vi "Measurement UI.vi"() -> ()   [LabVIEW 2024, in "Device Power Sequencer UI.lvlib"]
doc: "This module lets user configure a sequence to power up or power down any device. \n\nThe various configuration operations allowed are:\n1. Add Pin - Add a pin to the sequence\n2.Delete Pin - Delete a pin from the sequence\n3.Move Pin Up - Move the selected pin a level up in the sequence\n4.Move Pin Down - Move the selected pin a level down in the sequence\n5.Edit Pin - Change pin mapping and edit the configuration paramters.\n\nThe results displayed after sequence execution are:\n1. Voltage Waveform - Displays voltage graph for each pin\n2.Current Waveform - Displays current graph for each pin"
uses:
  Device Power Sequencer UI.lvlib
  Device Power Sequencer/controls/Source Pin Config.ctl
  Device Power Sequencer/controls/Source Mode.ctl
  Device Power Sequencer/controls/UI_Relative To.ctl
  Device Power Sequencer/controls/Sense Mode.ctl
  Device Power Sequencer/controls/Transient Response.ctl
  Device Power Sequencer/controls/Relative To.ctl
  Device Power Sequencer/controls/Plot Colors.ctl
  Device Power Sequencer/controls/Empty Plot Legend.ctl
  Device Power Sequencer/controls/Power line frequency.ctl
  Device Power Sequencer/controls/Plot Legend.ctl
  Device Power Sequencer/controls/Plot Cluster.ctl
  Device Power Sequencer/Device Power Sequencer.lvlib
panel:
  in  "Monitor":bool
  out "Pin Readbacks":string="      Pin readbacks"
  in  "Legend":T1
  in  "Empty Legend":T2={"Free label"="", "Header"="  Plot visibility", "Msg"="  No active channels"}
  out "Voltage":waveform(dbl)[](graph) caption="Voltage Measurements"
  out "Current":waveform(dbl)[](graph) caption="Current Measurements"
  in  "PD-Image":bool
  in  "Power Down Info":bool
  in  "Power Down":bool caption="Quick Power Down"
  out "Power Up/Down":bool
  in  "R-Image":bool
  in  "Pin Selection":i32(listbox)
  in  "Hover icon":bool
  in  "Selection icon":bool
  in  "Source Pin Seq":i32(listbox)
  out "Border":string
  in  "Move Down":bool
  in  "Move Up":bool
  in  "Remove":bool
  in  "Add":bool
  out "Error Header":string="Errors"
  out "Error":bool
  in  "Settings":bool
  in  "Reorder Hover Icon":bool
  out "Error Display":i32(listbox)
  out "Color Array":T3
  in  "Scrollbar":i32(c297)
  in  "Tab":T4(tab)
  in  "Info":bool
  in  "Pin Config":T5={"Pin"="Pin A", "MODE"="", "TARGET VALUE"=0.0, "RAMP RATE"=0.0, "COMPLIANCE LIMIT"=0.0, "START DELAY"=0.0, "Source Mode"=0, "RELATIVE TO"=enum."Power sequence start", "DEFAULT RAMP RATE"=FALSE, "SENSE MODE"=0, "Sense Mode Frame"="", "TRANSIENT RESPONSE"=0, "Transient Reponse Frame"="", "START VALUE"=0.0} {"START VALUE" min=-200.0 max=200.0 format="%_6p V"; "SENSE MODE" items=["Local", "Remote"]; "START DELAY" min=0.0 max=20.0 format="%_6p s"; "RAMP RATE" min=0.0 max=1.0 format="%_6p V/us"; "COMPLIANCE LIMIT" min=0.0 max=3.0 format="%_6p A"; "TARGET VALUE" min=-200.0 max=200.0 format="%_6p V"; "Source Mode" items=["DC Voltage", "DC Current"]; "TRANSIENT RESPONSE" items=["Slow", "Normal", "Fast"]}
  in  "PN AutoFit":string
  in  "Start Delay":dbl[](array[numeric]) format="%#_6p"
  in  "Start Value":dbl[](array[numeric]) format="%#_6p"
  in  "Relative To":T10[](array[typedef]) items=["Power sequence start", "Previous source start", "Previous source end"]
  in  "Pin Name":string[](array[combo])
  in  "Ramp Rate":dbl[](array[numeric]) format="%#_6p"
  in  "Compliance Limit":dbl[](array[numeric]) format="%#_6p"
  in  "Source Mode":T6[](array[typedef]) items=["Voltage", "Current"]
  in  "Target Value":dbl[](array[numeric]) format="%#_6p"
  in  "Data Capture":bool
  in  "Power line frequency":T11 items=["50 Hz", "60 Hz"]
  in  "Quick Power Down":bool
  in  "Default Ramp Rate":bool[](array[boolean])
  in  "Sense Mode":T8[](array[typedef]) items=["Local", "Remote"]
  in  "Transient Response":T9[](array[typedef]) items=["Slow", "Normal", "Fast"]
  out "Indices":i32[](array[numeric])
  out "Actual Ramp Rates":dbl[](array[numeric])
  out "dt values":dbl[](array[numeric])
  out "Current Measurements":dbl[](array[numeric])
  out "Voltage Measurements":dbl[](array[numeric])
  out "Default Ramp Rate?":bool[](array[boolean])
  out "Warning":string[](array[string])
  out "Operation Complete?":bool
  # "Source Pins"
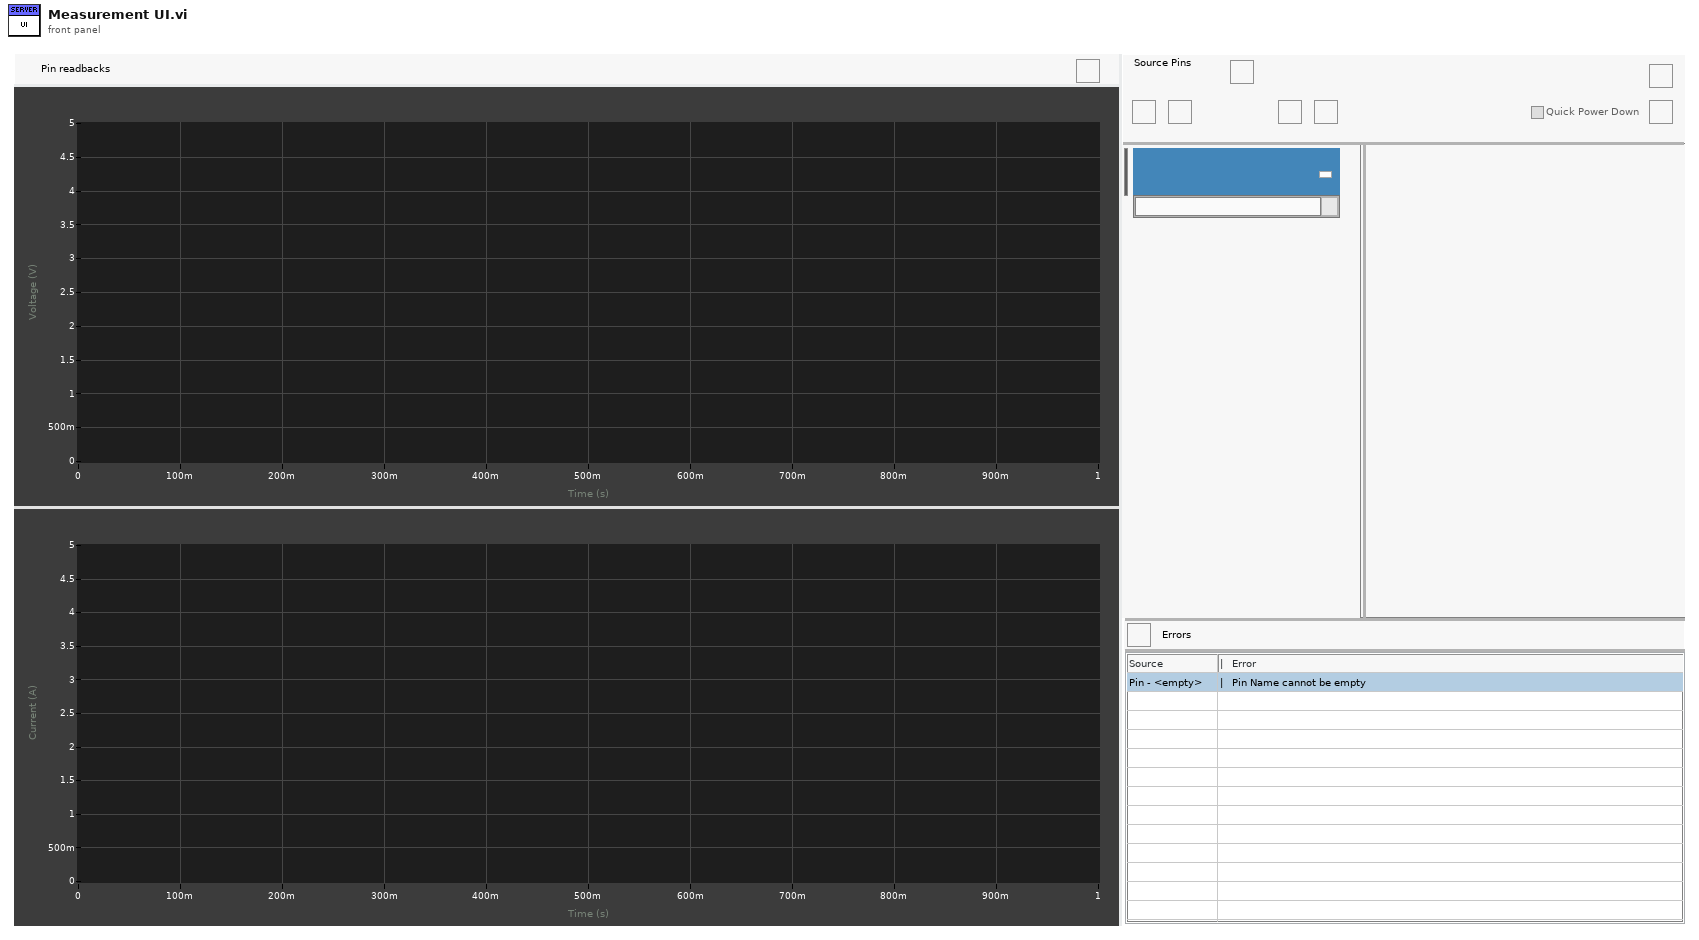
[diagram p1: front panel]
types:
  T1 = cluster{"Free label":string, "Voltage (V)":cluster{"Color":u32, "Name":string, "Visible":bool}[], "Current (A)":cluster{"Color":u32, "Name":string, "Visible":bool}[]}
  T2 = typedef "Device Power Sequencer.lvlib/Empty Plot Legend.ctl" = cluster{"Free label":string, "Header":string, "Msg":string}
  T3 = typedef "Device Power Sequencer.lvlib/Plot Colors.ctl" = u32[]
  T4 = enum32{"Default", "Config", "Hidden Ctl", "ML Ctl", "ML Ctl 2", "ML Results 1"}
  T5 = typedef "Device Power Sequencer.lvlib/Source Pin Config.ctl" = cluster{"Pin":string, "MODE":string, "TARGET VALUE":dbl, "RAMP RATE":dbl, "COMPLIANCE LIMIT":dbl, "START DELAY":dbl, "Source Mode":T6, "RELATIVE TO":T7, "DEFAULT RAMP RATE":bool, "SENSE MODE":T8, "Sense Mode Frame":string, "TRANSIENT RESPONSE":T9, "Transient Reponse Frame":string, "START VALUE":dbl}
  T6 = typedef "Device Power Sequencer.lvlib/Source Mode.ctl" = i32
  T7 = typedef "Device Power Sequencer.lvlib/UI_Relative To.ctl" = enum32{"Power sequence start", "Previous source start", "Previous source end"}
  T8 = typedef "Device Power Sequencer.lvlib/Sense Mode.ctl" = i32
  T9 = typedef "Device Power Sequencer.lvlib/Transient Response.ctl" = i32
  T10 = typedef "Device Power Sequencer.lvlib/Relative To.ctl" = u32
  T11 = typedef "Device Power Sequencer.lvlib/Power line frequency.ctl" = u32
  T12 = typedef "Device Power Sequencer.lvlib/Plot Legend.ctl" = cluster{"Free label":string, "Voltage (V)":T13[], "Current (A)":T13[]}
  T13 = typedef "Device Power Sequencer.lvlib/Plot Cluster.ctl" = cluster{"Color":u32, "Name":string, "Visible":bool}
  T14 = cluster{"#Rows":u32, "List Specs":cluster{"Active Row Nos":u32[], "CellBG":u32[], "Cell Height":i32[], "UI Pin List":string[], "Pin List":string[]}, "Pinmap List":string[], "Action":string, "Pins":string[], "Scrollbar":cluster{"DocMax":u32, "New Val":i32, "Old Val":i32, "Action":enum16{"None", "Up", "Down"}}, "Pin Selection":cluster{"Selection Coords":cluster{"Horizontal":i32, "Vertical":i32}, "Dimensions":cluster{"Width":i32, "Left":i32, "Height":i32, "Top":i32}}, "Coords":cluster{"Selection Coords":cluster{"Horizontal":i32, "Vertical":i32}, "Hover Coords":cluster{"Horizontal":i32, "Vertical":i32}, "List Coords":cluster{"Icon Left":i32, "Icon Top Offset":i32, "Reorder Icon Left":i32, "Reorder Icon Top Offset":i32}, "Mouse Coords":cluster{"Horizontal":i32, "Vertical":i32}, "Border Left":i32, "Active Row Pos":cluster{"Left":i32, "Top":i32}, "Source Pin Seq":cluster{"Width":i32, "Left":i32, "Height":i32, "Top":i32}, "Selection Icon":cluster{"Width":i32, "Left":i32, "Height":i32, "Top":i32}, "Info Icon":cluster{"Width":i32, "Left":i32, "Height":i32, "Top":i32}, "Plot Legend":cluster{"Width":i32, "Left":i32, "Height":i32, "Top":i32}, "Monitor":cluster{"Width":i32, "Left":i32, "Height":i32, "Top":i32, "Right":i32}, "Empty Legend":cluster{"Width":i32, "Left":i32, "Height":i32, "Top":i32}, "Error Display":cluster{"Width":i32, "Left":i32, "Height":i32, "Top":i32}, "Hover Coords Old":cluster{"Horizontal":i32, "Vertical":i32}, "Graph Size":cluster{"Width":u32, "Height":u32}, "Reorder Hover Icon":cluster{"Width":i32, "Left":i32, "Height":i32, "Top":i32}, "PDInfo Icon":cluster{"Width":i32, "Left":i32, "Height":i32, "Top":i32}}, "Indices":cluster{"Active Row":i32, "Last Active Row":i32, "Pin Change":i32, "Row No Ref":u32, "Selected Row":i32, "NumRows":u32, "Top Row":u32, "Actual Sel Row":i32, "Pin Len \nold":i32, "Pin Len new":i32, "Pin Len Ind":i32, "No.Errors":i32, "Error Db Clk Row":i32, "Edit Pin Row":i32}, "Seq Reorder":cluster{"Drag Ind":i32, "Drop Ind":i32, "Drag?":bool, "Up?":bool}, "Pin Config":cluster{"Source Pin Config":T5[], "Active Pin Config":T5, "Power Up/Down":bool, "Color Array":T3, "ML Config":cluster{"Power Down":bool, "Pin Name":string[], "Source Mode":T6[], "Start Value":dbl[], "Target Value":dbl[], "Compliance Limit":dbl[], "Sense Mode":T8[], "Default Ramp Rate":bool[], "Ramp Rate":dbl[], "Start Delay":dbl[], "Relative To":T10[], "Transient Response":T9[], "Data Capture":bool, "Power line frequency":T11}, "Error Info":string[], "Overall Errors":string, "Error Ind":i32[]}, "Flags":cluster{"Same Hover Row?":bool, "Visibilty":cluster{"Hover Icon":bool, "Selection Icon":bool, "Pin Selection List":bool, "Border":bool, "Scrollbar?":bool, "Help?":bool, "Plot Legend":bool, "Plot Legend Scrollbar":bool, "Settings Icon":bool, "Reorder Hover Icon":bool, "PD Info":bool}, "Mouse Move In Source Pin Seq?":bool, "Mouse Down In Source Pin Seq?":bool, "Changes?":bool, "Same Size?":bool, "UI State":enum8{"Enabled", "Disabled", "Disabled and Grayed Out"}, "Check All?":bool, "Color Errors?":bool, "Adv Settings Change?":bool, "P.up Success?":bool}, "All Refs":refnum<vi>[], "Error Map":map{i32, string}, "Legend":T12, "Plot Colors":u32[], "Pin Symbols":i32[], "Adv Settings":cluster{"Setting.Sel":cluster{"Main":string[], "PL_Freq":string[]}, "Adv Setting":cluster{"Power line frequency":T11, "Data Capture":bool}, "Item Tag":string}, "Ref Colors":u32[]}
  T15 = typedef "LVRectTypeDef.ctl" = cluster{"Left":i16, "Top":i16, "Right":i16, "Bottom":i16}
  T16 = typedef "LVPoint32TypeDef.ctl" = cluster{"Horizontal":i32, "Vertical":i32}
  T17 = cluster{"Color":u32, "Name":string, "Visible":bool}[]
  T18 = cluster{"Pin":bool, "MODE":bool, "TARGET VALUE":bool, "RAMP RATE":bool, "COMPLIANCE LIMIT":bool, "START DELAY":bool, "Source Mode":bool, "RELATIVE TO":bool, "DEFAULT RAMP RATE":bool, "SENSE MODE":bool, "Sense Mode Frame":bool, "TRANSIENT RESPONSE":bool, "Transient Reponse Frame":bool, "START VALUE":bool}
  T19 = typedef "LVBoundsTypeDef.ctl" = cluster{"Width":u32, "Height":u32}
  T20 = enum8{"Enabled", "Disabled", "Disabled and Grayed Out"}
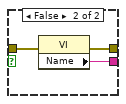
[diagram p2: hidden frame]
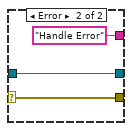
[diagram p3: hidden frame]
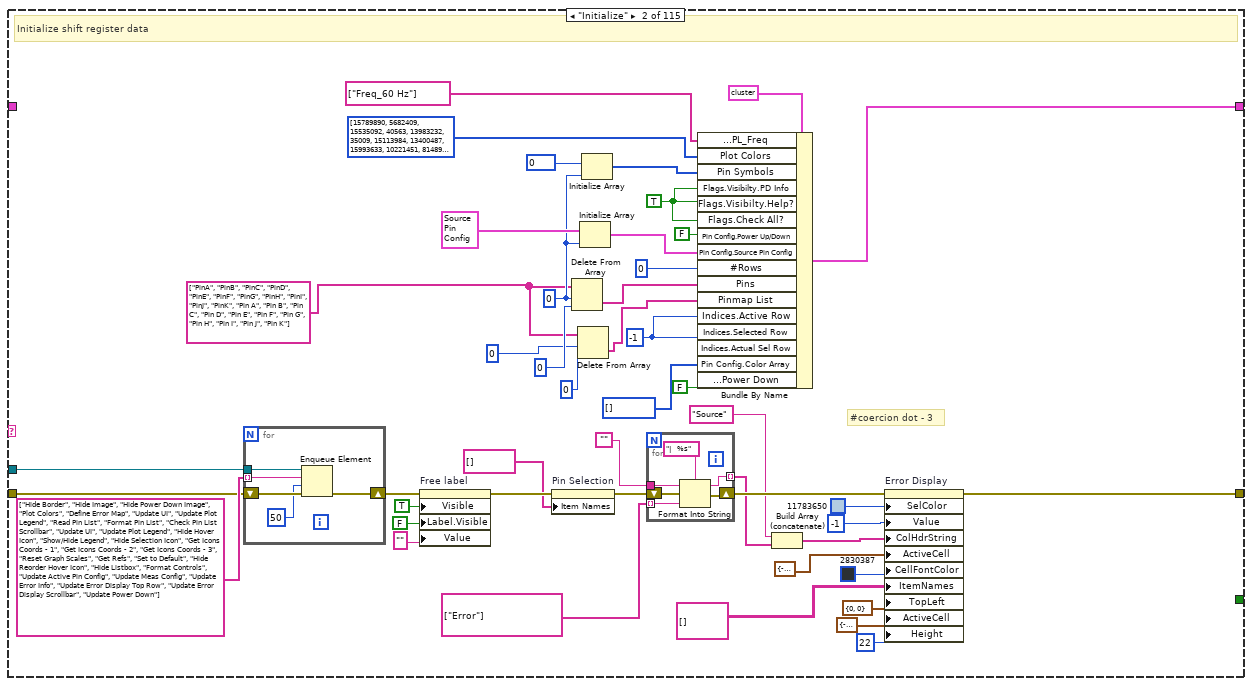
[diagram p5: hidden frame]
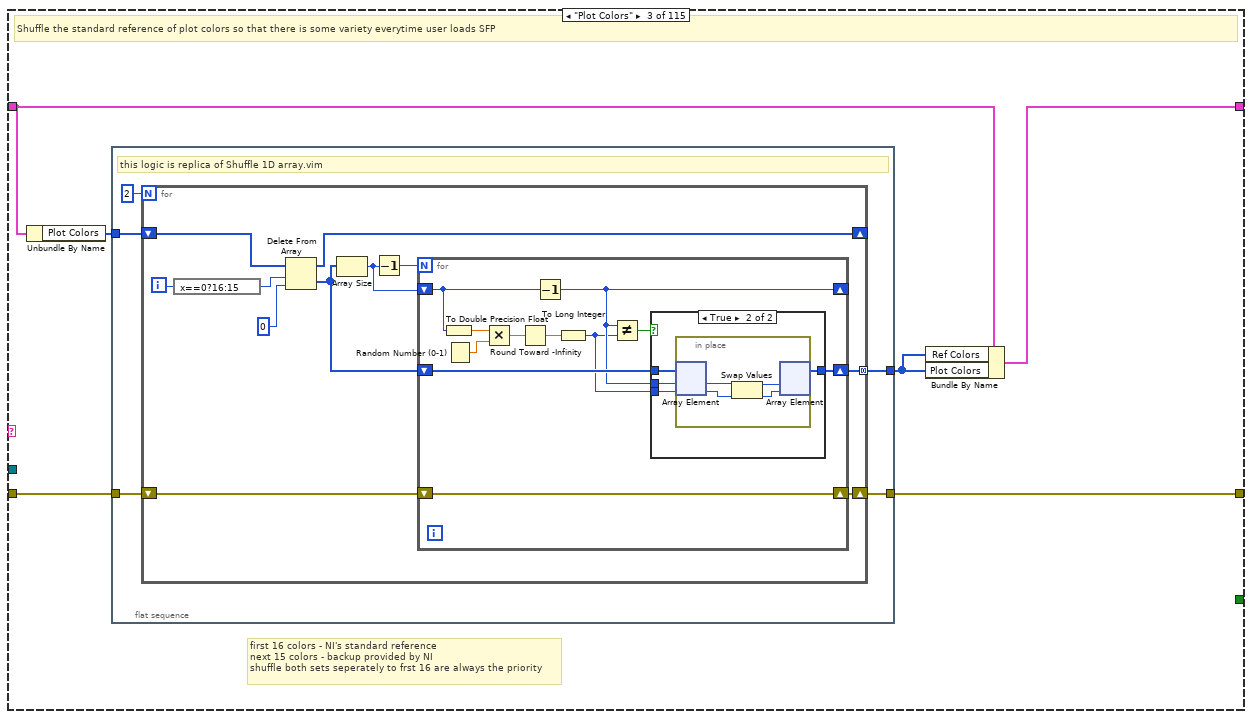
[diagram p6: hidden frame]
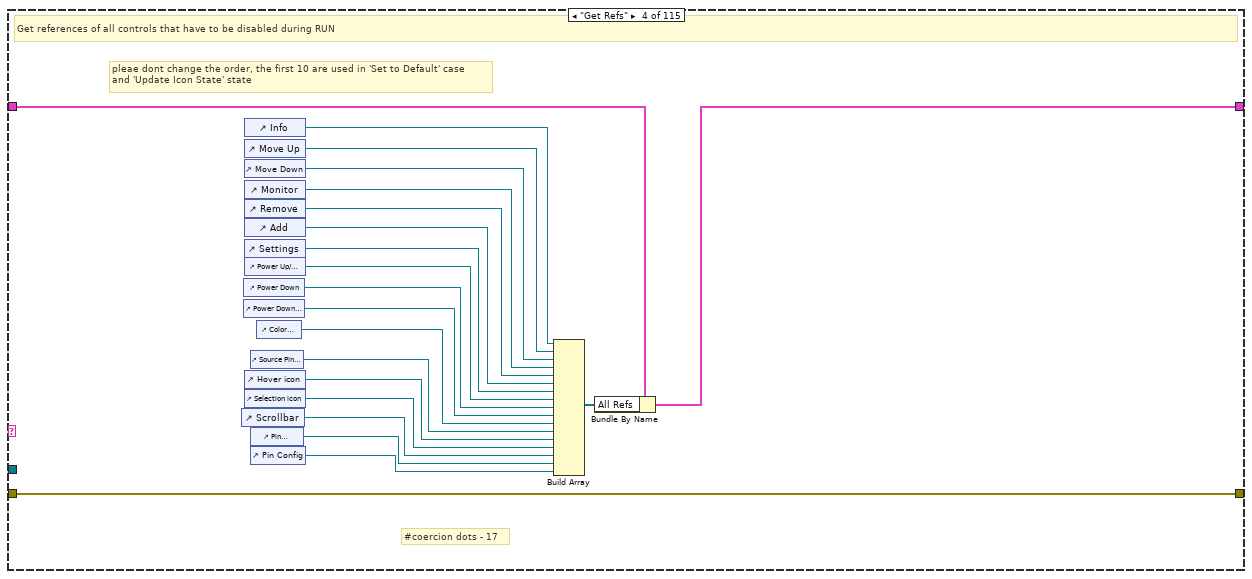
[diagram p8: hidden frame]
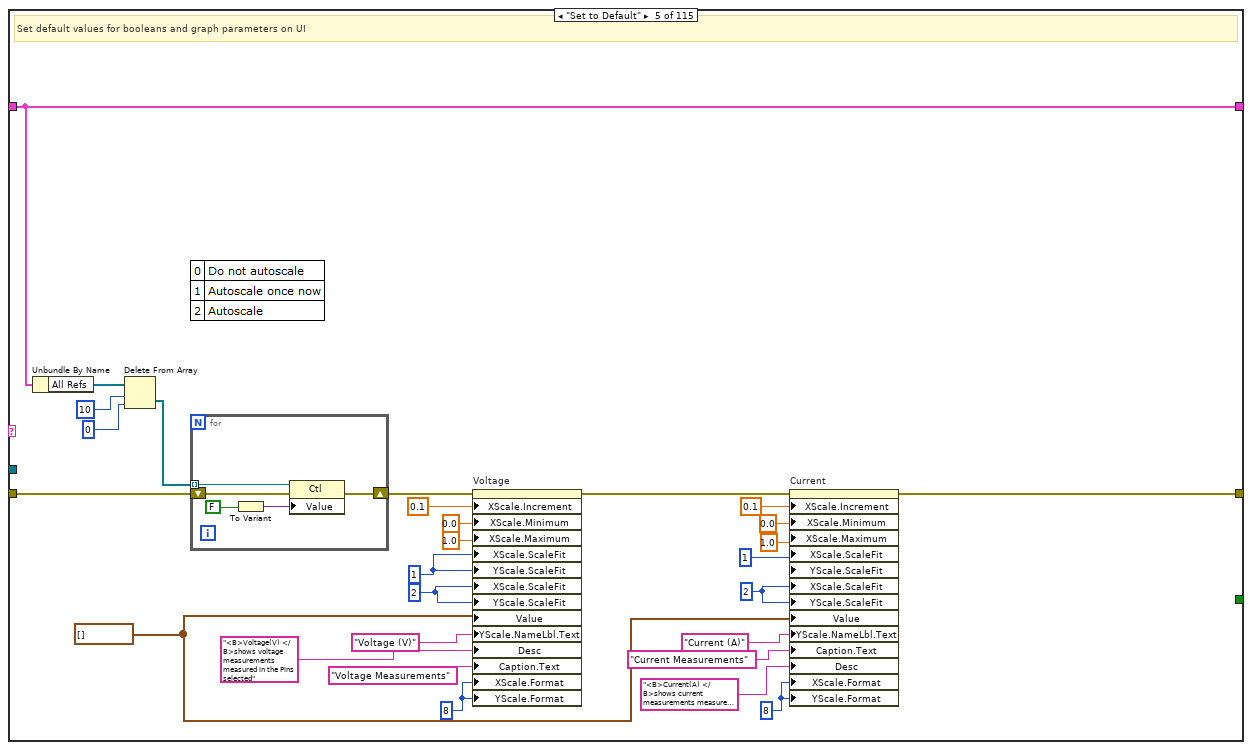
[diagram p9: hidden frame]
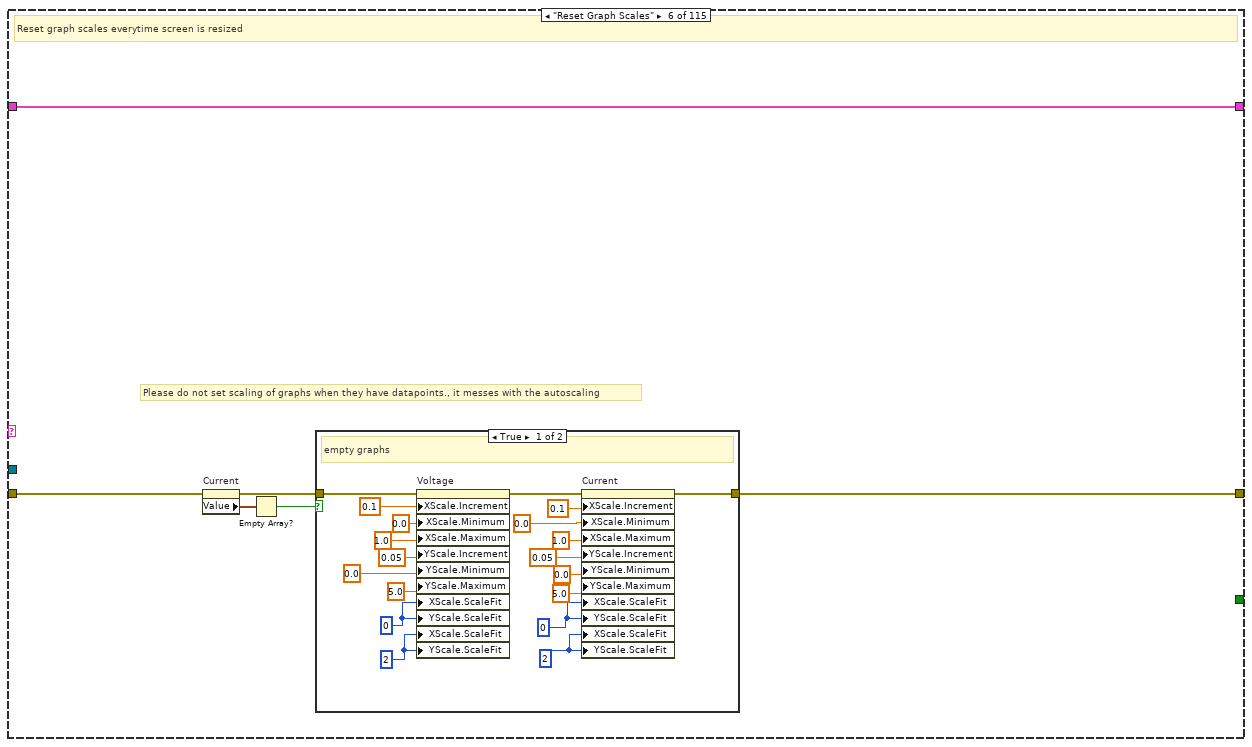
[diagram p10: hidden frame]
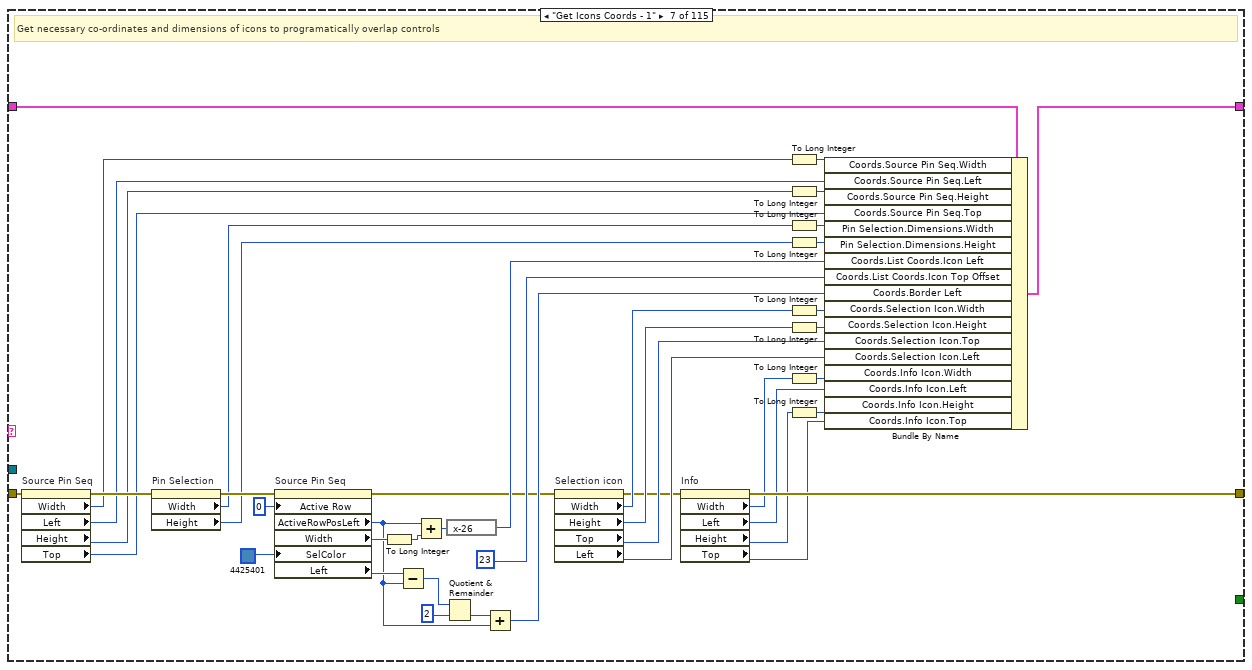
[diagram p12: hidden frame]
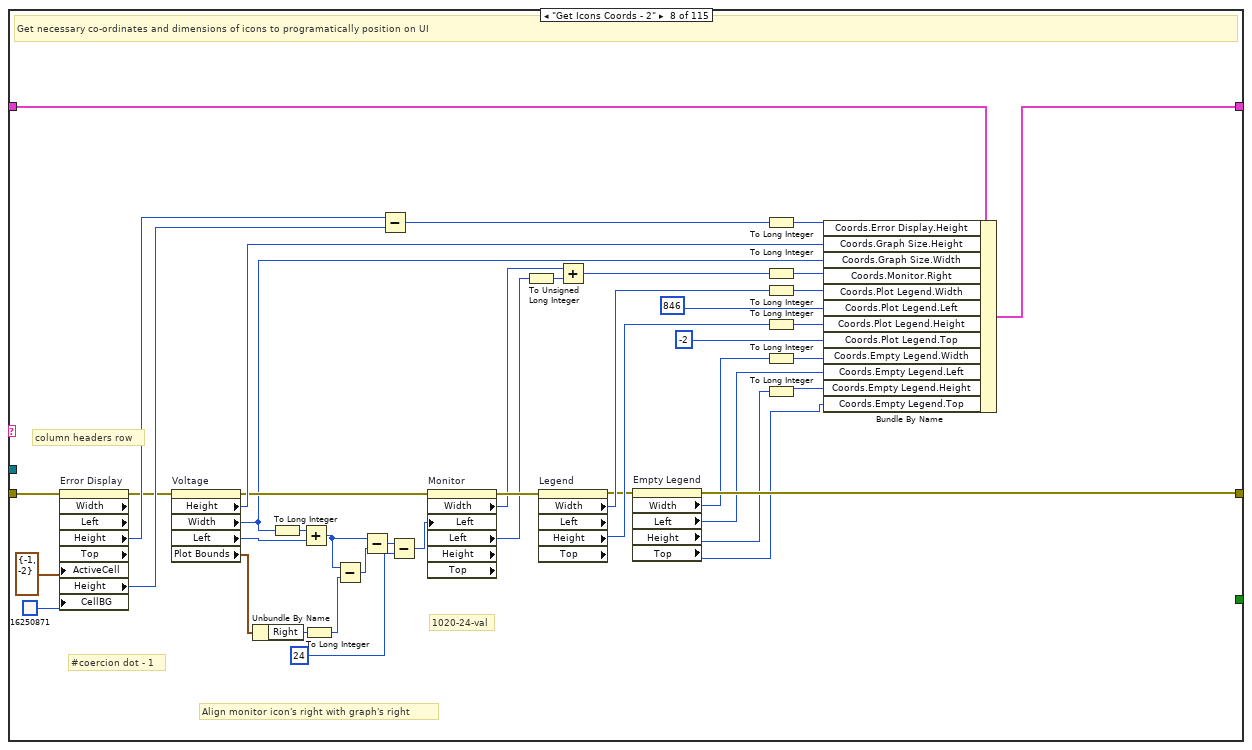
[diagram p13: hidden frame]
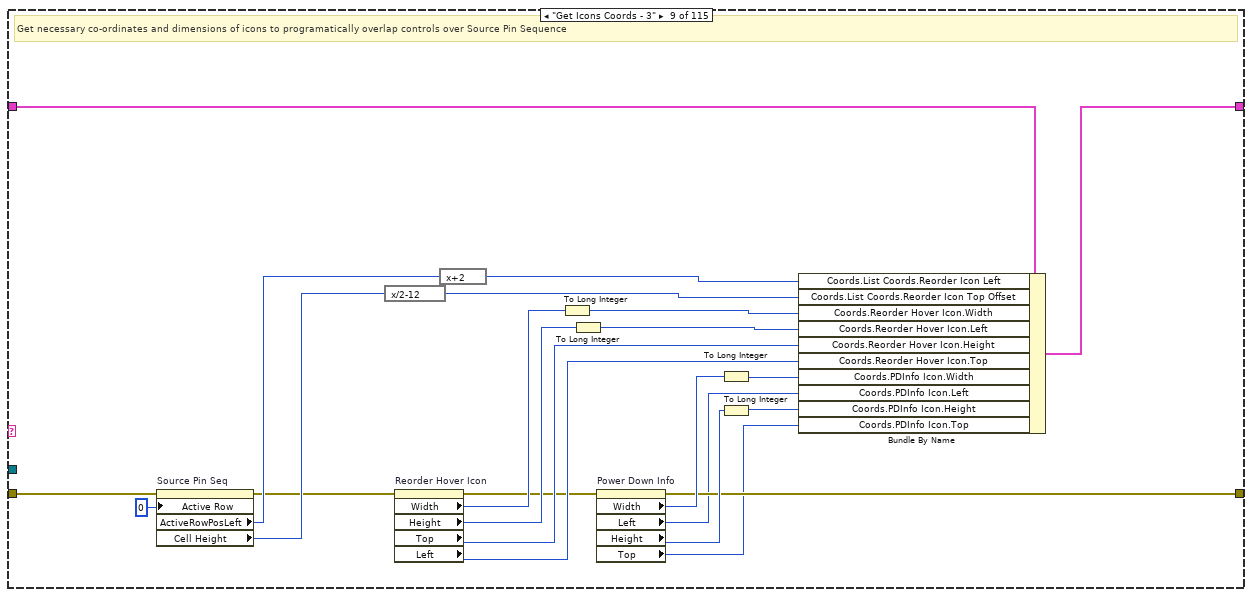
[diagram p14: hidden frame]
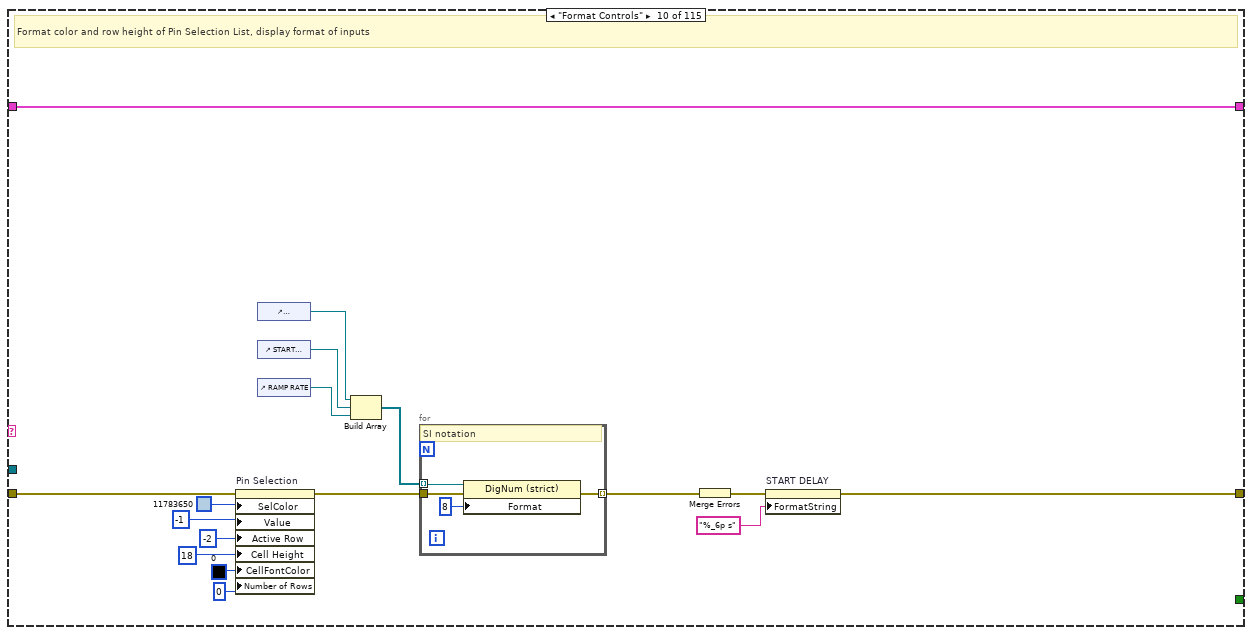
[diagram p15: hidden frame]
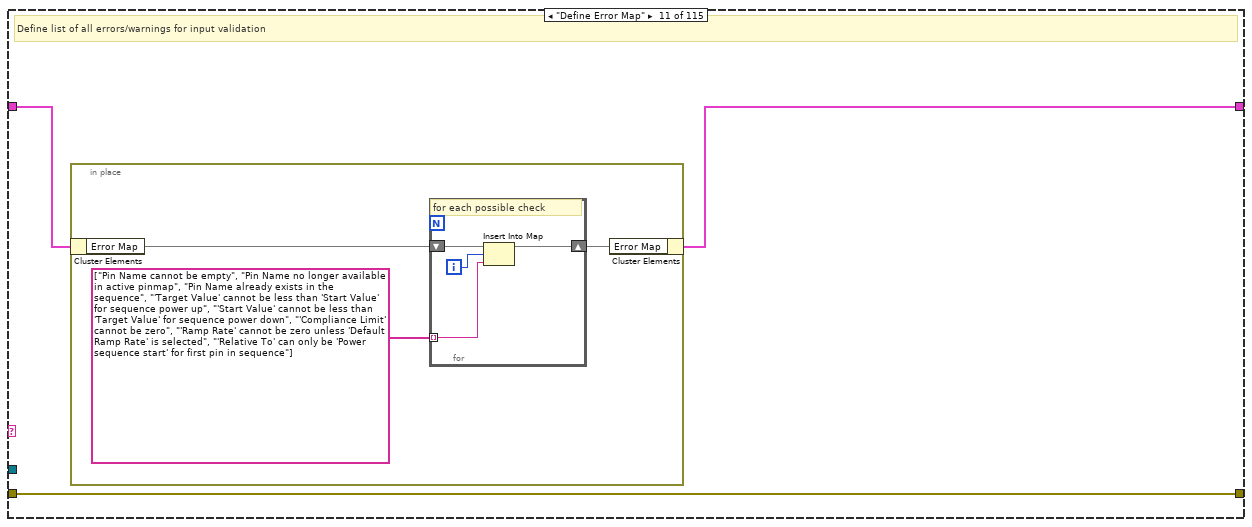
[diagram p16: hidden frame]
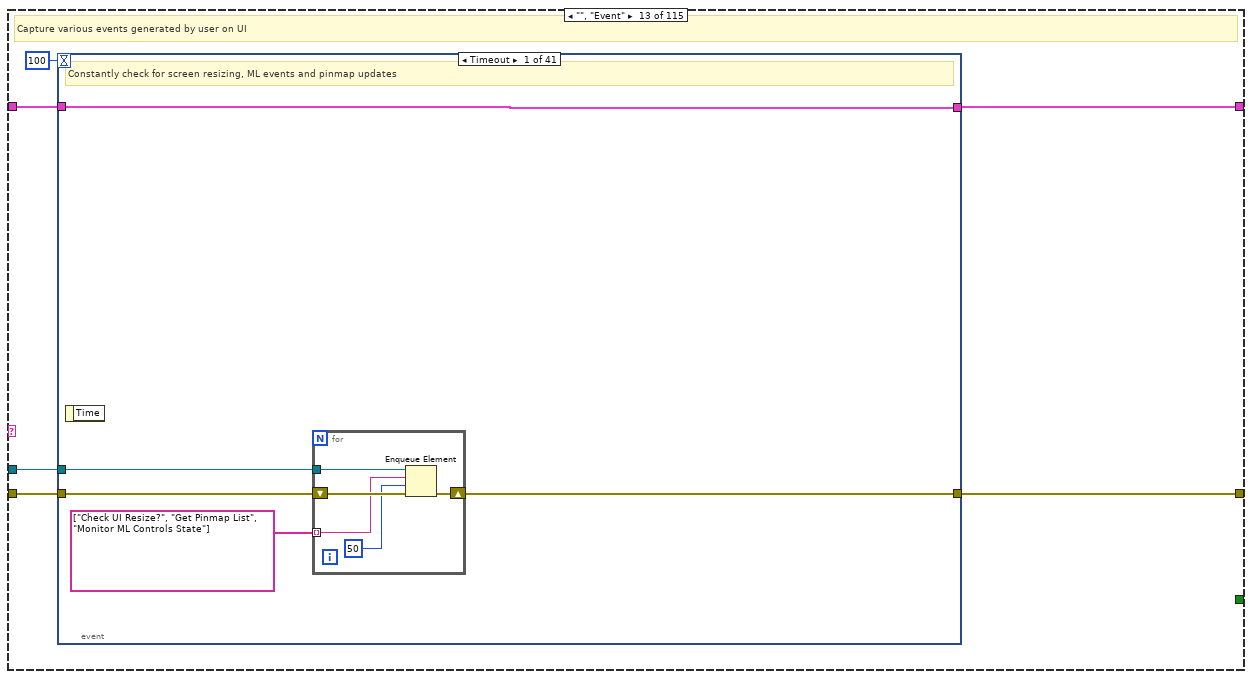
[diagram p18: hidden frame]
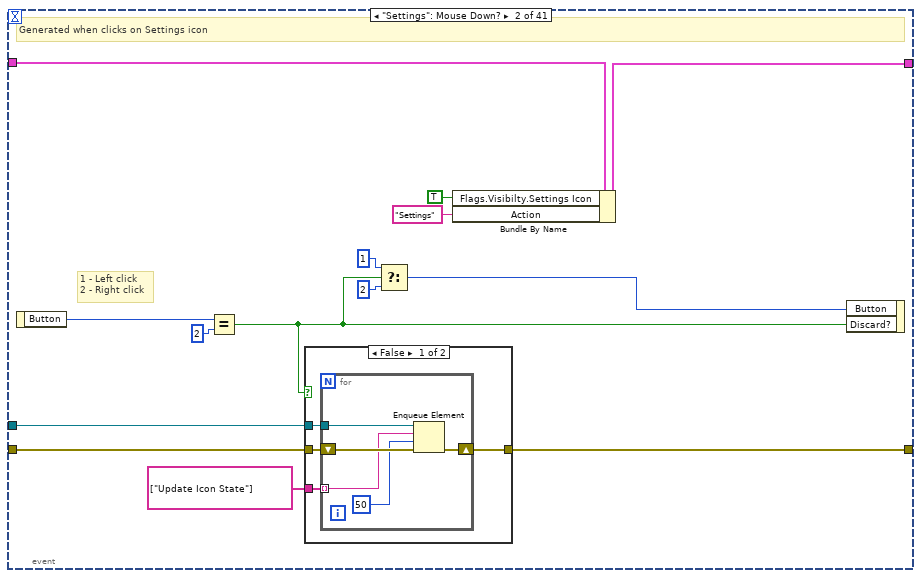
[diagram p19: hidden frame]
diagram:
  # "Notes - \n- For coercion dots check bookmark #coercion\n   there are 48 instances - either from invoke/property nodes for lv typedefs (or) project\n   typedefs (or) control references' arrays (Except control references' arrays, other       instances are from lv typedefs from vi.lib which MeasLink does not support\n- All measurement link controls and indicators are hidden in Tab control pages"
  # "NOTE:\n- 'Legend' and its controls should NOT be typedefs \n- Graphs CANNOT be typedefs (Graph.ctl). Does not work with scale objects with pane\n- Ensure Pin Readbacks string indicator (in DISABLED state)\n     and decoration strip are grouped and of same size as the pane itself.\n- DO NOT modify Pin Readbacks strip's both value/default value.\n-  power line frequency value upon sfp launch is 60 Hz by default. Please set 60 Hz as DEFAULT value in Measurement Configuration.ctl\n- The label for Quick Power Down on UI top right is kept 'Power Down' and caption is visible - 'Quick Power Down'. Please DO NOT change this as MeasLink will consider this as its control and start enable/disbale it during run."
  # "Instructions:\n-Avoid coercion dots\n-Do not use any functions/controls from vi.lib\n  (Ex: Trim Whitespaces, Coords cluster in mouse events,\n   Error Handler VIs, RGB to color)\n- Do not use any booleans in latch mode\n- Do not pass any references to SubVIs"
  # "Measurement Link Results"
  # "12 px - 15 pt in labview\n10 px - 12 pt in labview"
  # "#MeasurementToDo  \n\nAdd the User Interface controls and Indicator to the Front Panel of this VI. The control and indicator label name should match the name of the `Measurement Configuration` and `Measurement Results` data.\n\nNote:  If user interface needs to have UI logic that post process the `Measurement Results` to display more information, `Post UI Update` case can be used to post process the results from `Measurement Results` Indicator and update them again. This case will be invoked by InstrumentStudio G Plugin after the UI is updated with Measurement Results."
  n1 = property on="Property Node" class="VI"() -> (error out=w1:errorcluster, "IsCloneVI"=w2:bool)  [unwired: 2 in, 1 out]
  n2 = case shown="True" w2 {
    tunnel: [w13 w16] -> w10
    tunnel: [w12 w15] -> w9
    tunnel: w1 -> [w11 w14]
    frame True {
      n3 = property on="Property Node" class="VI"(error in=w11) -> (error out=w13:errorcluster, "Clone Name"=w12:string)  [unwired: 1 in, 1 out]
    }
    frame False {
      n4 = property on="Property Node" class="VI"(error in=w14) -> (error out=w16:errorcluster, "Name"=w15:string)  [unwired: 1 in, 1 out]
    }
  }
  n5 = Obtain Queue(name (unnamed)=w9, element data type="" ("Empty String Constant"), error in (no error)=w10) -> (queue out=w6:refnum<queue>, error out=w8:errorcluster)  [unwired: 2 in, 1 out]
  n6 = Enqueue Element(queue=w6, element="Initialize", error in (no error)=w8) -> (queue out=w5:refnum<queue>, error out=w7:errorcluster)  [unwired: 1 in, 1 out]
  n7 = while {
    shift-right: [w21] -> _
    shift-left: w7 -> [w25]
    tunnel: w5 -> [w23]
    shift-right: [w17] -> _
    shift-left: _ -> [w19]
    stop <- w20 stop-if-true
    # "Device Power Sequencing Module - UI Operations"
    n8 = case shown="No Error" w25 {
      selector: w25 -> [w31 w34]
      tunnel: [w30 w34] -> w24
      tunnel: w23 -> [w29 w33]
      tunnel: [w28 w33] -> w22
      tunnel: [w27 "Handle Error"] -> w18
      frame No Error {
        n9 = Dequeue Element(queue=w29, timeout in ms (-1)=100, error in (no error)=w31) -> (queue out=w28:refnum<queue>, element=w27:string, error out=w30:errorcluster)  [unwired: 1 out]
      }
      frame Error {
      }
    }
    n10 = case shown="\"Read Pin List\"" w18 {
      tunnel: w24 -> [w36 w79 w99 w156 w180 w194 w248 w274 w315 w330 w348 w357 w362 w853 w863 w878 w912 w914 w970 w972 w977 w1003 w1036 w1074 w1115 w1155 w1166 w1181 w1187 w1189 w1214 w1269 w1282 w1286 w1291 w1311 w1329 w1347 w1362 w1389 w1419 w1426 w1437 w1483 w1521 w1548 w1580 w1626 w1644 w1660 w1662 w1707 w1745 w1768 w1771 w1812 w1814 w1831 w1856 w1859 w1872 w1889 w1957 w1975 w1993 w2000 w2007 w2015 w2021 w2032 w2040 w2047 w2053 w2069 w2100 w2108 w2148 w2165 w2182 w2216 w2255 w2266 w2300 w2356 w2409 w2445 w2460 w2560 w2616 w2653 w2660 w2694 w2700 w2722 w2746 w2751 w2762 w2784 w2803 w2836 w2843 w2860 w2870 w2955 w2972 w2986 w3029 w3073 w3105 w3169 w3181 w3205 _ w3209 w3217]
      tunnel: w22 -> [_ w82 _ _ _ _ _ _ _ _ _ _ w360 _ w862 w891 _ _ _ _ _ w1002 w1035 w1073 w1114 _ w1165 _ _ _ _ _ _ _ w1288 _ w1328 w1346 _ _ _ _ w1441 _ _ w1547 _ _ _ _ w1664 _ w1741 _ _ _ _ w1820 _ _ w1870 w1886 _ _ _ _ _ _ _ _ _ _ _ _ _ _ _ _ _ _ _ _ _ _ _ _ _ _ _ _ _ _ _ _ _ w2749 _ _ _ _ w2842 _ _ w2954 _ w2988 w3018 w3072 _ _ w3189 _ _ _ w3215]
      tunnel: [w36 w65 w98 w156 w170 w193 w222 w287 w306 w326 w348 w357 w363 w853 w861 w885 w912 w913 w970 w972 w977 w1004 w1037 w1075 w1116 w1155 w1167 w1181 w1187 w1189 w1198 w1270 w1283 w1286 w1287 w1302 w1330 w1345 w1368 w1396 w1419 w1426 w1442 w1486 w1522 w1546 w1586 w1626 w1643 w1660 w1665 w1707 w1742 w1768 w1771 w1812 w1814 w1819 w1856 w1859 w1871 w1888 w1957 w1975 w1993 w1999 w2006 w2014 w2018 w2031 w2039 w2046 w2049 w2064 w2099 w2107 w2141 w2160 w2168 w2212 w2261 w2270 w2300 w2341 w2409 w2445 w2459 w2572 w2615 w2652 w2666 w2696 w2697 w2724 w2746 w2748 w2760 w2784 w2786 w2836 w2841 w2860 w2869 w2953 w2972 w2987 w3024 w3071 errorcluster {"status"=FALSE, "code"=0, "source"=""} ("error out") w3167 w3191 w3205 w3206 w3209 w3212] -> w21
      tunnel: [_ _ _ _ _ _ _ _ _ _ _ _ _ _ _ _ _ _ _ _ _ _ _ _ _ _ _ _ _ _ _ _ _ _ _ _ _ _ _ _ _ _ _ _ _ _ _ _ _ _ _ _ _ _ _ _ _ _ _ _ _ _ _ _ _ _ _ _ _ _ _ _ _ _ _ _ _ _ _ _ _ _ _ _ _ _ _ _ _ _ _ _ _ _ _ _ _ _ _ _ _ _ _ _ _ _ _ _ _ _ _ _ _ _ TRUE] -> w20
      tunnel: w19 -> [w35 _ w97 w155 w184 w195 w258 w301 w324 w341 w347 w356 w359 w852 w860 w884 w911 w920 w969 w971 w976 w991 w1026 w1064 w1106 w1154 w1164 w1180 w1186 w1188 w1196 w1271 w1284 w1285 w1290 w1309 w1322 w1344 w1367 w1395 w1418 w1425 w1440 w1485 w1518 w1545 w1585 w1625 w1650 w1661 w1671 w1711 w1747 w1770 w1772 w1807 w1813 w1834 w1857 w1858 w1874 w1895 w1956 w1974 w1994 w2001 w2008 w2016 w2020 w2033 w2041 w2044 w2051 w2068 w2098 w2137 w2157 w2161 w2185 w2213 w2262 w2274 w2287 w2379 w2415 w2444 w2465 w2571 w2614 w2649 w2667 w2693 w2701 w2725 w2745 w2747 w2761 w2783 w2804 w2831 w2840 w2859 w2867 w2952 w2971 w2989 w3028 w3076 w3101 w3163 w3192 w3204 w3207 w3208 w3210]
      tunnel: [w35 w78 w96 w154 w184 w195 w255 w300 w323 w341 w346 w356 w358 w852 w860 w883 w911 w917 w969 w971 w974 w991 w1024 w1062 w1104 w1153 w1158 w1180 w1185 w1188 w1212 w1271 w1284 w1285 w1290 w1310 w1327 w1344 w1366 w1394 w1418 w1422 w1439 w1484 w1520 w1545 w1584 w1625 w1648 w1661 w1671 w1709 w1746 w1769 w1772 w1811 w1813 w1833 w1852 w1858 w1866 w1894 w1955 w1973 w1994 w1996 w2003 w2011 w2020 w2028 w2035 w2042 w2050 w2056 w2098 w2124 w2156 w2161 w2171 w2213 w2256 w2273 w2286 w2376 w2414 w2444 w2461 w2571 w2614 w2651 w2663 w2692 w2701 w2723 w2745 w2747 w2759 w2783 w2805 w2830 w2840 w2857 w2866 w2957 w2971 w2978 w3023 w3076 w3099 w3161 w3190 w3204 w3207 w3208 w3210] -> w17
      frame "--- Initializations ----" {
      }
      frame "Initialize" {
        w38 = TRUE ("Pin Config.Power Up?")
        w50 = 0 ("length")
        w44 = string[] ["PinA", "PinB", "PinC", "PinD", "PinE", "PinF", "PinG", "PinH", "PinI", "PinJ", "PinK", "Pin A", "Pin B", "Pin C", "Pin D", "Pin E", "Pin F", "Pin G", "Pin H", "Pin I", "Pin J", "Pin K"]
        w70 = -1 ("Selected Row")
        # "#coercion dot - 3"
        # "Initialize shift register data"
        n11 = for {
          shift-right: [w92] -> w68
          shift-left: w79 -> [w93]
          tunnel: w82 -> [w91]
          tunnel: string[] ["Hide Border", "Hide Image", "Hide Power Down Image", "Plot Colors", "Define Error Map", "Update UI", "Update Plot Legend", "Read Pin List", "Format Pin List", "Check Pin List Scrollbar", "Update UI", "Update Plot Legend", "Hide Hover Icon", "Show/Hide Legend", "Hide Selection Icon", "Get Icons Coords - 1", "Get Icons Coords - 2", "Get Icons Coords - 3", "Reset Graph Scales", "Get Refs", "Set to Default", "Hide Reorder Hover Icon", "Hide Listbox", "Format Controls", "Update Active Pin Config", "Update Meas Config", "Update Error Info", "Update Error Display Top Row", "Update Error Display Scrollbar", "Update Power Down"] -> [w90] mode=indexing
          n12 = Enqueue Element(queue=w91, element=w90, timeout in ms (-1)=50, error in (no error)=w93) -> (error out=w92:errorcluster)  [unwired: 2 out]
        }
        n13 = property on="Free label" class="Str"(error in=w68, "Visible"=TRUE, "Label.Visible"=FALSE ("Visible"), "Value"="" ("Label.Text")) -> (error out=w46:errorcluster)  [unwired: 1 in, 1 out]
        n14 = property on="Pin Selection" class="LstBox (strict)"(error in=w46, "Item Names"=string[] []) -> (error out=w45:errorcluster)  [unwired: 1 in, 1 out]
        n15 = Delete From Array(array=w44, length=w50, index=0) -> (deleted portion=w76:string[])  [unwired: 1 out]
        n16 = Delete From Array(array=w44, length=0, index=0) -> (deleted portion=w40:string[])  [unwired: 1 out]
        n17 = Initialize Array(T5 {"Pin"="", "MODE"="", "TARGET VALUE"=0.0, "RAMP RATE"=0.0, "COMPLIANCE LIMIT"=0.0, "START DELAY"=0.0, "Source Mode"=0, "RELATIVE TO"=enum."Power sequence start", "DEFAULT RAMP RATE"=FALSE, "SENSE MODE"=0, "Sense Mode Frame"="", "TRANSIENT RESPONSE"=0, "Transient Reponse Frame"="", "START VALUE"=0.0} ("Pin Config"), w50) -> (w74:T5[])
        n18 = Initialize Array(0, w50) -> (w51:i32[])
        n19 = for {
          tunnel: string[] ["Error"] -> [w86] mode=indexing
          tunnel: "" ("initial string") -> [w87]
          tunnel: [w88] -> w59 mode=indexing
          shift-right: [w84] -> w60
          shift-left: w45 -> [w85]
          n20 = Format Into String(format string="|   %s" ("initial string"), initial string=w87, error in=w85, w86) -> (resulting string=w88:string, error out=w84:errorcluster)
        }
        n21 = Bundle By Name(cluster=T14 {"#Rows"=0, "List Specs"={"Active Row Nos"=[], "CellBG"=[], "Cell Height"=[], "UI Pin List"=[], "Pin List"=[]}, "Pinmap List"=[], "Action"="", "Pins"=[], "Scrollbar"={"DocMax"=0, "New Val"=0, "Old Val"=0, "Action"=enum."None"}, "Pin Selection"={"Selection Coords"={"Horizontal"=0, "Vertical"=0}, "Dimensions"={"Width"=0, "Left"=0, "Height"=0, "Top"=0}}, "Coords"={"Selection Coords"={"Horizontal"=0, "Vertical"=0}, "Hover Coords"={"Horizontal"=0, "Vertical"=0}, "List Coords"={"Icon Left"=0, "Icon Top Offset"=0, "Reorder Icon Left"=0, "Reorder Icon Top Offset"=0}, "Mouse Coords"={"Horizontal"=0, "Vertical"=0}, "Border Left"=0, "Active Row Pos"={"Left"=0, "Top"=0}, "Source Pin Seq"={"Width"=0, "Left"=0, "Height"=0, "Top"=0}, "Selection Icon"={"Width"=0, "Left"=0, "Height"=0, "Top"=0}, "Info Icon"={"Width"=0, "Left"=0, "Height"=0, "Top"=0}, "Plot Legend"={"Width"=0, "Left"=0, "Height"=0, "Top"=0}, "Monitor"={"Width"=0, "Left"=0, "Height"=0, "Top"=0, "Right"=0}, "Empty Legend"={"Width"=0, "Left"=0, "Height"=0, "Top"=0}, "Error Display"={"Width"=0, "Left"=0, "Height"=0, "Top"=0}, "Hover Coords Old"={"Horizontal"=0, "Vertical"=0}, "Graph Size"={"Width"=0, "Height"=0}, "Reorder Hover Icon"={"Width"=0, "Left"=0, "Height"=0, "Top"=0}, "PDInfo Icon"={"Width"=0, "Left"=0, "Height"=0, "Top"=0}}, "Indices"={"Active Row"=0, "Last Active Row"=0, "Pin Change"=0, "Row No Ref"=0, "Selected Row"=0, "NumRows"=0, "Top Row"=0, "Actual Sel Row"=0, "Pin Len \nold"=0, "Pin Len new"=0, "Pin Len Ind"=0, "No.Errors"=0, "Error Db Clk Row"=0, "Edit Pin Row"=0}, "Seq Reorder"={"Drag Ind"=0, "Drop Ind"=0, "Drag?"=FALSE, "Up?"=FALSE}, "Pin Config"={"Source Pin Config"=[], "Active Pin Config"={"Pin"="Pin A", "MODE"="", "TARGET VALUE"=0.0, "RAMP RATE"=0.0, "COMPLIANCE LIMIT"=0.0, "START DELAY"=0.0, "Source Mode"=0, "RELATIVE TO"=enum."Power sequence start", "DEFAULT RAMP RATE"=FALSE, "SENSE MODE"=0, "Sense Mode Frame"="", "TRANSIENT RESPONSE"=0, "Transient Reponse Frame"="", "START VALUE"=0.0}, "Power Up/Down"=FALSE, "Color Array"=[], "ML Config"={"Power Down"=FALSE, "Pin Name"=[], "Source Mode"=[], "Start Value"=[], "Target Value"=[], "Compliance Limit"=[], "Sense Mode"=[], "Default Ramp Rate"=[], "Ramp Rate"=[], "Start Delay"=[], "Relative To"=[], "Transient Response"=[], "Data Capture"=TRUE, "Power line frequency"=0}, "Error Info"=[], "Overall Errors"="", "Error Ind"=[]}, "Flags"={"Same Hover Row?"=FALSE, "Visibilty"={"Hover Icon"=FALSE, "Selection Icon"=FALSE, "Pin Selection List"=FALSE, "Border"=FALSE, "Scrollbar?"=FALSE, "Help?"=FALSE, "Plot Legend"=FALSE, "Plot Legend Scrollbar"=FALSE, "Settings Icon"=FALSE, "Reorder Hover Icon"=FALSE, "PD Info"=FALSE}, "Mouse Move In Source Pin Seq?"=FALSE, "Mouse Down In Source Pin Seq?"=FALSE, "Changes?"=FALSE, "Same Size?"=FALSE, "UI State"=enum."Enabled", "Check All?"=FALSE, "Color Errors?"=FALSE, "Adv Settings Change?"=FALSE, "P.up Success?"=FALSE}, "All Refs"=[], "Error Map"={}, "Legend"={"Free label"="", "Voltage (V)"=[], "Current (A)"=[]}, "Plot Colors"=[], "Pin Symbols"=[], "Adv Settings"={"Setting.Sel"={"Main"=[], "PL_Freq"=["Freq_50 Hz"]}, "Adv Setting"={"Power line frequency"=1, "Data Capture"=FALSE}, "Item Tag"=""}, "Ref Colors"=[]}, "Adv Settings.Setting.Sel.PL_Freq"=string[] ["Freq_60 Hz"], "Plot Colors"=u32[] [15789890, 5682409, 15535092, 40563, 13983232, 35009, 15113984, 13400487, 15993633, 10221451, 8148942, 15869817, 32914, 9999872, 6271923, 16355671, 11874304, 16860, 14212066, 9836385, 13015295, 16765814, 41756, 15289683, 11194367, 16752575, 3961436, 9999871, 7036516, 3011823, 14210719], "Pin Symbols"=w51, "Flags.Visibilty.PD Info"=w38, "Flags.Visibilty.Help?"=w38, "Flags.Check All?"=w38, "Pin Config.Power Up/Down"=FALSE, "Pin Config.Source Pin Config"=w74, "#Rows"=u32 0, "Pins"=w76, "Pinmap List"=w40, "Indices.Active Row"=w70, "Indices.Selected Row"=w70, "Indices.Actual Sel Row"=w70, "Pin Config.Color Array"=T3 [], "Pin Config.ML Config.Power Down"=FALSE) -> (w78:T14)
        n22 = Build Array (concatenate)("Source", w59) -> (w57:string[])
        n23 = property on="Error Display" class="MCListbox (strict)"(error in=w60, "SelColor"=u32 11783650 ("Color"), "Value"=-1 ("Error Display"), "ColHdrString"=w57, "ActiveCell"=cluster{"Row":i32, "Column":i32} {"Row"=-2, "Column"=-2} ("Active Cell:Active Cell"), "CellFontColor"=u32 2830387 ("Text.Text Colors:Text Color"), "ItemNames"=string[][] [] ("Item Names"), "TopLeft"=cluster{"Row":u32, "Column":u32} {"Row"=0, "Column"=0} ("Top Left Visible Cell"), "ActiveCell"=cluster{"Row":i32, "Column":i32} {"Row"=-1, "Column"=-2} ("Active Cell:Active Cell"), "Height"=u32 22 ("Active Cell:Cell Size:Height")) -> (error out=w65:errorcluster)  [unwired: 1 in, 1 out]
      }
      frame "Plot Colors" {
        # "first 16 colors - NI's standard reference\nnext 15 colors - backup provided by NI\nshuffle both sets seperately to frst 16 are always the priority"
        # "Shuffle the standard reference of plot colors so that there is some variety everytime user loads SFP"
        n24 = Unbundle By Name(w97) -> ("Plot Colors"=w95:u32[])
        n25 = flat-sequence {
          tunnel: w99 -> [w104]
          tunnel: [w103] -> w98
          tunnel: [w102] -> w94
          tunnel: w95 -> [w100]
          frame #0 {
            # "this logic is replica of Shuffle 1D array.vim"
            n26 = for {
              N: 2 -> [_]
              tunnel: [w111] -> w102 mode=concatenating
              shift-right: [w112] -> w103
              shift-left: w104 -> [w113]
              shift-right: [w107] -> _
              shift-left: w100 -> [w109]
              i -> [w106]
              n27 = expression code="x==0?16:15"(w106) -> (w105:i32)
              n28 = Delete From Array(array=w109, length=w105, index=0) -> (deleted portion=w108:u32[], array with subset deleted=w107:u32[])
              n29 = Array Size(array=w108) -> (size(s)=w115:i32)
              n30 = Decrement(x=w115) -> (x-1=w114:i32)
              n31 = for {
                N: w114 -> [_]
                shift-right: [w121] -> w111
                shift-left: w108 -> [w125]
                shift-right: [w119] -> _
                shift-left: w115 -> [w120]
                shift-right: [w116] -> w112
                shift-left: w113 -> [w116]
                n32 = To Double Precision Float(number=w120) -> (double precision float=w117:dbl)
                n33 = Random Number (0-1)() -> (number: 0 to 1=w126:dbl)
                n34 = Multiply(x=w117, y=w126) -> (x*y=w124:dbl)
                n35 = Round Toward -Infinity(1:w124) -> (0:w123:dbl)
                n36 = Decrement(x=w120) -> (x-1=w119:i32)
                n37 = To Long Integer(number=w123) -> (32bit integer=w118:i32)
                n38 = Not Equal?(x=w119, y=w118) -> (x != y?=w122:bool)
                n39 = case shown="True" w122 {
                  tunnel: w125 -> [w127 w131]
                  tunnel: [w127 w130] -> w121
                  tunnel: w119 -> [_ w129]
                  tunnel: w118 -> [_ w128]
                  frame False {
                  }
                  frame True {
                    n40 = in-place "In Place Element Structure" {
                      n41 = in-place-array #1(w131, w129, w128) -> (w135:u32, w134:u32)
                      n42 = Swap Values(12:w135, 14:w134) -> (1:w133:u32, 3:w132:u32)  [unwired: 1 in]
                      n43 = in-place-array #1(w133, w132) -> (w130:u32[])  [unwired: 2 out]
                    }
                  }
                }
              }
            }
          }
        }
        n44 = Bundle By Name(cluster=w97, "Ref Colors"=w94, "Plot Colors"=w94) -> (w96:T14)
      }
      frame "Get Refs" {
        # "pleae dont change the order, the first 10 are used in 'Set to Default' case \nand 'Update Icon State' state"
        # "#coercion dots - 17"
        # "Get references of all controls that have to be disabled during RUN"
        n45 = control-ref of="Scrollbar"() -> (w146:refnum<vi>)
        n46 = control-ref of="Power Down"() -> (w138:refnum<vi>)
        n47 = control-ref of="Power Down Info"() -> (w137:refnum<vi>)
        n48 = control-ref of="Info"() -> (w141:refnum<vi>)
        n49 = control-ref of="Move Up"() -> (w142:refnum<vi>)
        n50 = control-ref of="Move Down"() -> (w143:refnum<vi>)
        n51 = control-ref of="Monitor"() -> (w152:refnum<vi>)
        n52 = control-ref of="Remove"() -> (w151:refnum<vi>)
        n53 = control-ref of="Add"() -> (w150:refnum<vi>)
        n54 = control-ref of="Settings"() -> (w140:refnum<vi>)
        n55 = control-ref of="Power Up/Down"() -> (w139:refnum<vi>)
        n56 = control-ref of="Hover icon"() -> (w148:refnum<vi>)
        n57 = control-ref of="Selection icon"() -> (w147:refnum<vi>)
        n58 = control-ref of="Source Pin Seq"() -> (w149:refnum<vi>)
        n59 = control-ref of="Pin Selection"() -> (w145:refnum<vi>)
        n60 = control-ref of="Pin Config"() -> (w144:refnum<vi>)
        n61 = control-ref of="Color Array"() -> (w136:refnum<vi>)
        n62 = Build Array(w141, w142, w143, w152, w151, w150, w140, w139, w138, w137, w136, w149, w148, w147, w146, w145, w144) -> (w153:refnum<vi>[])
        n63 = Bundle By Name(cluster=w155, "All Refs"=w153) -> (w154:T14)
      }
      frame "Set to Default" {
        w161 = u8 8 ("X Scale.Display Format:Format")
        w162 = u8 8 ("X Scale.Display Format:Format")
        w169 = waveform(dbl)[] [] ("Voltage")
        w175 = u8 2 ("X Scale.Scale Fit")
        w176 = u8 2 ("Y Scale.Scale Fit")
        w172 = u8 1 ("X Scale.Scale Fit")
        w174 = u8 1 ("X Scale.Scale Fit")
        # "Set default values for booleans and graph parameters on UI"
        n64 = Unbundle By Name(w184) -> ("All Refs"=w183:refnum<vi>[])
        n65 = Delete From Array(array=w183, length=10, index=0) -> (deleted portion=w179:refnum<vi>[])  [unwired: 1 out]
        n66 = for {
          shift-right: [w187] -> w178
          shift-left: w180 -> [w189]
          tunnel: w179 -> [w188] mode=indexing
          n67 = To Variant(anything=FALSE) -> (Variant=w185:variant)
          n68 = property on="Property Node" class="Ctl"(reference=w188, error in=w189, "Value"=w185) -> (error out=w187:errorcluster)  [unwired: 1 out]
        }
        n69 = property on="Voltage" class="WFGraph (strict)"(error in=w178, "XScale.Increment"=0.1 ("X Scale.Range:Increment"), "XScale.Minimum"=0.0 ("X Scale.Range:Minimum"), "XScale.Maximum"=1.0 ("X Scale.Range:Maximum"), "XScale.ScaleFit"=w174, "YScale.ScaleFit"=w174, "XScale.ScaleFit"=w176, "YScale.ScaleFit"=w176, "Value"=w169, "YScale.NameLbl.Text"="Voltage (V)" ("Y Scale.Name Label.Text"), "Desc"="<B>Voltage(V) </B>shows voltage measurements measured in the Pins selected" ("Description"), "Caption.Text"="Voltage Measurements", "XScale.Format"=w162, "YScale.Format"=w162) -> (error out=w177:errorcluster)  [unwired: 1 in, 1 out]
        n70 = property on="Current" class="WFGraph (strict)"(error in=w177, "XScale.Increment"=0.1 ("X Scale.Range:Increment"), "XScale.Minimum"=0.0 ("X Scale.Range:Minimum"), "XScale.Maximum"=1.0 ("X Scale.Range:Maximum"), "XScale.ScaleFit"=w172, "YScale.ScaleFit"=w172, "XScale.ScaleFit"=w175, "YScale.ScaleFit"=w175, "Value"=w169, "YScale.NameLbl.Text"="Current (A)" ("Y Scale.Name Label.Text"), "Caption.Text"="Current Measurements", "Desc"="<B>Current(A) </B>shows current measurements measured in the Pins selected" ("Description"), "XScale.Format"=w161, "YScale.Format"=w161) -> (error out=w170:errorcluster)  [unwired: 1 in, 1 out]
      }
      frame "Reset Graph Scales" {
        # "Please do not set scaling of graphs when they have datapoints., it messes with the autoscaling"
        # "Reset graph scales everytime screen is resized"
        n71 = property on="Current" class="WFGraph (strict)"(error in=w194) -> (error out=w192:errorcluster, "Value"=w191:waveform(dbl)[])  [unwired: 1 in, 1 out]
        n72 = Empty Array?(array=w191) -> (empty?=w190:bool)
        n73 = case shown="True" w190 {
          tunnel: [w214 w215] -> w193
          tunnel: w192 -> [w196 w215]
          frame True {
            w211 = u8 2 ("X Scale.Scale Fit")
            w212 = u8 2 ("Y Scale.Scale Fit")
            w208 = u8 0 ("X Scale.Scale Fit")
            w210 = u8 0 ("X Scale.Scale Fit")
            # "empty graphs"
            n74 = property on="Voltage" class="WFGraph (strict)"(error in=w196, "XScale.Increment"=0.1 ("X Scale.Range:Increment"), "XScale.Minimum"=0.0 ("X Scale.Range:Increment"), "XScale.Maximum"=1.0 ("X Scale.Range:Increment"), "YScale.Increment"=0.05 ("Y Scale.Range:Increment"), "YScale.Minimum"=0.0 ("Y Scale.Range:Minimum"), "YScale.Maximum"=5.0 ("Y Scale.Range:Maximum"), "XScale.ScaleFit"=w210, "YScale.ScaleFit"=w210, "XScale.ScaleFit"=w212, "YScale.ScaleFit"=w212) -> (error out=w213:errorcluster)  [unwired: 1 in, 1 out]
            n75 = property on="Current" class="WFGraph (strict)"(error in=w213, "XScale.Increment"=0.1 ("X Scale.Range:Increment"), "XScale.Minimum"=0.0 ("X Scale.Range:Minimum"), "XScale.Maximum"=1.0 ("X Scale.Range:Increment"), "YScale.Increment"=0.05 ("Y Scale.Range:Increment"), "YScale.Minimum"=0.0 ("Y Scale.Range:Minimum"), "YScale.Maximum"=5.0 ("Y Scale.Range:Maximum"), "XScale.ScaleFit"=w208, "YScale.ScaleFit"=w208, "XScale.ScaleFit"=w211, "YScale.ScaleFit"=w211) -> (error out=w214:errorcluster)  [unwired: 1 in, 1 out]
          }
          frame False {
          }
        }
      }
      frame "Get Icons Coords - 1" {
        # "Get necessary co-ordinates and dimensions of icons to programatically overlap controls"
        n76 = property on="Source Pin Seq" class="LstBox (strict)"(error in=w248) -> (error out=w247:errorcluster, "Width"=w246:u32, "Left"=w245:i32, "Height"=w244:u32, "Top"=w243:i32)  [unwired: 1 in, 1 out]
        n77 = property on="Pin Selection" class="LstBox (strict)"(error in=w247) -> (error out=w251:errorcluster, "Width"=w250:u32, "Height"=w249:u32)  [unwired: 1 in, 1 out]
        n78 = property on="Source Pin Seq" class="LstBox (strict)"(error in=w251, "Active Row"=0 ("Active Row:Active Row Number"), "SelColor"=u32 4425401 ("Color Box")) -> (error out=w235:errorcluster, "ActiveRowPosLeft"=w237:i32, "Width"=w257:u32, "Left"=w238:i32)  [unwired: 1 in, 1 out]
        n79 = To Long Integer(number=w257) -> (32bit integer=w230:i32)
        n80 = Subtract(x=w238, y=w237) -> (x-y=w241:i32)
        n81 = Add(x=w237, y=w230) -> (x+y=w256:i32)
        n82 = Quotient & Remainder(x=w241, y=2) -> (floor(x/y)=w239:i32)  [unwired: 1 out]
        n83 = expression code="x-26"(w256) -> (w254:i32)
        n84 = Add(x=w239, y=w237) -> (x+y=w236:i32)
        n85 = property on="Selection icon" class="Bool (strict)"(error in=w235) -> (error out=w223:errorcluster, "Width"=w234:u32, "Height"=w233:u32, "Top"=w232:i32, "Left"=w231:i32)  [unwired: 1 in, 1 out]
        n86 = property on="Info" class="Bool (strict)"(error in=w223) -> (error out=w222:errorcluster, "Width"=w221:u32, "Left"=w220:i32, "Height"=w219:u32, "Top"=w218:i32)  [unwired: 1 in, 1 out]
        n87 = To Long Integer(number=w246) -> (32bit integer=w229:i32)
        n88 = To Long Integer(number=w244) -> (32bit integer=w228:i32)
        n89 = To Long Integer(number=w250) -> (32bit integer=w227:i32)
        n90 = To Long Integer(number=w249) -> (32bit integer=w226:i32)
        n91 = To Long Integer(number=w234) -> (32bit integer=w225:i32)
        n92 = To Long Integer(number=w233) -> (32bit integer=w224:i32)
        n93 = To Long Integer(number=w221) -> (32bit integer=w217:i32)
        n94 = To Long Integer(number=w219) -> (32bit integer=w216:i32)
        n95 = Bundle By Name(cluster=w258, "Coords.Source Pin Seq.Width"=w229, "Coords.Source Pin Seq.Left"=w245, "Coords.Source Pin Seq.Height"=w228, "Coords.Source Pin Seq.Top"=w243, "Pin Selection.Dimensions.Width"=w227, "Pin Selection.Dimensions.Height"=w226, "Coords.List Coords.Icon Left"=w254, "Coords.List Coords.Icon Top Offset"=23, "Coords.Border Left"=w236, "Coords.Selection Icon.Width"=w225, "Coords.Selection Icon.Height"=w224, "Coords.Selection Icon.Top"=w232, "Coords.Selection Icon.Left"=w231, "Coords.Info Icon.Width"=w217, "Coords.Info Icon.Left"=w220, "Coords.Info Icon.Height"=w216, "Coords.Info Icon.Top"=w218) -> (w255:T14)
      }
      frame "Get Icons Coords - 2" {
        # "Align monitor icon's right with graph's right"
        # "#coercion dot - 1"
        # "1020-24-val"
        # "column headers row"
        # "Get necessary co-ordinates and dimensions of icons to programatically position on UI"
        n96 = property on="Error Display" class="MCListbox (strict)" props=["Width", "Left", "Height", "Top", "ActiveCell", "Height", "CellBG"](error in=w274, "ActiveCell"=cluster{"Row":i32, "Column":i32} {"Row"=-1, "Column"=-2} ("Active Cell:Active Cell"), "CellBG"=u32 16250871) -> (error out=w273:errorcluster, "Height"=w278:u32, "Height"=w277:u32)  [unwired: 1 in, 4 out]
        n97 = property on="Voltage" class="WFGraph (strict)"(error in=w273) -> (error out=w272:errorcluster, "Height"=w275:u32, "Width"=w271:u32, "Left"=w270:i32, "Plot Bounds"=w268:T15)  [unwired: 1 in, 1 out]
        n98 = Unbundle By Name(w268) -> ("Right"=w266:i16)
        n99 = To Long Integer(number=w271) -> (32bit integer=w260:i32)
        n100 = Add(x=w260, y=w270) -> (x+y=w264:i32)
        n101 = To Long Integer(number=w266) -> (32bit integer=w259:i32)
        n102 = Subtract(x=w264, y=w259) -> (x-y=w263:i32)
        n103 = Subtract(x=w264, y=w263) -> (x-y=w262:i32)
        n104 = Subtract(x=w278, y=w277) -> (x-y=w269:u32)
        n105 = Subtract(x=w262, y=24) -> (x-y=w267:i32)
        n106 = property on="Monitor" class="Bool (strict)" props=["Width", "Left", "Left", "Height", "Top"](error in=w272, "Left"=w267) -> (error out=w293:errorcluster, "Width"=w291:u32, "Left"=w292:i32)  [unwired: 1 in, 3 out]
        n107 = To Unsigned Long Integer(number=w292) -> (unsigned 32bit integer=w289:u32)
        n108 = property on="Legend" class="Clust (strict)" props=["Width", "Left", "Height", "Top"](error in=w293) -> (error out=w288:errorcluster, "Width"=w295:u32, "Height"=w294:u32)  [unwired: 1 in, 3 out]
        n109 = Add(x=w291, y=w289) -> (x+y=w290:u32)
        n110 = property on="Empty Legend" class="Clust (strict)"(error in=w288) -> (error out=w287:errorcluster, "Width"=w286:u32, "Left"=w285:i32, "Height"=w284:u32, "Top"=w283:i32)  [unwired: 1 in, 1 out]
        n111 = To Long Integer(number=w269) -> (32bit integer=w261:i32)
        n112 = To Long Integer(number=w290) -> (32bit integer=w282:i32)
        n113 = To Long Integer(number=w295) -> (32bit integer=w299:i32)
        n114 = To Long Integer(number=w294) -> (32bit integer=w298:i32)
        n115 = To Long Integer(number=w286) -> (32bit integer=w281:i32)
        n116 = To Long Integer(number=w284) -> (32bit integer=w280:i32)
        n117 = Bundle By Name(cluster=w301, "Coords.Error Display.Height"=w261, "Coords.Graph Size.Height"=w275, "Coords.Graph Size.Width"=w271, "Coords.Monitor.Right"=w282, "Coords.Plot Legend.Width"=w299, "Coords.Plot Legend.Left"=846 ("Left"), "Coords.Plot Legend.Height"=w298, "Coords.Plot Legend.Top"=-2 ("Top"), "Coords.Empty Legend.Width"=w281, "Coords.Empty Legend.Left"=w285, "Coords.Empty Legend.Height"=w280, "Coords.Empty Legend.Top"=w283) -> (w300:T14)
      }
      frame "Get Icons Coords - 3" {
        # "Get necessary co-ordinates and dimensions of icons to programatically overlap controls over Source Pin Sequence"
        n118 = property on="Source Pin Seq" class="LstBox (strict)"(error in=w315, "Active Row"=0 ("Active Row:Active Row Number")) -> (error out=w310:errorcluster, "ActiveRowPosLeft"=w314:i32, "Cell Height"=w312:i32)  [unwired: 1 in, 1 out]
        n119 = expression code="x/2-12"(w312) -> (w311:i32)
        n120 = property on="Reorder Hover Icon" class="Bool (strict)"(error in=w310) -> (error out=w307:errorcluster, "Width"=w322:u32, "Height"=w321:u32, "Top"=w320:i32, "Left"=w319:i32)  [unwired: 1 in, 1 out]
        n121 = expression code="x+2"(w314) -> (w313:i32)
        n122 = To Long Integer(number=w322) -> (32bit integer=w318:i32)
        n123 = To Long Integer(number=w321) -> (32bit integer=w317:i32)
        n124 = property on="Power Down Info" class="Bool (strict)"(error in=w307) -> (error out=w306:errorcluster, "Width"=w309:u32, "Left"=w304:i32, "Height"=w308:u32, "Top"=w302:i32)  [unwired: 1 in, 1 out]
        n125 = To Long Integer(number=w309) -> (32bit integer=w305:i32)
        n126 = To Long Integer(number=w308) -> (32bit integer=w303:i32)
        n127 = Bundle By Name(cluster=w324, "Coords.List Coords.Reorder Icon Left"=w313, "Coords.List Coords.Reorder Icon Top Offset"=w311, "Coords.Reorder Hover Icon.Width"=w318, "Coords.Reorder Hover Icon.Left"=w317, "Coords.Reorder Hover Icon.Height"=w320, "Coords.Reorder Hover Icon.Top"=w319, "Coords.PDInfo Icon.Width"=w305, "Coords.PDInfo Icon.Left"=w304, "Coords.PDInfo Icon.Height"=w303, "Coords.PDInfo Icon.Top"=w302) -> (w323:T14)
      }
      frame "Format Controls" {
        # "Format color and row height of Pin Selection List, display format of inputs"
        n128 = property on="Pin Selection" class="LstBox (strict)"(error in=w330, "SelColor"=u32 11783650 ("Color"), "Value"=-1 ("Pin Dropdown"), "Active Row"=-2 ("Active Row:Active Row Number"), "Cell Height"=18 ("Active Row:Cell Height"), "CellFontColor"=u32 0 ("Active Row:Cell Font:Color"), "Number of Rows"=u32 0) -> (error out=w336:errorcluster)  [unwired: 1 in, 1 out]
        n129 = control-ref of="COMPLIANCE LIMIT"() -> (w332:refnum<vi>)
        n130 = control-ref of="START DELAY"() -> (w333:refnum<vi>)
        n131 = control-ref of="RAMP RATE"() -> (w334:refnum<vi>)
        n132 = Build Array(w332, w333, w334) -> (w331:refnum<vi>[])
        n133 = for {
          tunnel: w336 -> [w345]
          tunnel: [w344] -> w335 mode=indexing
          tunnel: w331 -> [w343] mode=indexing
          # "SI notation"
          n134 = property on="Property Node" class="DigNum (strict)"(reference=w343, error in=w345, "Format"=u8 8 ("Display Format:Format")) -> (error out=w344:errorcluster)  [unwired: 1 out]
        }
        n135 = Merge Errors(w335) -> (w328:errorcluster)
        n136 = property on="START DELAY" class="DigNum (strict)"(error in=w328, "FormatString"="%_6p s" ("Format String")) -> (error out=w326:errorcluster)  [unwired: 1 in, 1 out]
      }
      frame "Define Error Map" {
        # "Define list of all errors/warnings for input validation"
        n137 = in-place "In Place Element Structure" {
          n138 = in-place-cluster #2(w347) -> ("Error Map"=w350:map{i32, string})
          n139 = for {
            tunnel: string[] ["Pin Name cannot be empty", "Pin Name no longer available in active pinmap", "Pin Name already exists in the sequence", "'Target Value' cannot be less than 'Start Value' for sequence power up", "'Start Value' cannot be less than 'Target Value' for sequence power down", "'Compliance Limit' cannot be zero", "'Ramp Rate' cannot be zero unless 'Default Ramp Rate' is selected", "'Relative To' can only be 'Power sequence start' for first pin in sequence"] -> [w354] mode=indexing
            shift-right: [w352] -> w349
            shift-left: w350 -> [w353]
            i -> [w355]
            # "for each possible check"
            n140 = Insert Into Map(map in=w353, key=w355, value=w354) -> (map out=w352:map{i32, string})  [unwired: 2 out]
          }
          n141 = in-place-cluster #2("Error Map"=w349) -> (w346:T14)
        }
      }
      frame "--- Capture User Events ---" {
      }
      frame "", "Event" {
        # "Capture various events generated by user on UI"
        n142 = event shown="[0] Timeout" {
          selector: _ -> [_ _ _ _ _ _ _ _ _ _ _ _ _ _ _ _ _ _ _ _ _ _ _ _ _ _ _ _ _ _ _ _ _ _ _ _ _ _ _ _ _]
          dyn-events: _ -> [_ _ _ _ _ _ _ _ _ _ _ _ _ _ _ _ _ _ _ _ _ _ _ _ _ _ _ _ _ _ _ _ _ _ _ _ _ _ _ _ _]
          timeout: 100 -> [_ _ _ _ _ _ _ _ _ _ _ _ _ _ _ _ _ _ _ _ _ _ _ _ _ _ _ _ _ _ _ _ _ _ _ _ _ _ _ _ _]
          tunnel: [w366 w378 w402 w411 w413 w416 w436 w452 w479 w509 w533 w548 w568 w589 w601 w614 w627 w630 w633 w636 w639 w642 w645 w651 w662 w667 w679 w692 w706 w714 w726 w744 w750 w757 w770 w782 w794 w806 w807 w830 w849] -> w363
          tunnel: w362 -> [w368 w380 w403 w411 w413 w417 w438 w449 w476 w508 w534 w549 w569 w591 w604 w618 w627 w630 w633 w636 w639 w642 w645 w652 w662 w668 w680 w693 w708 w715 w727 w741 w750 w758 w771 w784 w797 w806 w810 w832 w850]
          tunnel: w360 -> [w365 w379 w400 _ _ _ w437 w453 w481 w507 w535 _ _ w590 w603 w617 _ _ _ _ _ _ _ w650 _ w666 w678 w691 w705 w713 w725 w740 _ w756 w769 w783 w796 _ _ w831 w845]
          tunnel: w359 -> [w367 w387 w404 w410 w412 w414 w440 w455 w470 w511 w531 w546 w566 w592 w605 w619 w626 w629 w632 w635 w638 w641 w644 w653 w661 w669 w681 w694 w707 w711 w723 w736 w749 w759 w772 w779 w795 w805 w811 w822 w847]
          tunnel: [w367 w377 w399 w410 w412 w414 w435 w454 w480 w506 w532 w546 w566 w588 w600 w613 w626 w629 w632 w635 w638 w641 w644 w648 w660 w664 w676 w689 w702 w712 w724 w743 w748 w755 w768 w781 w792 w804 w811 w835 w847] -> w358
          event Timeout {
            # "Constantly check for screen resizing, ML events and pinmap updates"
            n143 = event-data() -> ()  [unwired: 1 in, 1 out]
            n144 = for {
              tunnel: w365 -> [w371]
              shift-right: [w372] -> w366
              shift-left: w368 -> [w373]
              tunnel: string[] ["Check UI Resize?", "Get Pinmap List", "Monitor ML Controls State"] -> [w369] mode=indexing
              n145 = Enqueue Element(queue=w371, element=w369, timeout in ms (-1)=50, error in (no error)=w373) -> (error out=w372:errorcluster)  [unwired: 2 out]
            }
          }
          event "Settings": Mouse Down? {
            # "1 - Left click\n2 - Right click"
            # "Generated when clicks on Settings icon"
            n146 = event-data() -> ("Button"=w383:u16)  [unwired: 1 in]
            n147 = Equal?(x=w383, y=u16 2) -> (x = y?=w374:bool)
            n148 = case shown="False" w374 {
              tunnel: string[] ["Update Icon State"] -> [w391 _]
              tunnel: w380 -> [w390 w397]
              tunnel: w379 -> [w389 _]
              tunnel: [w388 w397] -> w378
              frame False {
                n149 = for {
                  tunnel: w389 -> [w394]
                  shift-right: [w395] -> w388
                  shift-left: w390 -> [w396]
                  tunnel: w391 -> [w392] mode=indexing
                  n150 = Enqueue Element(queue=w394, element=w392, timeout in ms (-1)=50, error in (no error)=w396) -> (error out=w395:errorcluster)  [unwired: 2 out]
                }
              }
              frame True {
              }
            }
            n151 = Select(t=u16 1 ("Button"), s=w374, f=u16 2) -> (s? t:f=w382:u16)
            n152 = Bundle By Name(cluster=w387, "Flags.Visibilty.Settings Icon"=TRUE, "Action"="Settings") -> (w377:T14)
            n153 = event-data ("Event Filter Node")("Button"=w382, "Discard?"=w374) -> ()  [unwired: 1 in, 1 out]
          }
          event "Settings": Shortcut Menu Selection (User) {
            # "Generated when user selects any item from the shortcut menu of Settings icon"
            n154 = event-data() -> ("ItemTag"=w398:string)  [unwired: 1 in]
            n155 = Bundle By Name(cluster=w404, "Adv Settings.Item Tag"=w398) -> (w399:T14)
            n156 = for {
              tunnel: w400 -> [w407]
              shift-right: [w408] -> w402
              shift-left: w403 -> [w409]
              tunnel: string[] ["Settings - Menu Selection(User)", "Update Meas Config - 2", "Update Icon State"] -> [w405] mode=indexing
              n157 = Enqueue Element(queue=w407, element=w405, timeout in ms (-1)=50, error in (no error)=w409) -> (error out=w408:errorcluster)  [unwired: 2 out]
            }
          }
          event Value Change {
            # "NOTE - DO NOT delete this event case. It impacts MeasLink framework\nconfiguration changes' detection!"
            # "Generated when user modifies Powerline frequency option in Settings menu"
            n158 = event-data() -> ()  [unwired: 1 in, 1 out]
          }
          event "Data Capture": Value Change {
            # "NOTE - DO NOT delete this event case. It impacts MeasLink framework\nconfiguration changes' detection!"
            # "Generated when user selects/deselects Capture data option in Settings menu"
            n159 = event-data() -> ()  [unwired: 1 in, 1 out]
          }
          event "Settings": Shortcut Menu Activation? {
            # "Enable all the items which have have been previously selected"
            # "Generated when user accesses shortcut menu of Settings icon"
            n160 = event-data() -> ("MenuRef"=w415:refnum<k9>)  [unwired: 1 in]
            n161 = Unbundle By Name(w414) -> ("Adv Settings.Setting.Sel.Main"=w420:string[], "Adv Settings.Setting.Sel.PL_Freq"=w421:string[])
            n162 = for {
              tunnel: w415 -> [w429]
              tunnel: w421 -> [w428] mode=indexing
              shift-right: [w430] -> w418
              shift-left: w417 -> [w431]
              tunnel: [w427] -> w419
              # "Check All selected settings"
              n163 = Set Menu Item Info(6:TRUE ("checked"), 7:w428, 8:w431, 11:w429) -> (0:w430:errorcluster, 3:w427:refnum<k9>)  [unwired: 3 in]
            }
            n164 = for {
              tunnel: w419 -> [w423]
              tunnel: w420 -> [w422] mode=indexing
              shift-right: [w424] -> w416
              shift-left: w418 -> [w425]
              # "Check All selected settings"
              n165 = Set Menu Item Info(6:TRUE ("checked"), 7:w422, 8:w425, 11:w423) -> (0:w424:errorcluster)  [unwired: 3 in, 1 out]
            }
            n166 = event-data ("Event Filter Node")() -> ()  [unwired: 2 in, 1 out]
          }
          event "Settings": event #0x44 {
            # "Generated when user clicks anywhere other than shortcut menu of Settings icon when its active"
            n167 = event-data() -> ()  [unwired: 1 in, 1 out]
            n168 = for {
              tunnel: w437 -> [w443]
              shift-right: [w444] -> w436
              shift-left: w438 -> [w445]
              tunnel: string[] ["Update Icon State"] -> [w441] mode=indexing
              n169 = Enqueue Element(queue=w443, element=w441, timeout in ms (-1)=50, error in (no error)=w445) -> (error out=w444:errorcluster)  [unwired: 2 out]
            }
            n170 = Bundle By Name(cluster=w440, "Flags.Visibilty.Settings Icon"=FALSE, "Action"="Settings") -> (w435:T14)
          }
          event "Source Pin Seq": Mouse Move {
            # "Generate when mouse movement on UI is inside Source Pin Sequence"
            n171 = event-data() -> ("Coords.Horizontal"=w451:i32, "Coords.Vertical"=w450:i32, "Coords"=w448:T16)  [unwired: 1 in]
            n172 = invoke on="Source Pin Seq" class="LstBox (strict)" method="Point To Row"(error in=w449, "Point"=w448) -> (error out=w446:errorcluster, "InBounds"=w447:bool)  [unwired: 5 in, 5 out]
            n173 = case shown="True" w447 {
              tunnel: w453 -> [_ w460]
              tunnel: [w456 w459] -> w452
              tunnel: w446 -> [w456 w457]
              frame False {
              }
              frame True {
                # "in source pin seq bounds"
                n174 = for {
                  shift-right: [w464] -> w459
                  shift-left: w457 -> [w465]
                  tunnel: w460 -> [w463]
                  tunnel: string[] ["Check Scroll Direction", "Check Scroll for Reordering", "Update Scrollbar", "Get Mouse Hover Info", "Check Hover Action"] -> [w462] mode=indexing
                  n175 = Enqueue Element(queue=w463, element=w462, timeout in ms (-1)=50, error in (no error)=w465) -> (error out=w464:errorcluster)  [unwired: 2 out]
                }
              }
            }
            n176 = Bundle By Name(cluster=w455, "Coords.Hover Coords.Horizontal"=w451, "Coords.Hover Coords.Vertical"=w450) -> (w454:T14)
          }
          event "Source Pin Seq": Mouse Down? {
            # "#coercion dot"
            # "consider events only in actual pin rows and not in alternate empty rows\nalso do not Restore Cell Font Color if mouse down is already on selected row"
            # "Generate when user selects any row in Source Pin Sequence"
            n177 = event-data() -> ("Coords.Horizontal"=w478:i32, "Coords.Vertical"=w477:i32, "Coords"=w475:T16)  [unwired: 1 in]
            n178 = Unbundle By Name(w470) -> ("Indices.Selected Row"=w467:i32)
            n179 = invoke on="Source Pin Seq" class="LstBox (strict)" method="Point To Row"(error in=w476, "Point"=w475) -> (error out=w471:errorcluster, "Row"=w468:i32)  [unwired: 5 in, 5 out]
            n180 = Not Equal?(x=w467, y=w468) -> (x != y?=w466:bool)
            n181 = Quotient & Remainder(x=w468, y=2) -> (x-y*floor(x/y)=w474:i32)  [unwired: 1 out]
            n182 = Not Equal To 0?(x=w474) -> (x != 0?=w473:bool)
            n183 = case shown="False" w473 {
              selector: w473 -> [_ w504]
              tunnel: w470 -> [w496 w502]
              tunnel: w481 -> [w495 _]
              tunnel: [w493 w502] -> w480
              tunnel: [w492 w503] -> w479
              tunnel: w478 -> [w491 _]
              tunnel: w477 -> [w489 _]
              tunnel: [FALSE w504] -> w472
              tunnel: w471 -> [w482 w503]
              tunnel: w466 -> [w488 _]
              frame False {
                # "valid pin row selected"
                n184 = Select(t="Restore Cell Font Color", s=w488, f="") -> (s? t:f=w483:string)
                n185 = Bundle By Name(cluster=w496, "Seq Reorder.Drag?"=TRUE, "Coords.Selection Coords.Horizontal"=w491, "Coords.Selection Coords.Vertical"=w489) -> (w493:T14)
                n186 = Build Array (concatenate)(w483, string[] ["Check Empty Source Pin Seq"]) -> (w484:string[])
                n187 = for {
                  shift-right: [w500] -> w492
                  shift-left: w482 -> [w501]
                  tunnel: w495 -> [w499]
                  tunnel: w484 -> [w498] mode=indexing
                  n188 = Enqueue Element(queue=w499, element=w498, timeout in ms (-1)=50, error in (no error)=w501) -> (error out=w500:errorcluster)  [unwired: 2 out]
                }
              }
              frame True {
                # "empty row selected - discard"
              }
            }
            n189 = event-data ("Event Filter Node")("Discard?"=w472) -> ()  [unwired: 1 in, 1 out]
          }
          event "Monitor": Value Change {
            # "Generated when user clicks on Monitor icon"
            n190 = event-data() -> ("NewVal"=w505:bool)  [unwired: 1 in]
            n191 = Bundle By Name(cluster=w511, "Flags.Visibilty.Plot Legend"=w505) -> (w506:T14)
            n192 = for {
              shift-right: [w515] -> w509
              shift-left: w508 -> [w516]
              tunnel: w507 -> [w514]
              tunnel: string[] ["Show/Hide Legend"] -> [w513] mode=indexing
              n193 = Enqueue Element(queue=w514, element=w513, timeout in ms (-1)=50, error in (no error)=w516) -> (error out=w515:errorcluster)  [unwired: 2 out]
            }
          }
          event "Legend": Value Change {
            # "In array, when scrollbar is visible, by default one new element is shown. If user edits that element\nignore it else it messes with whole pin configuration in plot legend"
            # "Generated when user clicks on any entry in Plot Legend"
            n194 = event-data() -> ("NewVal"=w520:T1)  [unwired: 1 in]
            n195 = Unbundle By Name(w531) -> ("Legend"=w522:T12, "#Rows"=w528:u32)
            n196 = Unbundle By Name(w520) -> ("Voltage (V)"=w530:T17, "Current (A)"=w529:T17)
            n197 = expression code="x/2"(w528) -> (w525:u32)
            n198 = Array Size(array=w530) -> (size(s)=w527:i32)
            n199 = Array Size(array=w529) -> (size(s)=w526:i32)
            n200 = To Long Integer(number=w525) -> (32bit integer=w519:i32)
            n201 = Not Equal?(x=w519, y=w527) -> (x != y?=w524:bool)
            n202 = Not Equal?(x=w519, y=w526) -> (x != y?=w523:bool)
            n203 = Compound Arithmetic op=OR(w524, w523) -> (w518:bool)
            n204 = case shown="True" w518 {
              tunnel: w522 -> [_ w539]
              tunnel: [w537 w539] -> w521
              tunnel: w520 -> [w537 _]
              tunnel: [string[] ["Update Plot Visibility", "Update UI"] string[] ["Update Plot Legend", "Update UI"]] -> w517
              frame False {
                # "#coercion dot"
                # "Valid change"
              }
              frame True {
                # "Ignore"
              }
            }
            n205 = for {
              shift-right: [w543] -> w533
              shift-left: w534 -> [w544]
              tunnel: w535 -> [w542]
              tunnel: w517 -> [w541] mode=indexing
              n206 = Enqueue Element(queue=w542, element=w541, timeout in ms (-1)=50, error in (no error)=w544) -> (error out=w543:errorcluster)  [unwired: 2 out]
            }
            n207 = Bundle By Name(cluster=w531, "Legend"=w521) -> (w532:T14)
          }
          event "Legend.Voltage (V)": Mouse Down; "Legend.Voltage (V)": Mouse Move {
            # "adjust toprow visible so that new element in array is not visible to user"
            n208 = event-data() -> ()  [unwired: 1 in, 1 out]
            n209 = Unbundle By Name(w546) -> ("#Rows"=w547:u32, "Flags.Visibilty.Plot Legend Scrollbar"=w545:bool)
            n210 = case shown="True" w545 {
              tunnel: w549 -> [w550 w559]
              tunnel: [w550 w557] -> w548
              tunnel: w547 -> [_ w556]
              frame False {
                # "Nothing to do"
              }
              frame True {
                # "Plot legend scrollbar visible when pin count>4"
                n211 = expression code="x/2-4"(w556) -> (w555:u32)
                n212 = property on="Voltage (V)" class="Arr (strict)"(error in=w559) -> (error out=w558:errorcluster, "Index Values"=w551:u32[])  [unwired: 1 in, 1 out]
                n213 = To Long Integer(number=w555) -> (32bit integer=w553:i32)
                n214 = Index Array(array=w551) -> (element=w554:u32)  [unwired: 1 in]
                n215 = Greater?(x=w554, y=w553) -> (0:w552:bool)
                n216 = case shown="True" w552 {
                  tunnel: w558 -> [w560 w564]
                  tunnel: [w560 w563] -> w557
                  tunnel: w551 -> [_ w562]
                  frame False {
                  }
                  frame True {
                    # "new element is visible"
                    n217 = Decrement(x=w562) -> (x-1=w561:u32[])
                    n218 = property on="Voltage (V)" class="Arr (strict)"(error in=w564, "Index Values"=w561) -> (error out=w563:errorcluster)  [unwired: 1 in, 1 out]
                  }
                }
              }
            }
          }
          event "Legend.Current (A)": Mouse Down; "Legend.Current (A)": Mouse Move {
            # "adjust toprow visible so that new element in array is not visible to user"
            n219 = event-data() -> ()  [unwired: 1 in, 1 out]
            n220 = Unbundle By Name(w566) -> ("#Rows"=w567:u32, "Flags.Visibilty.Plot Legend Scrollbar"=w565:bool)
            n221 = case shown="True" w565 {
              tunnel: w569 -> [w570 w579]
              tunnel: [w570 w577] -> w568
              tunnel: w567 -> [_ w576]
              frame False {
                # "Nothing to do"
              }
              frame True {
                # "Plot legend scrollbar visible when pin count>4"
                n222 = expression code="x/2-4"(w576) -> (w575:u32)
                n223 = property on="Current (A)" class="Arr (strict)"(error in=w579) -> (error out=w578:errorcluster, "Index Values"=w571:u32[])  [unwired: 1 in, 1 out]
                n224 = To Long Integer(number=w575) -> (32bit integer=w573:i32)
                n225 = Index Array(array=w571) -> (element=w574:u32)  [unwired: 1 in]
                n226 = Greater?(x=w574, y=w573) -> (0:w572:bool)
                n227 = case shown="True" w572 {
                  tunnel: w578 -> [w580 w584]
                  tunnel: [w580 w583] -> w577
                  tunnel: w571 -> [_ w582]
                  frame False {
                  }
                  frame True {
                    # "new element is visible"
                    n228 = Decrement(x=w582) -> (x-1=w581:u32[])
                    n229 = property on="Current (A)" class="Arr (strict)"(error in=w584, "Index Values"=w581) -> (error out=w583:errorcluster)  [unwired: 1 in, 1 out]
                  }
                }
              }
            }
          }
          event "Move Up": Value Change {
            # "Generate when user click on Move Up icon to move the selected pin a level up in 'Source Pin Sequence'"
            n230 = event-data() -> ()  [unwired: 1 in, 1 out]
            n231 = for {
              shift-right: [w596] -> w589
              shift-left: w591 -> [w597]
              tunnel: w590 -> [w595]
              tunnel: string[] ["Move Pin"] -> [w594] mode=indexing
              n232 = Enqueue Element(queue=w595, element=w594, timeout in ms (-1)=50, error in (no error)=w597) -> (error out=w596:errorcluster)  [unwired: 2 out]
            }
            n233 = Bundle By Name(cluster=w592, "Action"="Up", "Seq Reorder.Up?"=TRUE) -> (w588:T14)
          }
          event "Move Down": Value Change {
            # "Generate when user click on Move Down  icon to move the selected pin a level down in 'Source Pin Sequence'"
            n234 = event-data() -> ()  [unwired: 1 in, 1 out]
            n235 = for {
              shift-right: [w609] -> w601
              shift-left: w604 -> [w610]
              tunnel: w603 -> [w608]
              tunnel: string[] ["Move Pin"] -> [w607] mode=indexing
              n236 = Enqueue Element(queue=w608, element=w607, timeout in ms (-1)=50, error in (no error)=w610) -> (error out=w609:errorcluster)  [unwired: 2 out]
            }
            n237 = Bundle By Name(cluster=w605, "Action"="Down", "Seq Reorder.Up?"=FALSE) -> (w600:T14)
          }
          event "Selection icon": Mouse Down? {
            # "Generated when user clicks on white dropdown icon of selected pin to modify Source Pin"
            n238 = event-data() -> ("Coords.Horizontal"=w612:i32, "Coords.Vertical"=w611:i32)  [unwired: 1 in]
            n239 = for {
              shift-right: [w623] -> w614
              shift-left: w618 -> [w624]
              tunnel: w617 -> [w622]
              tunnel: string[] ["Check Hide/Unhide Listbox"] -> [w621] mode=indexing
              n240 = Enqueue Element(queue=w622, element=w621, timeout in ms (-1)=50, error in (no error)=w624) -> (error out=w623:errorcluster)  [unwired: 2 out]
            }
            n241 = Bundle By Name(cluster=w619, "Coords.Selection Coords.Horizontal"=w612, "Coords.Selection Coords.Vertical"=w611) -> (w613:T14)
            n242 = event-data ("Event Filter Node")("Discard?"=TRUE) -> ()  [unwired: 1 in, 1 out]
          }
          event Shortcut Menu Activation? {
            # "Discard runtime shortcut menu for 'Empty Legend'"
            n243 = event-data() -> ()  [unwired: 1 in, 1 out]
            n244 = event-data ("Event Filter Node")("Discard?"=TRUE) -> ()  [unwired: 1 in, 1 out]
          }
          event Shortcut Menu Activation? {
            # "Discard runtime shortcut menu for 'Pin Config'"
            n245 = event-data() -> ()  [unwired: 1 in, 1 out]
            n246 = event-data ("Event Filter Node")("Discard?"=TRUE) -> ()  [unwired: 1 in, 1 out]
          }
          event "Tab": Shortcut Menu Activation? {
            # "Discard runtime shortcut menu for 'Pin Config'"
            n247 = event-data() -> ()  [unwired: 1 in, 1 out]
            n248 = event-data ("Event Filter Node")("Discard?"=TRUE) -> ()  [unwired: 1 in, 1 out]
          }
          event Shortcut Menu Activation? {
            # "Discard runtime shortcut menu for 'Color Array'"
            n249 = event-data() -> ()  [unwired: 1 in, 1 out]
            n250 = event-data ("Event Filter Node")("Discard?"=TRUE) -> ()  [unwired: 1 in, 1 out]
          }
          event "Power Down": Shortcut Menu Activation? {
            # "Discard runtime shortcut menu for 'Power Down'"
            n251 = event-data() -> ()  [unwired: 1 in, 1 out]
            n252 = event-data ("Event Filter Node")("Discard?"=TRUE) -> ()  [unwired: 1 in, 1 out]
          }
          event "Scrollbar": Shortcut Menu Activation? {
            # "Discard runtime shortcut menu for Source Pin Seq scrollbar"
            n253 = event-data() -> ()  [unwired: 1 in, 1 out]
            n254 = event-data ("Event Filter Node")("Discard?"=TRUE) -> ()  [unwired: 1 in, 1 out]
          }
          event "Legend": Shortcut Menu Activation? {
            # "Discard runtime shortcut menu for 'Legend'"
            n255 = event-data() -> ()  [unwired: 1 in, 1 out]
            n256 = event-data ("Event Filter Node")("Discard?"=TRUE) -> ()  [unwired: 1 in, 1 out]
          }
          event "Pin Selection": Value Change {
            # "Generated when user selects a pin from 'Pin Selection List' to change Source Pin mapping"
            n257 = event-data() -> ("NewVal"=w647:i32)  [unwired: 1 in]
            n258 = Bundle By Name(cluster=w653, "Seq Reorder.Drag?"=FALSE, "Indices.Pin Change"=w647) -> (w648:T14)
            n259 = for {
              tunnel: w650 -> [w656]
              tunnel: string[] ["Update Pin Name", "Update UI", "Update Plot Legend", "Hide Listbox", "Update Active Pin Config", "Update Meas Config", "Validate Inputs", "Update Error Info", "Update Error Display Top Row", "Update Error Display Scrollbar", "Update Power Down"] -> [w655] mode=indexing
              shift-right: [w657] -> w651
              shift-left: w652 -> [w658]
              n260 = Enqueue Element(queue=w656, element=w655, timeout in ms (-1)=50, error in (no error)=w658) -> (error out=w657:errorcluster)  [unwired: 2 out]
            }
          }
          event "Pin Selection": Mouse Enter {
            # "Generated when mouse enters 'Pin Selection List' control"
            n261 = event-data() -> ()  [unwired: 1 in, 1 out]
            n262 = Bundle By Name(cluster=w661, "Seq Reorder.Drag?"=FALSE) -> (w660:T14)
          }
          event "Remove": Value Change {
            # "Remove selected pin from  'Source Pin Seq'"
            n263 = event-data() -> ()  [unwired: 1 in, 1 out]
            n264 = for {
              tunnel: w666 -> [w672]
              tunnel: string[] ["Check Delete Pin?"] -> [w671] mode=indexing
              shift-right: [w673] -> w667
              shift-left: w668 -> [w674]
              n265 = Enqueue Element(queue=w672, element=w671, timeout in ms (-1)=50, error in (no error)=w674) -> (error out=w673:errorcluster)  [unwired: 2 out]
            }
            n266 = Bundle By Name(cluster=w669, "Action"="Delete") -> (w664:T14)
          }
          event "Add": Value Change {
            # "Add pin to 'Source Pin Seq'"
            n267 = event-data() -> ()  [unwired: 1 in, 1 out]
            n268 = for {
              tunnel: w678 -> [w684]
              tunnel: string[] ["Restore Cell Font Color", "Add Pin", "Read Pin List", "Format Pin List", "Check Pin List Scrollbar", "Update UI", "Update Plot Legend", "Get Mouse Down Row Info", "Update Icon State", "Overlap Selection Pin List", "Update Power Down"] -> [w683] mode=indexing
              shift-right: [w685] -> w679
              shift-left: w680 -> [w686]
              n269 = Enqueue Element(queue=w684, element=w683, timeout in ms (-1)=50, error in (no error)=w686) -> (error out=w685:errorcluster)  [unwired: 2 out]
            }
            n270 = Bundle By Name(cluster=w681, "Action"="Add") -> (w676:T14)
          }
          event "Scrollbar": Value Change {
            # "Generated when user scrolls the scrollbar for 'Source Pin Seq'"
            n271 = event-data() -> ("OldVal"=w687:i32, "NewVal"=w688:i32)  [unwired: 1 in]
            n272 = Bundle By Name(cluster=w694, "Scrollbar.Old Val"=w687, "Scrollbar.New Val"=w688) -> (w689:T14)
            n273 = for {
              tunnel: w691 -> [w697]
              tunnel: string[] ["Set Source Pin Seq Top Row", "Update UI", "Update Plot Legend", "Hide Border", "Restore Previous to Default"] -> [w696] mode=indexing
              shift-right: [w698] -> w692
              shift-left: w693 -> [w699]
              n274 = Enqueue Element(queue=w697, element=w696, timeout in ms (-1)=50, error in (no error)=w699) -> (error out=w698:errorcluster)  [unwired: 2 out]
            }
          }
          event "Pin Selection": Mouse Move {
            # "Generated when mouse moves over 'Pin Selection List'"
            n275 = event-data() -> ("Coords.Horizontal"=w701:i32, "Coords.Vertical"=w700:i32)  [unwired: 1 in]
            n276 = Enqueue Element(queue=w705, element="Format Selection List", timeout in ms (-1)=50, error in (no error)=w708) -> (error out=w706:errorcluster)  [unwired: 2 out]
            n277 = Bundle By Name(cluster=w707, "Pin Selection.Selection Coords.Horizontal"=w701, "Pin Selection.Selection Coords.Vertical"=w700) -> (w702:T14)
          }
          event "Info": Value Change {
            # "Generated when user clicks on 'Info' icon"
            n278 = event-data() -> ()  [unwired: 1 in, 1 out]
            n279 = for {
              tunnel: w713 -> [w718]
              shift-right: [w719] -> w714
              shift-left: w715 -> [w720]
              tunnel: string[] ["Hide Image"] -> [w716] mode=indexing
              n280 = Enqueue Element(queue=w718, element=w716, timeout in ms (-1)=50, error in (no error)=w720) -> (error out=w719:errorcluster)  [unwired: 2 out]
            }
            n281 = Bundle By Name(cluster=w711, "Action"="Help") -> (w712:T14)
          }
          event "Power Down Info": Value Change {
            # "Generated when user clicks on 'Power Down Info' icon"
            n282 = event-data() -> ()  [unwired: 1 in, 1 out]
            n283 = for {
              tunnel: w725 -> [w730]
              shift-right: [w731] -> w726
              shift-left: w727 -> [w732]
              tunnel: string[] ["Hide Power Down Image"] -> [w728] mode=indexing
              n284 = Enqueue Element(queue=w730, element=w728, timeout in ms (-1)=50, error in (no error)=w732) -> (error out=w731:errorcluster)  [unwired: 2 out]
            }
            n285 = Bundle By Name(cluster=w723, "Action"="Power Down Help") -> (w724:T14)
          }
          event "Source Pin Seq": Mouse Up {
            # "ignore drop if mouse up happens out of bounds of listbox"
            # "#coercion dot"
            # "Generated when mouse press is released anywhere in 'Source Pin Seq'"
            n286 = event-data() -> ("CtlRef"=w746:refnum<vi>, "Coords"=w745:T16)  [unwired: 1 in]
            n287 = Unbundle By Name(w736) -> ("Seq Reorder.Drag?"=w735:bool)
            n288 = Enqueue Element(queue=w740, element="Check for valid pin re-order", timeout in ms (-1)=50, error in (no error)=w741) -> (error out=w739:errorcluster)  [unwired: 2 out]
            n289 = invoke on="Invoke Node" class="LstBox (strict)" method="Point To Row"(reference=w746, error in=w739, "Point"=w745) -> (error out=w744:errorcluster, "InBounds"=w734:bool, "Row"=w742:i32)  [unwired: 4 in, 4 out]
            n290 = Select(t=w735, s=w734, f=w734) -> (s? t:f=w733:bool)
            n291 = Bundle By Name(cluster=w736, "Seq Reorder.Drag?"=w733, "Seq Reorder.Drop Ind"=w742) -> (w743:T14)
          }
          event Mouse Down; Key Down {
            n292 = event-data() -> ()  [unwired: 1 in, 1 out]
            n293 = Unbundle By Name(w749) -> ("Indices.Selected Row"=w747:i32)
            n294 = Bundle By Name(cluster=w749, "Indices.Edit Pin Row"=w747) -> (w748:T14)
          }
          event Mouse Down {
            # "Generated when user clicks anywhere in the UI bounds"
            n295 = event-data() -> ("Coords.Horizontal"=w754:i32, "Coords.Vertical"=w752:i32)  [unwired: 1 in]
            n296 = for {
              tunnel: w756 -> [w762]
              shift-right: [w763] -> w757
              shift-left: w758 -> [w764]
              tunnel: string[] ["Click In Source Pin Sel?", "Click In Selection Icon?", "Check Hover Operations", "Check Pin Seq Drag", "Click in Info Icon?", "Click in PD Info Icon?", "Click in Plot Legend?"] -> [w760] mode=indexing
              n297 = Enqueue Element(queue=w762, element=w760, timeout in ms (-1)=50, error in (no error)=w764) -> (error out=w763:errorcluster)  [unwired: 2 out]
            }
            n298 = Bundle By Name(cluster=w759, "Action"="Help", "Coords.Mouse Coords.Horizontal"=w754, "Coords.Mouse Coords.Vertical"=w752) -> (w755:T14)
          }
          event Mouse Move {
            # "Generated when user moves the mouse anywhere in the UI bounds"
            n299 = event-data() -> ("Coords.Horizontal"=w767:i32, "Coords.Vertical"=w765:i32)  [unwired: 1 in]
            n300 = for {
              tunnel: w769 -> [w775]
              shift-right: [w776] -> w770
              shift-left: w771 -> [w777]
              tunnel: string[] ["Check Pin Seq Drag", "Check Hover Operations"] -> [w773] mode=indexing
              n301 = Enqueue Element(queue=w775, element=w773, timeout in ms (-1)=50, error in (no error)=w777) -> (error out=w776:errorcluster)  [unwired: 2 out]
            }
            n302 = Bundle By Name(cluster=w772, "Coords.Mouse Coords.Horizontal"=w767, "Coords.Mouse Coords.Vertical"=w765) -> (w768:T14)
          }
          event "Hover icon": Mouse Down {
            # "Generated when user clicks on black dropdown icon' to modify Source Pin"
            n303 = event-data() -> ("Coords.Horizontal"=w780:i32, "Coords.Vertical"=w778:i32)  [unwired: 1 in]
            n304 = Bundle By Name(cluster=w779, "Coords.Selection Coords.Horizontal"=w780, "Coords.Selection Coords.Vertical"=w778) -> (w781:T14)
            n305 = for {
              tunnel: w783 -> [w788]
              tunnel: string[] ["Hide Hover Icon", "Restore Cell Font Color", "Update Selected Row", "Check Empty Source Pin Seq", "Overlap Selection Pin List"] -> [w787] mode=indexing
              shift-right: [w789] -> w782
              shift-left: w784 -> [w790]
              n306 = Enqueue Element(queue=w788, element=w787, timeout in ms (-1)=50, error in (no error)=w790) -> (error out=w789:errorcluster)  [unwired: 2 out]
            }
          }
          event "Error Display": Double Click {
            # "Generated when user doubles clicks any error entry in 'Error Display'"
            n307 = event-data() -> ("Row"=w791:i32)  [unwired: 1 in]
            n308 = for {
              shift-right: [w801] -> w794
              shift-left: w797 -> [w802]
              tunnel: w796 -> [w800]
              tunnel: string[] ["Valid Error Navigation?"] -> [w799] mode=indexing
              n309 = Enqueue Element(queue=w800, element=w799, timeout in ms (-1)=50, error in (no error)=w802) -> (error out=w801:errorcluster)  [unwired: 2 out]
            }
            n310 = Bundle By Name(cluster=w795, "Indices.Error Db Clk Row"=w791) -> (w792:T14)
          }
          event "Power Down": Value Change {
            n311 = event-data() -> ("NewVal"=w803:bool)  [unwired: 1 in]
            n312 = local write "Quick Power Down"(w803) -> ()
            n313 = Bundle By Name(cluster=w805, "Pin Config.ML Config.Power Down"=w803) -> (w804:T14)
          }
          event "Voltage", "Current": Shortcut Menu Selection (User) {
            n314 = event-data() -> ("ItemTag"=w808:string, "CtlRef"=w809:refnum<vi>)  [unwired: 1 in]
            n315 = case shown="\"APP_SC_EXPORTDATATOCLIPBOARD\"" w808 {
              tunnel: w810 -> [w814 w815 w818]
              tunnel: [w813 w815 errorcluster {"status"=FALSE, "code"=0, "source"=""} ("error IO")] -> w807
              tunnel: w809 -> [w812 _ w817]
              frame "APP_SC_EXPORTDATATOCLIPBOARD" {
                n316 = invoke on="Invoke Node" class="WFGraph (strict)" method="Export Data to Clipboard"(reference=w812, error in=w814) -> (error out=w813:errorcluster)  [unwired: 1 in, 2 out]
              }
              frame "EXPORT", Default {
              }
              frame "APP_SC_EXPORTDATATOEXCEL" {
                n317 = invoke on="Invoke Node" class="WFGraph (strict)" method="Export Data to Excel"(reference=w817, error in=w818) -> ()  [unwired: 1 in, 3 out]
              }
            }
          }
          event Value Change {
            # "Update Error Display Scrollbar"
            # "Generated when user changes selected source pin configuration"
            n318 = event-data() -> ("NewVal"=w829:T5, "OldVal"=w828:T5)  [unwired: 1 in]
            n319 = Unbundle By Name(w822) -> ("Pin Config.Source Pin Config"=w820:T5[], "Indices.Edit Pin Row"=w834:i32)  [unwired: 1 out]
            n320 = expression code="x/2"(w834) -> (w819:i32)
            n321 = Replace Array Subset(array=w820, new element=w829, index=w819) -> (w833:T5[])
            n322 = Not Equal?(x=w829, y=w828) -> (x != y?=w827:T18)
            n323 = Cluster To Array(cluster=w827) -> (array=w826:bool[])
            n324 = Search 1D Array(1D array=w826, element=TRUE) -> (index of element=w824:i32)  [unwired: 1 in]
            n325 = case shown="6, 8" w824 {
              tunnel: [string[] ["Update Meas Config", "Validate Inputs", "Update Power Down", "Update Error Info", "Update Error Display Top Row", "Update Error Display Scrollbar"] string[] ["Check Limits", "Update Active Pin Config", "Update Meas Config", "Validate Inputs", "Update Error Info", "Update Error Display Scrollbar", "Update Power Down"] string[] []] -> w823
              frame 0..5, 7, 9..14 {
              }
              frame 6, 8 {
                # "6-Source Mode, 8-Default Ramp Rate"
              }
              frame Default {
              }
            }
            n326 = Bundle By Name(cluster=w822, "Pin Config.Source Pin Config"=w833, "Pin Config.Active Pin Config"=w829, "Flags.Check All?"=TRUE) -> (w835:T14)
            n327 = for {
              tunnel: w831 -> [w839]
              shift-right: [w837] -> w830
              shift-left: w832 -> [w840]
              tunnel: w823 -> [w836] mode=indexing
              n328 = Enqueue Element(queue=w839, element=w836, timeout in ms (-1)=50, error in (no error)=w840) -> (error out=w837:errorcluster)  [unwired: 2 out]
            }
          }
          event Panel Close? {
            # "Stop the application"
            n329 = event-data() -> ()  [unwired: 1 in, 1 out]
            n330 = Flush Queue(queue=w845, error in (no error)=w850) -> (queue out=w844:refnum<queue>, error out=w846:errorcluster)  [unwired: 1 out]
            n331 = Enqueue Element(queue=w844, element="Exit", error in (no error)=w846) -> (error out=w849:errorcluster)  [unwired: 1 in, 2 out]
            n332 = event-data ("Event Filter Node")("Discard?"=TRUE) -> ()  [unwired: 1 in, 1 out]
          }
        }
      }
      frame "--- Error Navigation Operations ---" {
      }
      frame "Valid Error Navigation?" {
        # "discard error column header click"
        # "Check if the double clicked row in 'Error Display' is in bounds"
        n333 = Unbundle By Name(w860) -> ("Indices.No.Errors"=w858:i32, "Indices.Error Db Clk Row"=w855:i32)
        n334 = Greater Or Equal To 0?(x=w855) -> (x >= 0?=w854:bool)
        n335 = Less Or Equal?(x=w858, y=w855) -> (x <= y?=w857:bool)
        n336 = Compound Arithmetic op=AND(invert w857, w854) -> (w856:bool)
        n337 = case shown="True" w856 {
          tunnel: w863 -> [w864 w868]
          tunnel: w862 -> [_ w867]
          tunnel: [w864 w866] -> w861
          tunnel: string[] ["Restore Previous to Default", "Restore Cell Font Color", "Error Navigation"] -> [_ w865]
          frame False {
            # "out of bounds - invalid"
          }
          frame True {
            # "in bounds - valid row"
            n338 = for {
              shift-right: [w872] -> w866
              shift-left: w868 -> [w873]
              tunnel: w867 -> [w871]
              tunnel: w865 -> [w870] mode=indexing
              n339 = Enqueue Element(queue=w871, element=w870, timeout in ms (-1)=50, error in (no error)=w873) -> (error out=w872:errorcluster)  [unwired: 2 out]
            }
          }
        }
      }
      frame "Error Navigation" {
        # "Navigate to the pin in the 'Source Pin Seq' whose error is double clicked in 'Error Display'"
        n340 = Unbundle By Name(w884) -> ("Flags.Visibilty.Scrollbar?"=w875:bool, "Pin Config.Error Ind"=w879:i32[], "Indices.Error Db Clk Row"=w876:i32, "Indices.Top Row"=w882:u32)
        n341 = Index Array(array=w879, index=w876) -> (element=w880:i32)
        n342 = property on="Error Display" class="MCListbox (strict)"(error in=w878, "Value"=w876) -> (error out=w877:errorcluster)  [unwired: 1 in, 1 out]
        n343 = expression code="x*2"(w880) -> (w874:i32)
        n344 = case shown="True" w875 {
          tunnel: w874 -> [_ w897]
          tunnel: w882 -> [w893 w895]
          tunnel: [w893 w894] -> w881
          frame False {
            # "scrollbar is invisble - so any error row selected will always be visible to user"
          }
          frame True {
            # "scrollbar is visible - so have to ensure the new selected pin is in visible range"
            n345 = To Unsigned Long Integer(number=w897) -> (unsigned 32bit integer=w896:u32)
            n346 = Greater?(x=w895, y=w896) -> (0:w898:bool)
            n347 = case shown="False" w898 {
              tunnel: w896 -> [w901 w905]
              tunnel: [w899 w905] -> w894
              tunnel: w895 -> [w902 _]
              frame False {
                # "False - selected row is hidden below the visible range\nTrue - selected row is in the visible range"
                n348 = expression code="x+16"(w902) -> (w904:u32)
                n349 = expression code="x-16"(w901) -> (w900:u32)
                n350 = Greater Or Equal?(x=w904, y=w901) -> (x >= y?=w903:bool)
                n351 = Select(t=w902, s=w903, f=w900) -> (s? t:f=w899:u32)
              }
              frame True {
                # "selected row is hidden above current top row - hence make the selected row the top row"
              }
            }
          }
        }
        n352 = for {
          shift-right: [w909] -> w886
          shift-left: w877 -> [w910]
          tunnel: w891 -> [w908]
          tunnel: string[] ["Hide Hover Icon", "Hide Reorder Hover Icon", "Hide Border", "Overlap White Dropdown", "Update Active Pin Config", "Re-Calculate Top Row", "Update Scrollbar", "Update UI"] -> [w907] mode=indexing
          n353 = Enqueue Element(queue=w908, element=w907, timeout in ms (-1)=50, error in (no error)=w910) -> (error out=w909:errorcluster)  [unwired: 2 out]
        }
        n354 = property on="Source Pin Seq" class="LstBox (strict)"(error in=w886, "Active Row"=w874) -> (error out=w885:errorcluster, "ActiveRowPosLeft"=w890:i32, "ActiveRowPosTop"=w888:i32)  [unwired: 1 in, 1 out]
        n355 = Quotient & Remainder(x=w874, y=2) -> (floor(x/y)=w887:i32)  [unwired: 1 out]
        n356 = Bundle By Name(cluster=w884, "Indices.Top Row"=w881, "Coords.Active Row Pos.Left"=w890, "Coords.Active Row Pos.Top"=w888, "Indices.Selected Row"=w874, "Indices.Edit Pin Row"=w874, "Indices.Actual Sel Row"=w887) -> (w883:T14)
      }
      frame "--- Advanced Settings  Operations ---" {
      }
      frame "Settings - Menu Selection(User)" {
        # "NOTE - DO NOT delete the property nodes in above cases. It impacts MeasLink framework\nconfiguration changes' detection!"
        # "Store the items selected from shortcut menu fo Settings icon"
        n357 = Unbundle By Name(w920) -> ("Adv Settings.Item Tag"=w919:string)
        n358 = case shown="\"User manual\"" w919 {
          selector: w919 -> [w924 w932 w943 _ _]
          tunnel: w920 -> [w928 w936 w945 w956 w967]
          tunnel: [w927 w935 w946 w956 w967] -> w918
          tunnel: w914 -> [w923 w931 w939 w955 w968]
          tunnel: [w922 w930 w938 w955 w964] -> w913
          frame "Freq_50 Hz" {
            w921 = T11 0 items=["50 Hz", "60 Hz"] ("Adv Setting.Power line frequency")
            # "Power line frequency - 50 Hz"
            n359 = Insert Into Array(array=string[] [], new element=w924) -> (w925:string[])  [unwired: 1 in]
            n360 = Bundle By Name(cluster=w928, "Adv Settings.Setting.Sel.PL_Freq"=w925, "Adv Settings.Adv Setting.Power line frequency"=w921) -> (w927:T14)
            n361 = property on="Power line frequency" class="Ring (strict)"(error in=w923, "Val(Sgnl)"=w921) -> (error out=w922:errorcluster)  [unwired: 1 in, 1 out]
          }
          frame "Freq_60 Hz" {
            w929 = T11 1 items=["50 Hz", "60 Hz"] ("Adv Setting.Power line frequency")
            # "Power line frequency - 60 Hz"
            n362 = Insert Into Array(array=string[] [], new element=w932) -> (w933:string[])  [unwired: 1 in]
            n363 = Bundle By Name(cluster=w936, "Adv Settings.Setting.Sel.PL_Freq"=w933, "Adv Settings.Adv Setting.Power line frequency"=w929) -> (w935:T14)
            n364 = property on="Power line frequency" class="Ring (strict)"(error in=w931, "Val(Sgnl)"=w929) -> (error out=w930:errorcluster)  [unwired: 1 in, 1 out]
          }
          frame "Capture data" {
            # "Capture data"
            n365 = Unbundle By Name(w945) -> ("Adv Settings.Setting.Sel.Main"=w944:string[])
            n366 = Search 1D Array(1D array=w944, element=w943) -> (index of element=w941:i32)  [unwired: 1 in]
            n367 = Greater Or Equal To 0?(x=w941) -> (x >= 0?=w942:bool)
            n368 = case shown="True" w942 {
              tunnel: w944 -> [w950 w954]
              tunnel: w943 -> [w949 _]
              tunnel: w941 -> [_ w953]
              tunnel: [w948 w952] -> w940
              tunnel: [TRUE ("Adv Setting.Data Capture") FALSE ("Adv Setting.Data Capture")] -> w937
              frame False {
                n369 = Insert Into Array(array=w950, new element=w949) -> (w948:string[])  [unwired: 1 in]
              }
              frame True {
                n370 = Delete From Array(array=w954, index=w953) -> (array with subset deleted=w952:string[])  [unwired: 1 in, 1 out]
              }
            }
            n371 = Bundle By Name(cluster=w945, "Adv Settings.Setting.Sel.Main"=w940, "Adv Settings.Adv Setting.Data Capture"=w937) -> (w946:T14)
            n372 = property on="Data Capture" class="Bool (strict)"(error in=w939, "Val(Sgnl)"=w937) -> (error out=w938:errorcluster)  [unwired: 1 in, 1 out]
          }
          frame Default {
          }
          frame "User manual" {
            # "Open DPSM user manual from target path based on runtime environment"
            n373 = Build Path(base path=path "C:/Users/Public/Documents/National Instruments/DPS", name or relative path="Device Power Sequencing Add-on for InstrumentStudio Beta User Manual.pdf") -> (appended path=w960:path)
            n374 = Path To String(path=w960) -> (string=w957:string)
            n375 = Concatenate Strings("cmd  /c \"", w957, "\"") -> (w963:string)
            n376 = call <vilib>:"System Exec.vi"("run minimized? (F)"=TRUE, "wait until completion? (T)"=FALSE, "error in (no error)"=w968, "command line"=w963) -> ("error out"=w964:errorcluster)  [unwired: 4 in, 3 out]
          }
        }
        n377 = Bundle By Name(cluster=w918, "Flags.Visibilty.Settings Icon"=FALSE, "Action"="Settings") -> (w917:T14)
      }
      frame Default {
      }
      frame "--- Panel Mouse Monitor Operations ---" {
      }
      frame "Click In Source Pin Sel?" {
        # "Check if the mouse click happened inside the 'Source Pin Selection'"
        # "Check mouse click co-ordinates to hide the 'Source Pin Selection' control"
        n378 = Unbundle By Name(w976) -> ("Flags.Visibilty.Pin Selection List"=w975:bool)
        n379 = case shown="True" w975 {
          tunnel: [TRUE w986] -> w973
          tunnel: w976 -> [_ w985]
          frame False {
          }
          frame True {
            # "Source Pin selection control is visible - hence check if mouse click is inside the control"
            n380 = Unbundle By Name(w985) -> ("Coords.Mouse Coords.Horizontal"=w980:i32, "Pin Selection.Dimensions.Width"=w984:i32, "Pin Selection.Dimensions.Left"=w983:i32, "Coords.Mouse Coords.Vertical"=w979:i32, "Pin Selection.Dimensions.Height"=w982:i32, "Pin Selection.Dimensions.Top"=w981:i32)
            n381 = Add(x=w982, y=w981) -> (x+y=w989:i32)
            n382 = Add(x=w984, y=w983) -> (x+y=w990:i32)
            n383 = In Range and Coerce(upper limit=w989, x=w979, lower limit=w981) -> (In Range?=w987:bool)  [unwired: 1 out]
            n384 = In Range and Coerce(upper limit=w990, x=w980, lower limit=w983) -> (In Range?=w988:bool)  [unwired: 1 out]
            n385 = Compound Arithmetic op=AND(w988, w987) -> (w986:bool)
          }
        }
        n386 = Bundle By Name(cluster=w976, "Flags.Mouse Down In Source Pin Seq?"=w973) -> (w974:T14)
      }
      frame "Click In Selection Icon?" {
        # "Objective - to hide 'Pin Selection List' control (checked in previous state(Click in Source Pin Sel?')\n upon mouse click anywhere outside of its bounds and 'Selection Icon' bounds"
        # "Check if the mouse click happened inside the 'Selection Icon'"
        # "Check mouse co-ordinates to hide the 'Source Pin Selection' control"
        n387 = Unbundle By Name(w991) -> ("Flags.Mouse Down In Source Pin Seq?"=w993:bool, "Flags.Visibilty.Selection Icon"=w995:bool, "Coords.Mouse Coords.Horizontal"=w997:i32, "Coords.Selection Icon.Width"=w1001:i32, "Coords.Selection Icon.Left"=w1000:i32, "Coords.Mouse Coords.Vertical"=w996:i32, "Coords.Selection Icon.Height"=w999:i32, "Coords.Selection Icon.Top"=w998:i32)
        n388 = case shown="True" w995 {
          tunnel: [TRUE w1016] -> w994
          tunnel: w1001 -> [_ w1011]
          tunnel: w1000 -> [_ w1010]
          tunnel: w999 -> [_ w1009]
          tunnel: w998 -> [_ w1008]
          tunnel: w997 -> [_ w1007]
          tunnel: w996 -> [_ w1006]
          frame False {
          }
          frame True {
            n389 = Add(x=w1009, y=w1008) -> (x+y=w1014:i32)
            n390 = Add(x=w1011, y=w1010) -> (x+y=w1015:i32)
            n391 = In Range and Coerce(upper limit=w1014, x=w1006, lower limit=w1008) -> (In Range?=w1012:bool)  [unwired: 1 out]
            n392 = In Range and Coerce(upper limit=w1015, x=w1007, lower limit=w1010) -> (In Range?=w1013:bool)  [unwired: 1 out]
            n393 = Compound Arithmetic op=AND(w1013, w1012) -> (w1016:bool)
          }
        }
        n394 = Compound Arithmetic op=AND(invert w993, invert w994) -> (w992:bool)
        n395 = case shown="True" w992 {
          tunnel: w1003 -> [w1017 w1022]
          tunnel: [w1017 w1021] -> w1004
          tunnel: w1002 -> [_ w1020]
          frame False {
          }
          frame True {
            # "outside listbox bounds\n- hide 'Pin Selection' control"
            n396 = Enqueue Element(queue=w1020, element="Hide Listbox", timeout in ms (-1)=50, error in (no error)=w1022) -> (error out=w1021:errorcluster)  [unwired: 2 out]
          }
        }
      }
      frame "Click in Info Icon?" {
        # "Check mouse click co-ordinates to hide the 'Image' control"
        n397 = Unbundle By Name(w1026) -> ("Flags.Visibilty.Help?"=w1028:bool, "Coords.Mouse Coords.Horizontal"=w1030:i32, "Coords.Info Icon.Width"=w1034:i32, "Coords.Info Icon.Left"=w1033:i32, "Coords.Mouse Coords.Vertical"=w1029:i32, "Coords.Info Icon.Height"=w1032:i32, "Coords.Info Icon.Top"=w1031:i32)
        n398 = case shown="True" w1028 {
          tunnel: [TRUE w1049] -> w1027
          tunnel: w1034 -> [_ w1044]
          tunnel: w1033 -> [_ w1043]
          tunnel: w1032 -> [_ w1042]
          tunnel: w1031 -> [_ w1041]
          tunnel: w1030 -> [_ w1040]
          tunnel: w1029 -> [_ w1039]
          frame False {
          }
          frame True {
            # "Info image is visible"
            n399 = Add(x=w1042, y=w1041) -> (x+y=w1047:i32)
            n400 = Add(x=w1044, y=w1043) -> (x+y=w1048:i32)
            n401 = In Range and Coerce(upper limit=w1047, x=w1039, lower limit=w1041) -> (In Range?=w1045:bool)  [unwired: 1 out]
            n402 = In Range and Coerce(upper limit=w1048, x=w1040, lower limit=w1043) -> (In Range?=w1046:bool)  [unwired: 1 out]
            n403 = Compound Arithmetic op=AND(w1046, w1045) -> (w1049:bool)
          }
        }
        n404 = case shown="False" w1027 {
          tunnel: w1036 -> [w1053 w1059]
          tunnel: [w1052 w1059] -> w1037
          tunnel: w1035 -> [w1051 _]
          tunnel: string[] ["Hide Image", "Update Icon State"] -> [w1050 _]
          frame False {
            # "outside Info icon bounds\n- hide 'Image' control"
            n405 = for {
              tunnel: w1051 -> [w1056]
              shift-right: [w1057] -> w1052
              shift-left: w1053 -> [w1058]
              tunnel: w1050 -> [w1054] mode=indexing
              n406 = Enqueue Element(queue=w1056, element=w1054, timeout in ms (-1)=50, error in (no error)=w1058) -> (error out=w1057:errorcluster)  [unwired: 2 out]
            }
          }
          frame True {
          }
        }
        n407 = Bundle By Name(cluster=w1026, "Action"="Help") -> (w1024:T14)
      }
      frame "Click in PD Info Icon?" {
        # "Check mouse click co-ordinates to hide the ' Power Down Image' control"
        n408 = Unbundle By Name(w1064) -> ("Action"=w1060:string, "Flags.Visibilty.PD Info"=w1066:bool, "Coords.Mouse Coords.Horizontal"=w1068:i32, "Coords.PDInfo Icon.Width"=w1072:i32, "Coords.PDInfo Icon.Left"=w1071:i32, "Coords.Mouse Coords.Vertical"=w1067:i32, "Coords.PDInfo Icon.Height"=w1070:i32, "Coords.PDInfo Icon.Top"=w1069:i32)
        n409 = case shown="True" w1066 {
          tunnel: [TRUE w1081] -> w1065
          tunnel: w1072 -> [_ w1087]
          tunnel: w1071 -> [_ w1086]
          tunnel: w1070 -> [_ w1085]
          tunnel: w1069 -> [_ w1084]
          tunnel: w1068 -> [_ w1083]
          tunnel: w1067 -> [_ w1082]
          tunnel: [w1076 w1078] -> w1061
          tunnel: w1060 -> [w1076 w1080]
          frame False {
          }
          frame True {
            # "Power Down Info image is visible"
            n410 = Add(x=w1085, y=w1084) -> (x+y=w1090:i32)
            n411 = Add(x=w1087, y=w1086) -> (x+y=w1091:i32)
            n412 = In Range and Coerce(upper limit=w1090, x=w1082, lower limit=w1084) -> (In Range?=w1088:bool)  [unwired: 1 out]
            n413 = In Range and Coerce(upper limit=w1091, x=w1083, lower limit=w1086) -> (In Range?=w1089:bool)  [unwired: 1 out]
            n414 = Compound Arithmetic op=AND(w1089, w1088) -> (w1081:bool)
            n415 = Select(t=w1080, s=w1081, f="Power Down Help" ("Action")) -> (s? t:f=w1078:string)
          }
        }
        n416 = case shown="False" w1065 {
          tunnel: w1074 -> [w1095 w1101]
          tunnel: [w1094 w1101] -> w1075
          tunnel: w1073 -> [w1093 _]
          tunnel: string[] ["Hide Power Down Image", "Update Icon State"] -> [w1092 _]
          frame False {
            # "outside Power Down Info icon bounds\n- hide ' Power Down Image' control"
            n417 = for {
              tunnel: w1093 -> [w1098]
              shift-right: [w1099] -> w1094
              shift-left: w1095 -> [w1100]
              tunnel: w1092 -> [w1096] mode=indexing
              n418 = Enqueue Element(queue=w1098, element=w1096, timeout in ms (-1)=50, error in (no error)=w1100) -> (error out=w1099:errorcluster)  [unwired: 2 out]
            }
          }
          frame True {
          }
        }
        n419 = Bundle By Name(cluster=w1064, "Action"=w1061) -> (w1062:T14)
      }
      frame "Click in Plot Legend?" {
        # "Check mouse co-ordinates to hide the 'Plot Legend' control"
        n420 = Unbundle By Name(w1106) -> ("Flags.Visibilty.Plot Legend"=w1107:bool, "Coords.Mouse Coords.Horizontal"=w1109:i32, "Coords.Plot Legend.Width"=w1113:i32, "Coords.Plot Legend.Left"=w1112:i32, "Coords.Mouse Coords.Vertical"=w1108:i32, "Coords.Plot Legend.Height"=w1111:i32, "Coords.Plot Legend.Top"=w1110:i32)
        n421 = case shown="True" w1107 {
          selector: w1107 -> [w1117 _]
          tunnel: [TRUE w1119] -> w1103
          tunnel: w1113 -> [_ w1125]
          tunnel: w1112 -> [_ w1124]
          tunnel: w1111 -> [_ w1123]
          tunnel: w1110 -> [_ w1122]
          tunnel: w1109 -> [_ w1121]
          tunnel: w1108 -> [_ w1120]
          tunnel: [w1117 w1119] -> w1102
          frame False {
          }
          frame True {
            # "Plot Legend is visible"
            n422 = Add(x=w1123, y=w1122) -> (x+y=w1128:i32)
            n423 = Add(x=w1125, y=w1124) -> (x+y=w1129:i32)
            n424 = In Range and Coerce(upper limit=w1128, x=w1120, lower limit=w1122) -> (In Range?=w1126:bool)  [unwired: 1 out]
            n425 = In Range and Coerce(upper limit=w1129, x=w1121, lower limit=w1124) -> (In Range?=w1127:bool)  [unwired: 1 out]
            n426 = Compound Arithmetic op=AND(w1127, w1126) -> (w1119:bool)
          }
        }
        n427 = case shown="False" w1103 {
          tunnel: w1115 -> [w1133 w1139]
          tunnel: [w1132 w1139] -> w1116
          tunnel: w1114 -> [w1131 _]
          tunnel: string[] ["Show/Hide Legend", "Update Icon State"] -> [w1130 _]
          frame False {
            # "outside Info icon bounds\n- hide 'Plot Legend' control"
            n428 = for {
              tunnel: w1131 -> [w1136]
              shift-right: [w1137] -> w1132
              shift-left: w1133 -> [w1138]
              tunnel: w1130 -> [w1134] mode=indexing
              n429 = Enqueue Element(queue=w1136, element=w1134, timeout in ms (-1)=50, error in (no error)=w1138) -> (error out=w1137:errorcluster)  [unwired: 2 out]
            }
          }
          frame True {
          }
        }
        n430 = Bundle By Name(cluster=w1106, "Flags.Visibilty.Plot Legend"=w1102) -> (w1104:T14)
      }
      frame "Check Pin Seq Drag" {
        # "Invalid - if mouse leaves bounds of Source Pin Seq control"
        # "Continuously check if Drag is valid in 'Source Pin Seq'"
        n431 = Unbundle By Name(w1154) -> ("Seq Reorder.Drag?"=w1144:bool, "Coords.Mouse Coords.Horizontal"=w1146:i32, "Coords.Source Pin Seq.Width"=w1150:i32, "Coords.Source Pin Seq.Left"=w1149:i32, "Coords.Mouse Coords.Vertical"=w1145:i32, "Coords.Source Pin Seq.Height"=w1148:i32, "Coords.Source Pin Seq.Top"=w1147:i32)
        n432 = Add(x=w1148, y=w1147) -> (x+y=w1151:i32)
        n433 = Add(x=w1150, y=w1149) -> (x+y=w1152:i32)
        n434 = In Range and Coerce(upper limit=w1151, x=w1145, lower limit=w1147) -> (In Range?=w1141:bool)  [unwired: 1 out]
        n435 = In Range and Coerce(upper limit=w1152, x=w1146, lower limit=w1149) -> (In Range?=w1142:bool)  [unwired: 1 out]
        n436 = Compound Arithmetic op=AND(w1144, w1142, w1141) -> (w1140:bool)
        n437 = Compound Arithmetic op=AND(w1142, w1141) -> (w1143:bool)
        n438 = Bundle By Name(cluster=w1154, "Seq Reorder.Drag?"=w1140, "Flags.Mouse Move In Source Pin Seq?"=w1143) -> (w1153:T14)
      }
      frame "Check Hover Operations" {
        # "Objective - Hide hover effects (if on) in 'Source Pin Seq' control once mouse leaves the control bounds"
        # "Check mouse co-ordinates to hide the 'Border' and 'Hover icon' controls"
        n439 = Unbundle By Name(w1164) -> ("Indices.Active Row"=w1159:i32, "Flags.Mouse Move In Source Pin Seq?"=w1160:bool, "Flags.Visibilty.Hover Icon"=w1163:bool, "Flags.Visibilty.Border"=w1162:bool, "Flags.Visibilty.Reorder Hover Icon"=w1156:bool)
        n440 = Compound Arithmetic op=AND(invert w1160, w1163, w1162, w1156) -> (w1161:bool)
        n441 = case shown="True" w1161 {
          tunnel: w1166 -> [w1169 w1174]
          tunnel: [w1169 w1173] -> w1167
          tunnel: w1165 -> [_ w1172]
          tunnel: w1159 -> [w1168 _]
          tunnel: [w1168 -1 ("Active Row")] -> w1157
          frame False {
          }
          frame True {
            # "Both 'Border' and 'Hover Icon' are visible - hide them"
            n442 = for {
              tunnel: w1172 -> [w1177]
              shift-right: [w1178] -> w1173
              shift-left: w1174 -> [w1179]
              tunnel: string[] ["Hide Hover Icon", "Hide Reorder Hover Icon", "Hide Border", "Restore Previous to Default"] -> [w1175] mode=indexing
              n443 = Enqueue Element(queue=w1177, element=w1175, timeout in ms (-1)=50, error in (no error)=w1179) -> (error out=w1178:errorcluster)  [unwired: 2 out]
            }
          }
        }
        n444 = Bundle By Name(cluster=w1164, "Indices.Active Row"=w1157) -> (w1158:T14)
      }
      frame "--- Hover Icon Selection Operations ---" {
      }
      frame "Update Selected Row" {
        n445 = Unbundle By Name(w1186) -> ("Indices.Active Row"=w1183:i32)
        n446 = Quotient & Remainder(x=w1183, y=2) -> (floor(x/y)=w1182:i32)  [unwired: 1 out]
        n447 = Bundle By Name(cluster=w1186, "Indices.Actual Sel Row"=w1182, "Indices.Selected Row"=w1183) -> (w1185:T14)
      }
      frame "Source Pin Sequence Common Operations ---" {
      }
      frame "Read Pin List" {
        # "Format Pin configuration as needed for display on UI in Source Pin Sequence"
        n448 = Unbundle By Name(w1196) -> ("Pins"=w1201:string[], "Indices.Row No Ref"=w1206:u32)
        n449 = Unbundle By Name(w1196) -> ("List Specs.Pin List"=w1202:string[], "List Specs.UI Pin List"=w1205:string[], "Pin Config.Error Info"=w1195:string[], "Pin Config.Error Ind"=w1192:i32[])
        n450 = for {
          tunnel: w1214 -> [w1227]
          tunnel: [w1218] -> w1213 mode=indexing
          tunnel: w1201 -> [w1229] mode=indexing
          tunnel: [w1226] -> w1204 mode=concatenating
          tunnel: [w1225] -> w1211
          tunnel: [w1223] -> w1209 mode=concatenating
          tunnel: [w1222] -> w1208 mode=concatenating
          tunnel: [w1221] -> w1207 mode=concatenating
          tunnel: w1206 -> [w1219]
          tunnel: ["" ("initial string")] -> w1194 mode=indexing
          tunnel: [0] -> w1190 mode=indexing
          i -> [w1224]
          # "for each pin in sequence"
          n451 = To Unsigned Long Integer(number=w1224) -> (unsigned 32bit integer=w1217:u32)
          n452 = Add(x=w1217, y=w1219) -> (x+y=w1220:u32)
          n453 = for {
            N: 2 -> [_]
            tunnel: w1229 -> [w1241]
            tunnel: [w1240] -> w1226 mode=indexing
            tunnel: w1220 -> [w1238]
            tunnel: [w1233] -> w1225
            tunnel: [w1233] -> w1223 mode=indexing
            tunnel: [w1232] -> w1222 mode=indexing
            tunnel: [w1231] -> w1221 mode=indexing
            tunnel: w1227 -> [w1242]
            tunnel: [w1235] -> w1230 mode=indexing
            i -> [w1239]
            # "for each row of a pin"
            n454 = case shown="0" w1239 {
              tunnel: w1242 -> [w1251 w1255 w1261]
              tunnel: [w1250 w1255 w1261] -> w1235
              tunnel: w1241 -> [w1248 _ _]
              tunnel: [w1246 "" ("Empty String Constant") "" ("Empty String Constant")] -> w1240
              tunnel: [u32 15460844 u32 0 u32 16777216] -> w1232
              tunnel: [47 0 3] -> w1231
              tunnel: [u32 0 u32 0 u32 1] -> w1234
              frame 0 {
                # "pin row"
                n455 = Format Into String(format string="\n      %s\n", initial string="", error in=w1251, w1248) -> (resulting string=w1246:string, error out=w1250:errorcluster)
              }
              frame Default {
                # "empty row"
              }
              frame 1 {
                # "invalid scenario"
              }
            }
            n456 = Multiply(x=w1238, y=u32 2 ("x")) -> (x*y=w1237:u32)
            n457 = Add(x=w1234, y=w1237) -> (x+y=w1233:u32)
          }
          n458 = Merge Errors(w1230) -> (w1218:errorcluster)
        }
        n459 = expression code="x==0 ? 0:x+1"(w1211) -> (w1210:u32)
        n460 = Build Array (concatenate)(w1202, w1201) -> (w1200:string[])
        n461 = Build Array (concatenate)(w1205, w1204) -> (w1203:string[])
        n462 = Build Array (concatenate)(w1195, w1194) -> (w1193:string[])
        n463 = Build Array (concatenate)(w1192, w1190) -> (w1191:i32[])
        n464 = Array Size(array=w1200) -> (size(s)=w1199:i32)
        n465 = To Unsigned Long Integer(number=w1199) -> (unsigned 32bit integer=w1197:u32)
        n466 = Merge Errors(w1213) -> (w1198:errorcluster)
        n467 = Bundle By Name(cluster=w1196, "Indices.Row No Ref"=w1197, "List Specs.Pin List"=w1200, "List Specs.UI Pin List"=w1203, "Pin Config.Error Info"=w1193, "Pin Config.Error Ind"=w1191, "#Rows"=w1210, "List Specs.Active Row Nos"=w1209, "List Specs.CellBG"=w1208, "List Specs.Cell Height"=w1207) -> (w1212:T14)
      }
      frame "Restore Previous to Default" {
        # "Restore CellBG color of 'Source Pin Sequence' of previously active row"
        n468 = Unbundle By Name(w1271) -> ("Indices.Last Active Row"=w1268:i32)
        n469 = Quotient & Remainder(x=w1268, y=2) -> (x-y*floor(x/y)=w1265:i32)  [unwired: 1 out]
        n470 = Equal To 0?(x=w1265) -> (x = 0?=w1266:bool)
        n471 = Select(t=u32 15460844, s=w1266, f=u32 16777216) -> (s? t:f=w1262:u32)
        n472 = property on="Source Pin Seq" class="LstBox (strict)"(error in=w1269, "Active Row"=w1268, "CellBG"=w1262) -> (error out=w1270:errorcluster)  [unwired: 1 in, 1 out]
      }
      frame "Restore Cell Font Color" {
        # "Restore CellBG color of 'Source Pin Sequence' of previously selected row"
        n473 = Unbundle By Name(w1284) -> ("Indices.Last Active Row"=w1281:i32, "Indices.Selected Row"=w1272:i32)
        n474 = Quotient & Remainder(x=w1281, y=2) -> (x-y*floor(x/y)=w1278:i32)  [unwired: 1 out]
        n475 = Equal To 0?(x=w1278) -> (x = 0?=w1279:bool)
        n476 = Select(t=u32 15460844, s=w1279, f=u32 16777216) -> (s? t:f=w1275:u32)
        n477 = property on="Source Pin Seq" class="LstBox (strict)"(error in=w1282, "Active Row"=w1281, "CellBG"=w1275, "CellFontColor"=u32 0 ("Active Row:Cell Font:Color"), "Active Row"=w1272, "CellFontColor"=u32 0 ("Active Row:Cell Font:Color")) -> (error out=w1283:errorcluster)  [unwired: 1 in, 1 out]
      }
      frame "--- Source Pin Sequence Mouse Down Operations ---" {
      }
      frame "Check Empty Source Pin Seq" {
        # "Check if Source Pin Sequence is empty"
        n478 = Unbundle By Name(w1290) -> ("#Rows"=w1289:u32)
        n479 = case shown="1.." w1289 {
          tunnel: w1291 -> [w1292 w1295]
          tunnel: w1288 -> [_ w1294]
          tunnel: [w1292 w1293] -> w1287
          frame 0 {
          }
          frame 1.. {
            # "non-empty Source Pin Sequence"
            n480 = for {
              shift-right: [w1300] -> w1293
              shift-left: w1295 -> [w1301]
              tunnel: w1294 -> [w1299]
              tunnel: string[] ["Get Mouse Down Info", "Get Mouse Down Row Info"] -> [w1298] mode=indexing
              n481 = Enqueue Element(queue=w1299, element=w1298, timeout in ms (-1)=50, error in (no error)=w1301) -> (error out=w1300:errorcluster)  [unwired: 2 out]
            }
          }
        }
      }
      frame "Get Mouse Down Info" {
        # "#coercion dot"
        # "Get selected row number of 'Source Pin Seq'"
        n482 = Unbundle By Name(w1309) -> ("Coords.Selection Coords"=w1308:cluster{"Horizontal":i32, "Vertical":i32})
        n483 = invoke on="Source Pin Seq" class="LstBox (strict)" method="Point To Row"(error in=w1311, "Point"=w1308) -> (error out=w1303:errorcluster, "Row"=w1306:i32)  [unwired: 5 in, 5 out]
        n484 = Quotient & Remainder(x=w1306, y=2) -> (x-y*floor(x/y)=w1304:i32, floor(x/y)=w1305:i32)
        n485 = case shown="0" w1304 {
          tunnel: [w1313 w1318] -> w1310
          tunnel: w1309 -> [w1313 w1317]
          tunnel: w1306 -> [_ w1316]
          tunnel: w1305 -> [_ w1315]
          tunnel: w1303 -> [w1312 w1314]
          tunnel: [w1312 w1314] -> w1302
          frame 1, Default {
          }
          frame 0 {
            n486 = Bundle By Name(cluster=w1317, "Seq Reorder.Drag Ind"=w1316, "Indices.Selected Row"=w1316, "Indices.Actual Sel Row"=w1315) -> (w1318:T14)
          }
        }
      }
      frame "Get Mouse Down Row Info" {
        # "Get selected row co-ordinates in 'Source Pin Seq'"
        n487 = Unbundle By Name(w1322) -> ("Indices.Selected Row"=w1321:i32)
        n488 = property on="Source Pin Seq" class="LstBox (strict)"(error in=w1329, "Active Row"=w1321) -> (error out=w1324:errorcluster, "ActiveRowPosLeft"=w1326:i32, "ActiveRowPosTop"=w1323:i32)  [unwired: 1 in, 1 out]
        n489 = Quotient & Remainder(x=w1321, y=2) -> (x-y*floor(x/y)=w1320:i32, floor(x/y)=w1319:i32)
        n490 = case shown="0" w1320 {
          tunnel: w1324 -> [w1331 w1332 w1335]
          tunnel: [w1331 w1332 w1334] -> w1330
          tunnel: w1328 -> [_ _ w1333]
          frame 1 {
          }
          frame Default {
          }
          frame 0 {
            n491 = for {
              shift-right: [w1340] -> w1334
              shift-left: w1335 -> [w1341]
              tunnel: w1333 -> [w1339]
              tunnel: string[] ["Hide Hover Icon", "Hide Reorder Hover Icon", "Hide Border", "Restore Previous to Default", "Overlap White Dropdown", "Check Limits", "Update Active Pin Config", "Update Meas Config", "Validate Inputs", "Update Error Info", "Update Error Display Top Row", "Update Error Display Scrollbar"] -> [w1338] mode=indexing
              n492 = Enqueue Element(queue=w1339, element=w1338, timeout in ms (-1)=50, error in (no error)=w1341) -> (error out=w1340:errorcluster)  [unwired: 2 out]
            }
          }
        }
        n493 = Bundle By Name(cluster=w1322, "Coords.Active Row Pos.Left"=w1326, "Coords.Active Row Pos.Top"=w1323, "Indices.Selected Row"=w1321, "Indices.Actual Sel Row"=w1319) -> (w1327:T14)
      }
      frame "Check Hide/Unhide Listbox" {
        # "Triggered when user clicks on selection dropdown icon on selected row in Source Pin Seq"
        # "Check if Pin Selection List has to be shown or hidden"
        n494 = Unbundle By Name(w1344) -> ("Flags.Visibilty.Pin Selection List"=w1343:bool)
        n495 = case shown="False" w1343 {
          tunnel: [string[] ["Check Empty Source Pin Seq", "Overlap Selection Pin List"] string[] ["Hide Listbox"]] -> w1342
          frame False {
            # "Hidden - so show it below selected pin"
          }
          frame True {
            # "Already visible - so hide it"
          }
        }
        n496 = for {
          shift-right: [w1353] -> w1345
          shift-left: w1347 -> [w1354]
          tunnel: w1346 -> [w1352]
          tunnel: w1342 -> [w1351] mode=indexing
          n497 = Enqueue Element(queue=w1352, element=w1351, timeout in ms (-1)=50, error in (no error)=w1354) -> (error out=w1353:errorcluster)  [unwired: 2 out]
        }
      }
      frame "Overlap White Dropdown" {
        # "Update CellBG color and display 'Selection icon' on the selected row in 'Source Pin Seq'"
        n498 = Unbundle By Name(w1367) -> ("Coords.List Coords.Icon Left"=w1359:i32, "Coords.List Coords.Icon Top Offset"=w1358:i32, "Indices.Selected Row"=w1363:i32, "Coords.Active Row Pos"=w1361:cluster{"Left":i32, "Top":i32})
        n499 = Quotient & Remainder(x=w1363, y=2) -> (x-y*floor(x/y)=w1364:i32, floor(x/y)=w1360:i32)
        n500 = case shown="0" w1364 {
          tunnel: w1362 -> [w1379 w1380 w1381]
          tunnel: w1363 -> [w1371 _ _]
          tunnel: [w1375 w1380 w1381] -> w1368
          tunnel: w1361 -> [w1377 _ _]
          tunnel: w1360 -> [_ _ _]
          tunnel: w1359 -> [w1370 _ _]
          tunnel: w1358 -> [w1374 _ _]
          tunnel: [w1370 _ _] -> w1356
          tunnel: [w1369 _ _] -> w1355
          frame 0 {
            # "valid pin row"
            n501 = property on="Source Pin Seq" class="LstBox (strict)"(error in=w1379, "Active Row"=w1371, "CellBG"=u32 15460844 ("Active Row:Cell Font:Color"), "CellFontColor"=u32 16448250 ("Active Row:Cell Font:Color"), "Value"=w1371) -> (error out=w1378:errorcluster)  [unwired: 1 in, 1 out]
            n502 = Unbundle By Name(w1377) -> ("Top"=w1373:i32)  [unwired: 1 out]
            n503 = Add(x=w1374, y=w1373) -> (x+y=w1369:i32)
            n504 = property on="Selection icon" class="Bool (strict)"(error in=w1378, "Left"=w1370, "Top"=w1369) -> (error out=w1375:errorcluster)  [unwired: 1 in, 1 out]
          }
          frame 1 {
            # "empty row"
          }
          frame Default {
          }
        }
        n505 = Bundle By Name(cluster=w1367, "Flags.Visibilty.Selection Icon"=TRUE ("Visibilty.Selection Icon"), "Indices.Last Active Row"=w1363, "Coords.Selection Icon.Left"=w1356, "Coords.Selection Icon.Top"=w1355) -> (w1366:T14)
      }
      frame "Overlap Selection Pin List" {
        # "ensure then selected pin in seq is selected row (tickmark itemname) in Pin Selection List\nand in visible range to user"
        # "Overlap the Pin Selection control beneath selected row in 'Source Pin Seq'"
        n506 = Unbundle By Name(w1395) -> ("Pin Symbols"=w1382:i32[], "Pinmap List"=w1383:string[], "List Specs.Pin List"=w1391:string[], "Indices.Selected Row"=w1390:i32, "Coords.Active Row Pos"=w1388:cluster{"Left":i32, "Top":i32})
        n507 = Quotient & Remainder(x=w1390, y=2) -> (x-y*floor(x/y)=w1392:i32, floor(x/y)=w1387:i32)
        n508 = case shown="0" w1392 {
          tunnel: w1389 -> [w1415 w1416 w1417]
          tunnel: w1390 -> [_ _ _]
          tunnel: [w1413 w1416 w1417] -> w1396
          tunnel: w1388 -> [w1414 _ _]
          tunnel: w1391 -> [w1406 _ _]
          tunnel: w1387 -> [w1405 _ _]
          tunnel: [w1411 _ _] -> w1385
          tunnel: [w1410 _ _] -> w1384
          tunnel: w1383 -> [w1404 _ _]
          tunnel: w1382 -> [w1402 _ _]
          frame 0 {
            # "valid pin row"
            n509 = Index Array(array=w1406, index=w1405) -> (element=w1403:string)
            n510 = Search 1D Array(1D array=w1404, element=w1403) -> (index of element=w1399:i32)  [unwired: 1 in]
            n511 = expression code="x>6? x-6:0"(w1399) -> (w1398:i32)
            n512 = Unbundle By Name(w1414) -> ("Left"=w1411:i32, "Top"=w1412:i32)
            n513 = Replace Array Subset(array=w1402, new element=1, index=w1399) -> (w1400:i32[])
            n514 = expression code="x+47"(w1412) -> (w1410:i32)
            n515 = property on="Pin Selection" class="LstBox (strict)"(error in=w1415, "Item Symbols"=w1400, "Value"=-1 ("Pin Selection"), "Left"=w1411, "Top"=w1410, "Top Row"=w1398, "Active Row"=-2 ("Active Row:Active Row Number"), "CellBG"=u32 16448250 ("Active Row:Cell Font:Color"), "CellFontColor"=u32 0 ("Active Row:Cell Font:Color")) -> (error out=w1413:errorcluster)  [unwired: 1 in, 1 out]
          }
          frame 1 {
            # "empty row"
          }
          frame Default {
          }
        }
        n516 = Bundle By Name(cluster=w1395, "Flags.Visibilty.Pin Selection List"=TRUE ("Visibilty.Pin Selection List"), "Indices.Last Active Row"=w1390, "Pin Selection.Dimensions.Left"=w1385, "Pin Selection.Dimensions.Top"=w1384) -> (w1394:T14)
      }
      frame "--- Source Pin Sequence Mouse Hover Operations ---" {
      }
      frame "Check Scroll Direction" {
        # "Compare consecutive mouse positions in 'Source Pin Seq' to determine the direction of drag and drop operation"
        n517 = Unbundle By Name(w1425) -> ("Coords.Hover Coords.Vertical"=w1424:i32, "Coords.Hover Coords Old.Vertical"=w1423:i32, "Coords.Hover Coords"=w1420:cluster{"Horizontal":i32, "Vertical":i32})
        n518 = Less Or Equal?(x=w1424, y=w1423) -> (x <= y?=w1421:bool)
        n519 = Bundle By Name(cluster=w1425, "Seq Reorder.Up?"=w1421, "Coords.Hover Coords Old"=w1420) -> (w1422:T14)
      }
      frame "Check Scroll for Reordering" {
        # "#coercion dot"
        # "True - Move top row higher until first pin is top row\nFalse - active row is in visble range, so do nothing"
        # "True - two scenarios\n     True - already the last pin in seq is visible, so do nothing\n      False - move top row a level bottom \nFalse - active row is in visble range, so do nothing"
        # "Create auto-scroll effect in 'Source Pin Seq' as user performs drag and drop operation"
        n520 = Unbundle By Name(w1440) -> ("Seq Reorder.Up?"=w1429:bool, "#Rows"=w1443:u32, "Seq Reorder.Drag?"=w1433:bool, "Flags.Visibilty.Scrollbar?"=w1430:bool, "Seq Reorder.Drag Ind"=w1447:i32, "Indices.Top Row"=w1445:u32, "Coords.Hover Coords"=w1438:cluster{"Horizontal":i32, "Vertical":i32})
        n521 = invoke on="Source Pin Seq" class="LstBox (strict)" method="Point To Row"(error in=w1437, "Point"=w1438) -> (error out=w1436:errorcluster, "InBounds"=w1427:bool, "Row"=w1435:i32)  [unwired: 5 in, 4 out]
        n522 = Compound Arithmetic op=AND(w1433, w1430) -> (w1431:bool)
        n523 = Less Or Equal?(x=w1447, y=w1435) -> (x <= y?=w1446:bool)
        n524 = To Unsigned Long Integer(number=w1435) -> (unsigned 32bit integer=w1434:u32)
        n525 = case shown="True" w1431 {
          tunnel: w1446 -> [_ _]
          tunnel: w1445 -> [w1455 w1461]
          tunnel: w1434 -> [_ w1460]
          tunnel: [w1455 w1459] -> w1444
          tunnel: w1443 -> [_ w1458]
          tunnel: [FALSE w1457] -> w1432
          tunnel: w1429 -> [_ w1456]
          frame False {
            # "scrollbar is hidden - no auto-scroll needed"
          }
          frame True {
            # "scrollbar is visible - hence check for autoscroll"
            n526 = case shown="True" w1456 {
              tunnel: w1461 -> [w1464 w1475]
              tunnel: w1460 -> [w1470 w1476]
              tunnel: [w1469 w1473] -> w1459
              tunnel: w1458 -> [w1468 _]
              tunnel: [w1462 w1472] -> w1457
              frame False {
                # "drag down"
                n527 = expression code="x+18"(w1464) -> (w1463:u32)
                n528 = expression code="x+2"(w1464) -> (w1466:u32)
                n529 = expression code="x+16"(w1464) -> (w1471:u32)
                n530 = Greater Or Equal?(x=w1463, y=w1468) -> (x >= y?=w1467:bool)
                n531 = Greater Or Equal?(x=w1470, y=w1471) -> (x >= y?=w1462:bool)
                n532 = Select(t=w1464, s=w1467, f=w1466) -> (s? t:f=w1465:u32)
                n533 = Select(t=w1465, s=w1462, f=w1464) -> (s? t:f=w1469:u32)
              }
              frame True {
                # "drag up"
                n534 = expression code="x>0?x-2:0"(w1475) -> (w1474:u32)
                n535 = Greater Or Equal?(x=w1475, y=w1476) -> (x >= y?=w1472:bool)
                n536 = Select(t=w1474, s=w1472, f=w1475) -> (s? t:f=w1473:u32)
              }
            }
          }
        }
        n537 = Compound Arithmetic op=AND(w1432, w1427) -> (w1428:bool)
        n538 = Bundle By Name(cluster=w1440, "Indices.Top Row"=w1444) -> (w1439:T14)
        n539 = case shown="True" w1428 {
          tunnel: w1441 -> [_ w1453]
          tunnel: w1436 -> [w1448 w1452]
          tunnel: [w1448 w1451] -> w1442
          frame False {
          }
          frame True {
            n540 = Enqueue Element(queue=w1453, element="Update Scrollbar", timeout in ms (-1)=50, error in (no error)=w1452) -> (error out=w1451:errorcluster)  [unwired: 2 out]
          }
        }
      }
      frame "Reposition White Dropdown" {
        # "When user is dragging in pin sequence and scrollbar is visible, the white drpdown icon in selected row has to be moved as\nwe auto-scroll seq up/down"
        # "Move selection dropdown icon as we auto-scroll pin seq for drag and drop"
        n541 = Unbundle By Name(w1485) -> ("Coords.List Coords.Icon Left"=w1482:i32, "Coords.List Coords.Icon Top Offset"=w1481:i32, "Indices.Selected Row"=w1480:i32, "Seq Reorder.Drag?"=w1479:bool, "Flags.Visibilty.Scrollbar?"=w1477:bool)
        n542 = Compound Arithmetic op=AND(w1479, w1477) -> (w1478:bool)
        n543 = case shown="True" w1478 {
          tunnel: [w1487 w1504] -> w1486
          tunnel: w1485 -> [w1488 w1503]
          tunnel: [w1488 w1502] -> w1484
          tunnel: w1483 -> [w1487 w1492]
          tunnel: w1482 -> [_ w1498]
          tunnel: w1481 -> [_ w1497]
          tunnel: w1480 -> [_ w1493]
          frame False {
          }
          frame True {
            n544 = property on="Source Pin Seq" class="LstBox (strict)"(error in=w1492, "Active Row"=w1493) -> (error out=w1491:errorcluster, "ActiveRowPosLeft"=w1489:i32, "ActiveRowPosTop"=w1490:i32)  [unwired: 1 in, 1 out]
            n545 = Quotient & Remainder(x=w1493, y=2) -> (x-y*floor(x/y)=w1500:i32, floor(x/y)=w1499:i32)
            n546 = case shown="0" w1500 {
              tunnel: w1491 -> [w1510 w1511 w1512]
              tunnel: w1493 -> [_ _ _]
              tunnel: [w1509 w1511 w1512] -> w1504
              tunnel: w1499 -> [_ _ _]
              tunnel: w1498 -> [w1507 _ _]
              tunnel: w1497 -> [w1508 _ _]
              tunnel: [w1507 _ _] -> w1495
              tunnel: [w1506 _ _] -> w1494
              tunnel: w1490 -> [w1505 _ _]
              frame 0 {
                # "valid pin row"
                n547 = Add(x=w1508, y=w1505) -> (x+y=w1506:i32)
                n548 = property on="Selection icon" class="Bool (strict)"(error in=w1510, "Left"=w1507, "Top"=w1506) -> (error out=w1509:errorcluster)  [unwired: 1 in, 1 out]
              }
              frame 1 {
                # "empty row"
              }
              frame Default {
              }
            }
            n549 = Bundle By Name(cluster=w1503, "Coords.Active Row Pos.Left"=w1489, "Coords.Active Row Pos.Top"=w1490, "Flags.Visibilty.Selection Icon"=TRUE ("Visibilty.Selection Icon"), "Coords.Selection Icon.Left"=w1495, "Coords.Selection Icon.Top"=w1494) -> (w1502:T14)
          }
        }
      }
      frame "Get Mouse Hover Info" {
        # "#coercion dot"
        # "Get hover row number of 'Source Pin Seq'"
        n550 = Unbundle By Name(w1518) -> ("Indices.Active Row"=w1516:i32, "Coords.Hover Coords"=w1517:cluster{"Horizontal":i32, "Vertical":i32})
        n551 = invoke on="Source Pin Seq" class="LstBox (strict)" method="Point To Row"(error in=w1521, "Point"=w1517) -> (error out=w1519:errorcluster, "Row"=w1515:i32)  [unwired: 5 in, 5 out]
        n552 = Quotient & Remainder(x=w1515, y=2) -> (x-y*floor(x/y)=w1513:i32)  [unwired: 1 out]
        n553 = case shown="0" w1513 {
          tunnel: [w1531 w1535 w1536] -> w1522
          tunnel: [w1530 w1532 w1537] -> w1520
          tunnel: w1519 -> [w1528 w1535 w1536]
          tunnel: w1518 -> [w1526 w1533 w1537]
          tunnel: w1516 -> [w1525 _ _]
          tunnel: w1515 -> [w1524 w1534 _]
          frame 0 {
            # "valid pin row"
            n554 = Equal?(x=w1525, y=w1524) -> (x = y?=w1523:bool)
            n555 = property on="Source Pin Seq" class="LstBox (strict)"(error in=w1528, "Active Row"=w1524) -> (error out=w1531:errorcluster, "ActiveRowPosLeft"=w1529:i32, "ActiveRowPosTop"=w1527:i32)  [unwired: 1 in, 1 out]
            n556 = Bundle By Name(cluster=w1526, "Flags.Same Hover Row?"=w1523, "Coords.Active Row Pos.Left"=w1529, "Coords.Active Row Pos.Top"=w1527, "Indices.Active Row"=w1524) -> (w1530:T14)
          }
          frame 1 {
            # "empty row"
            n557 = Bundle By Name(cluster=w1533, "Indices.Active Row"=w1534) -> (w1532:T14)
          }
          frame Default {
          }
        }
      }
      frame "Check Hover Action" {
        # "NOTE: Do not create hover effect if the hover row is already selected"
        # "Check for non-empty 'Source Pin Seq' to create hover effect"
        n558 = Unbundle By Name(w1545) -> ("#Rows"=w1540:u32, "Flags.Same Hover Row?"=w1541:bool, "Indices.Active Row"=w1543:i32, "Indices.Selected Row"=w1544:i32)
        n559 = Greater Than 0?(x=w1540) -> (x > 0?=w1539:bool)
        n560 = Not Equal?(x=w1543, y=w1544) -> (x != y?=w1538:bool)
        n561 = Compound Arithmetic op=AND(w1539, invert w1541, w1538) -> (w1542:bool)
        n562 = case shown="True" w1542 {
          tunnel: w1548 -> [w1551 w1566]
          tunnel: w1547 -> [w1552 w1565]
          tunnel: [w1550 w1564] -> w1546
          tunnel: w1538 -> [w1549 _]
          frame False {
            n563 = case shown="False" w1549 {
              tunnel: w1552 -> [w1555 _]
              tunnel: w1551 -> [w1554 w1562]
              tunnel: [w1553 w1562] -> w1550
              frame False {
                # "hide hover effects"
                n564 = for {
                  shift-right: [w1560] -> w1553
                  shift-left: w1554 -> [w1561]
                  tunnel: w1555 -> [w1559]
                  tunnel: string[] ["Restore Previous to Default", "Hide Border", "Hide Hover Icon", "Hide Reorder Hover Icon"] -> [w1558] mode=indexing
                  n565 = Enqueue Element(queue=w1559, element=w1558, timeout in ms (-1)=50, error in (no error)=w1561) -> (error out=w1560:errorcluster)  [unwired: 2 out]
                }
              }
              frame True {
              }
            }
          }
          frame True {
            # "Valid hover action"
            n566 = for {
              shift-right: [w1570] -> w1564
              shift-left: w1566 -> [w1571]
              tunnel: w1565 -> [w1569]
              tunnel: string[] ["Restore Previous to Default", "Hover in pin list", "Reposition White Dropdown"] -> [w1568] mode=indexing
              n567 = Enqueue Element(queue=w1569, element=w1568, timeout in ms (-1)=50, error in (no error)=w1571) -> (error out=w1570:errorcluster)  [unwired: 2 out]
            }
          }
        }
      }
      frame "Hover in pin list" {
        w1575 = TRUE ("Visibilty.Hover Icon")
        # "Update CellBG color and display Hover icon' + 'Border' control on the hover row in 'Source Pin Seq'"
        n568 = Unbundle By Name(w1585) -> ("Coords.List Coords.Reorder Icon Left"=w1574:i32, "Coords.List Coords.Reorder Icon Top Offset"=w1573:i32, "Coords.List Coords.Icon Left"=w1577:i32, "Coords.List Coords.Icon Top Offset"=w1576:i32, "Coords.Active Row Pos"=w1578:cluster{"Left":i32, "Top":i32}, "Indices.Active Row"=w1581:i32, "Indices.Top Row"=w1572:u32, "Coords.Border Left"=w1579:i32)
        n569 = Quotient & Remainder(x=w1581, y=2) -> (x-y*floor(x/y)=w1582:i32)  [unwired: 1 out]
        n570 = Bundle By Name(cluster=w1585, "Flags.Visibilty.Reorder Hover Icon"=w1575, "Flags.Visibilty.Border"=w1575, "Flags.Visibilty.Hover Icon"=w1575, "Indices.Last Active Row"=w1581) -> (w1584:T14)
        n571 = case shown="Default" w1582 {
          tunnel: w1580 -> [w1615 w1623 w1624]
          tunnel: w1581 -> [w1593 _ _]
          tunnel: [w1612 w1623 w1624] -> w1586
          tunnel: w1579 -> [w1608 _ _]
          tunnel: w1578 -> [w1603 _ _]
          tunnel: w1577 -> [w1602 _ _]
          tunnel: w1576 -> [w1601 _ _]
          tunnel: w1574 -> [w1597 _ _]
          tunnel: w1573 -> [w1596 _ _]
          tunnel: w1572 -> [w1594 _ _]
          frame 0 {
            # "valid pin row"
            n572 = Decrement(x=w1593) -> (x-1=w1606:i32)
            n573 = Not Equal To 0?(x=w1593) -> (x != 0?=w1592:bool)
            n574 = To Long Integer(number=w1594) -> (32bit integer=w1587:i32)
            n575 = Select(t=w1606, s=w1592, f=0) -> (s? t:f=w1604:i32)
            n576 = Equal?(x=w1593, y=w1587) -> (x = y?=w1591:bool)
            n577 = Unbundle By Name(w1603) -> ("Top"=w1588:i32)
            n578 = property on="Source Pin Seq" class="LstBox (strict)"(error in=w1615, "Active Row"=w1593, "CellBG"=u32 16448250 ("Active Row:Cell Font:Color"), "CellFontColor"=u32 0 ("Active Row:Cell Font:Color"), "Active Row"=w1604) -> (error out=w1614:errorcluster, "ActiveRowPosTop"=w1607:i32)  [unwired: 1 in, 1 out]
            n579 = Build Array(w1592, w1591) -> (w1590:bool[])
            n580 = Boolean Array To Number(Boolean array=w1590) -> (number=w1589:u32)
            n581 = Add(x=w1601, y=w1588) -> (x+y=w1600:i32)
            n582 = case shown="0, Default" w1589 {
              tunnel: [w1616 w1619 w1621] -> w1609
              tunnel: w1607 -> [w1617 w1618 _]
              tunnel: w1588 -> [_ _ w1622]
              frame 0, Default {
                n583 = Decrement(x=w1617) -> (x-1=w1616:i32)
              }
              frame 1 {
                n584 = Add(x=3, y=w1618) -> (x+y=w1619:i32)
              }
              frame 3 {
                n585 = Decrement(x=w1622) -> (x-1=w1621:i32)
              }
            }
            n586 = property on="Hover icon" class="Bool (strict)"(error in=w1614, "Left"=w1602, "Top"=w1600) -> (error out=w1599:errorcluster)  [unwired: 1 in, 1 out]
            n587 = Add(x=w1596, y=w1588) -> (x+y=w1595:i32)
            n588 = property on="Reorder Hover Icon" class="Bool (strict)"(error in=w1599, "Left"=w1597, "Top"=w1595) -> (error out=w1598:errorcluster)  [unwired: 1 in, 1 out]
            n589 = property on="Border" class="Str"(error in=w1598, "Top"=w1609, "Left"=w1608, "Visible"=TRUE) -> (error out=w1612:errorcluster)  [unwired: 1 in, 1 out]
          }
          frame 1 {
            # "empty row"
          }
          frame Default {
          }
        }
      }
      frame "--- Source Pin Modify Operations ---" {
      }
      frame "Update Pin Name" {
        # "Modify Source Pin mapping of selected pin in 'Source Pin Seq'"
        n590 = Unbundle By Name(w1650) -> ("Legend.Current (A)"=w1630:T13[], "Legend.Voltage (V)"=w1632:T13[], "Indices.Actual Sel Row"=w1629:i32, "Pin Config.Source Pin Config"=w1635:T5[], "List Specs.Pin List"=w1641:string[], "List Specs.UI Pin List"=w1649:string[], "Indices.Selected Row"=w1639:i32, "Pinmap List"=w1638:string[], "Indices.Pin Change"=w1637:i32)
        n591 = Index Array(array=w1638, index=w1637) -> (element=w1628:string)
        n592 = in-place "In Place Element Structure" {
          in-place-border: w1628 -> [w1656]
          in-place-border: w1628 -> [w1652]
          n593 = in-place-array #3(w1630, w1629) -> (w1653:T13)
          n594 = in-place-array #4(w1632, w1629) -> (w1655:T13)
          n595 = Bundle By Name(cluster=w1653, "Name"=w1652) -> (w1651:T13)
          n596 = Bundle By Name(cluster=w1655, "Name"=w1656) -> (w1654:T13)
          n597 = in-place-array #3(w1651) -> (w1627:T13[])  [unwired: 1 out]
          n598 = in-place-array #4(w1654) -> (w1631:T13[])  [unwired: 1 out]
        }
        n599 = Format Into String(format string="\n      %s\n", initial string="", error in=w1644, w1628) -> (resulting string=w1642:string, error out=w1643:errorcluster)
        n600 = in-place "In Place Element Structure" {
          in-place-border: w1628 -> [w1659]
          in-place-border: [w1657] -> w1636
          n601 = in-place-array #5(w1635, w1629) -> (w1658:T5)
          n602 = Bundle By Name(cluster=w1658, "Pin"=w1659) -> (w1657:T5)
          n603 = in-place-array #5(w1657) -> (w1634:T5[])  [unwired: 1 out]
        }
        n604 = Replace Array Subset(array=w1641, new element=w1628, index=w1629) -> (w1640:string[])
        n605 = Replace Array Subset(array=w1649, new element=w1642, index=w1639) -> (w1647:string[])
        n606 = Bundle By Name(cluster=w1650, "Legend.Current (A)"=w1627, "Legend.Voltage (V)"=w1631, "Pin Config.Source Pin Config"=w1634, "Pin Config.Active Pin Config"=w1636, "List Specs.Pin List"=w1640, "List Specs.UI Pin List"=w1647, "Flags.Check All?"=TRUE) -> (w1648:T14)
      }
      frame "--- Source Pin Delete Operations ---" {
      }
      frame "Check Delete Pin?" {
        # "Check for valid Delete operation"
        n607 = Unbundle By Name(w1671) -> ("#Rows"=w1670:u32, "Indices.Selected Row"=w1667:i32)
        n608 = Greater Or Equal To 0?(x=w1667) -> (x >= 0?=w1666:bool)
        n609 = Greater Than 0?(x=w1670) -> (x > 0?=w1669:bool)
        n610 = Compound Arithmetic op=AND(w1669, w1666) -> (w1668:bool)
        n611 = case shown="True" w1668 {
          tunnel: [string[] ["Delete Pin", "Load Adjacent Pin Config", "Re-Calculate Top Row", "Hide Hover Icon", "Hide Reorder Hover Icon", "Hide Selection Icon", "Check Pin List Scrollbar", "Update UI", "Update Plot Legend", "Update Icon State", "Update Power Down"] string[] ["Update Icon State", "Update Power Down"]] -> w1663
          frame True {
            # "non-empty seq and non-zero selected row"
          }
          frame False {
          }
        }
        n612 = for {
          tunnel: w1664 -> [w1674]
          tunnel: w1663 -> [w1673] mode=indexing
          shift-right: [w1675] -> w1665
          shift-left: w1662 -> [w1676]
          n613 = Enqueue Element(queue=w1674, element=w1673, timeout in ms (-1)=50, error in (no error)=w1676) -> (error out=w1675:errorcluster)  [unwired: 2 out]
        }
      }
      frame "Delete Pin" {
        # "when user deletes thef first pin in the sequence, ensure the new first pin's Relative To value is set to\n'Power sequence start'\nNote - Auto do it since delete operation cannot be restored"
        # "Delete  source pin configuration from the 'Source Pin Seq'"
        n614 = Unbundle By Name(w1711) -> ("#Rows"=w1702:u32, "List Specs.Pin List"=w1705:string[], "List Specs.UI Pin List"=w1710:string[], "Indices.Selected Row"=w1704:i32, "Indices.Actual Sel Row"=w1684:i32, "Pin Config.Source Pin Config"=w1700:T5[], "Pin Config.Color Array"=w1698:T3, "Pin Config.Error Info"=w1694:string[], "Pin Config.Error Ind"=w1691:i32[], "Legend.Voltage (V)"=w1689:T13[], "Legend.Current (A)"=w1683:T13[], "Ref Colors"=w1680:u32[], "Plot Colors"=w1685:u32[])
        n615 = expression code="x-2"(w1702) -> (w1699:u32)
        n616 = Delete From Array(array=w1689, index=w1684) -> (array with subset deleted=w1688:T13[])  [unwired: 1 in, 1 out]
        n617 = Delete From Array(array=w1683, index=w1684) -> (array with subset deleted=w1687:T13[])  [unwired: 1 in, 1 out]
        n618 = Delete From Array(array=w1700, index=w1684) -> (array with subset deleted=w1696:T5[])  [unwired: 1 in, 1 out]
        n619 = Delete From Array(array=w1691, index=w1684) -> (array with subset deleted=w1690:i32[])  [unwired: 1 in, 1 out]
        n620 = Delete From Array(array=w1698, index=w1684) -> (array with subset deleted=w1697:T3)  [unwired: 1 in, 1 out]
        n621 = Delete From Array(array=w1694, index=w1684) -> (array with subset deleted=w1693:string[])  [unwired: 1 in, 1 out]
        n622 = Delete From Array(array=w1705, index=w1684) -> (array with subset deleted=w1703:string[])  [unwired: 1 in, 1 out]
        n623 = Delete From Array(array=w1685, index=w1684) -> (deleted portion=w1681:u32, array with subset deleted=w1686:u32[])  [unwired: 1 in]
        n624 = case shown="Default" w1684 {
          tunnel: w1696 -> [w1720 w1721 w1725]
          tunnel: [w1720 w1721 w1722] -> w1695
          frame 1 {
            # "non-first row deleted"
          }
          frame Default {
          }
          frame 0 {
            # "first row is deleted"
            n625 = Index Array(array=w1725, index=0) -> (element=w1727:T5)
            n626 = Bundle By Name(cluster=w1727, "RELATIVE TO"=UI_Relative_To."Power sequence start") -> (w1723:T5)
            n627 = Replace Array Subset(array=w1725, new element=w1723, index=0) -> (w1722:T5[])
          }
        }
        n628 = Delete From Array(array=w1710, length=2, index=w1704) -> (array with subset deleted=w1708:string[])  [unwired: 1 out]
        n629 = Search 1D Array(1D array=w1680, element=w1681) -> (index of element=w1679:i32)  [unwired: 1 in]
        n630 = expression code="x/2"(w1699) -> (w1701:u32)
        n631 = case shown="-1, Default" w1679 {
          tunnel: w1686 -> [w1715 w1716 w1719]
          tunnel: [w1712 w1716 w1718] -> w1682
          tunnel: w1681 -> [w1714 _ w1717]
          frame 67 {
            n632 = Insert Into Array(array=w1715, index=15, new element=w1714) -> (w1712:u32[])
          }
          frame -1, Default {
          }
          frame 0..30 {
            n633 = Build Array (concatenate)(w1719, w1717) -> (w1718:u32[])
          }
        }
        n634 = Bundle By Name(cluster=w1711, "Flags.Check All?"=TRUE, "Indices.Row No Ref"=w1701, "#Rows"=w1699, "List Specs.Pin List"=w1703, "List Specs.UI Pin List"=w1708, "Pin Config.Source Pin Config"=w1695, "Pin Config.Color Array"=w1697, "Pin Config.Error Info"=w1693, "Pin Config.Error Ind"=w1690, "Legend.Voltage (V)"=w1688, "Legend.Current (A)"=w1687, "Plot Colors"=w1682) -> (w1709:T14)
      }
      frame "Load Adjacent Pin Config" {
        w1734 = -1 ("t")
        # "True - load pin config below the deleted pin \nFalse - deleted pin was the last in seq, hence move up"
        # "Load configuration of adjacent pin after delete operation"
        n635 = Unbundle By Name(w1747) -> ("Indices.Selected Row"=w1740:i32, "#Rows"=w1744:u32)
        n636 = To Long Integer(number=w1744) -> (32bit integer=w1729:i32)
        n637 = Not Equal?(x=w1740, y=w1729) -> (x != y?=w1730:bool)
        n638 = expression code="x-2"(w1729) -> (w1743:i32)
        n639 = Select(t=w1740, s=w1730, f=w1743) -> (s? t:f=w1733:i32)
        n640 = Less Than 0?(x=w1733) -> (x < 0?=w1735:bool)
        n641 = expression code="x/2"(w1733) -> (w1732:i32)
        n642 = Select(t=w1734, s=w1735, f=w1732) -> (s? t:f=w1731:i32)
        n643 = Select(t=string[] ["Check Limits", "Update Active Pin Config", "Update Meas Config", "Validate Inputs", "Update Error Info", "Update Error Display Top Row", "Update Error Display Scrollbar"], s=w1735, f=string[] ["Get Mouse Down Row Info"]) -> (s? t:f=w1738:string[])
        n644 = Select(t=w1734, s=w1735, f=w1733) -> (s? t:f=w1739:i32)
        n645 = for {
          tunnel: w1741 -> [w1750]
          tunnel: w1738 -> [w1748] mode=indexing
          shift-right: [w1751] -> w1742
          shift-left: w1745 -> [w1752]
          n646 = Enqueue Element(queue=w1750, element=w1748, timeout in ms (-1)=50, error in (no error)=w1752) -> (error out=w1751:errorcluster)  [unwired: 2 out]
        }
        n647 = Bundle By Name(cluster=w1747, "Indices.Actual Sel Row"=w1731, "Indices.Selected Row"=w1739) -> (w1746:T14)
      }
      frame "Re-Calculate Top Row" {
        # "True - two scenarios\n      True -  selected row is hidden above the top row, so move top row a level higher\n       False - the selected row is already is in visible range - so no changes\nFalse - selected row is hidden beneath the last visible row in seq, hence move top row such that \nselected row is the last visible row"
        # "Re-evaluate the top row after every delete action to ensure new selected row is in visible range"
        n648 = Unbundle By Name(w1770) -> ("#Rows"=w1753:u32, "Indices.Top Row"=w1766:u32, "Indices.Selected Row"=w1765:i32)
        n649 = To Long Integer(number=w1766) -> (32bit integer=w1764:i32)
        n650 = To Long Integer(number=w1753) -> (32bit integer=w1763:i32)
        n651 = Add(x=w1764, y=16) -> (x+y=w1757:i32)
        n652 = expression code="x>0?x-2:0"(w1764) -> (w1754:i32)
        n653 = Greater?(x=w1757, y=w1765) -> (0:w1760:bool)
        n654 = Greater Or Equal?(x=w1757, y=w1763) -> (x >= y?=w1756:bool)
        n655 = Subtract(x=w1765, y=16) -> (x-y=w1758:i32)
        n656 = Select(t=w1754, s=w1756, f=w1764) -> (s? t:f=w1755:i32)
        n657 = Select(t=w1755, s=w1760, f=w1758) -> (s? t:f=w1767:i32)
        n658 = To Unsigned Long Integer(number=w1767) -> (unsigned 32bit integer=w1762:u32)
        n659 = Bundle By Name(cluster=w1770, "Indices.Top Row"=w1762) -> (w1769:T14)
      }
      frame "Source Pin Add Operations ---" {
      }
      frame "Add Pin" {
        w1798 = u32 18 ("y")
        # "Pick white as default color\nfor any pin >31"
        # "Add a new entry to Source Pin Seq'"
        n660 = Unbundle By Name(w1807) -> ("Pin Config.Power Up/Down"=w1785:bool, "Indices.Top Row"=w1792:u32, "#Rows"=w1797:u32, "Pin Config.Source Pin Config"=w1806:T5[], "Pin Config.Color Array"=w1800:T3, "Legend.Voltage (V)"=w1790:T13[], "Legend.Current (A)"=w1789:T13[], "Plot Colors"=w1781:u32[], "Indices.Row No Ref"=w1780:u32)
        n661 = To Long Integer(number=w1780) -> (32bit integer=w1778:i32)
        n662 = Less Or Equal?(x=w1778, y=30) -> (x <= y?=w1776:bool)
        n663 = Index Array(array=w1781, index=w1778) -> (element=w1775:u32)
        n664 = Select(t=w1775, s=w1776, f=u32 16777215) -> (s? t:f=w1774:u32)
        n665 = Bundle By Name(cluster=T13 {"Color"=0, "Name"="Pin", "Visible"=TRUE} ("Plot"), "Color"=w1774) -> (w1788:T13)
        n666 = Select(t=T5 {"Pin"="", "MODE"="", "TARGET VALUE"=0.0, "RAMP RATE"=0.003, "COMPLIANCE LIMIT"=0.01, "START DELAY"=0.0, "Source Mode"=0, "RELATIVE TO"=enum."Power sequence start", "DEFAULT RAMP RATE"=TRUE, "SENSE MODE"=0, "Sense Mode Frame"="", "TRANSIENT RESPONSE"=2, "Transient Reponse Frame"="", "START VALUE"=1.8} ("Pin Config"), s=w1785, f=T5 {"Pin"="", "MODE"="", "TARGET VALUE"=1.8, "RAMP RATE"=0.003, "COMPLIANCE LIMIT"=0.01, "START DELAY"=0.0, "Source Mode"=0, "RELATIVE TO"=enum."Power sequence start", "DEFAULT RAMP RATE"=TRUE, "SENSE MODE"=0, "Sense Mode Frame"="", "TRANSIENT RESPONSE"=2, "Transient Reponse Frame"="", "START VALUE"=0.0} ("Pin Config")) -> (s? t:f=w1782:T5)
        n667 = expression code="x+2"(w1797) -> (w1796:u32)
        n668 = Quotient & Remainder(x=w1797, y=u32 2) -> (floor(x/y)=w1803:u32)  [unwired: 1 out]
        n669 = Initialize Array("" ("Empty String Constant"), 1 ("dimension size")) -> (w1810:string[])
        n670 = Insert Into Array(array=w1806, new element=w1782) -> (w1805:T5[])  [unwired: 1 in]
        n671 = Insert Into Array(array=w1800, new element=w1774) -> (w1779:T3)  [unwired: 1 in]
        n672 = Greater?(x=w1796, y=w1798) -> (0:w1795:bool)
        n673 = Subtract(x=w1796, y=w1798) -> (x-y=w1793:u32)
        n674 = To Long Integer(number=w1797) -> (32bit integer=w1801:i32)
        n675 = To Long Integer(number=w1803) -> (32bit integer=w1802:i32)
        n676 = Select(t=w1793, s=w1795, f=w1792) -> (s? t:f=w1794:u32)
        n677 = Insert Into Array(array=w1790, new element=w1788) -> (w1787:T13[])  [unwired: 1 in]
        n678 = Insert Into Array(array=w1789, new element=w1788) -> (w1786:T13[])  [unwired: 1 in]
        n679 = Bundle By Name(cluster=w1807, "Indices.Top Row"=w1794, "Flags.Check All?"=FALSE, "Indices.Actual Sel Row"=w1802, "Indices.Selected Row"=w1801, "Pins"=w1810, "Pin Config.Source Pin Config"=w1805, "Pin Config.Active Pin Config"=w1782, "Pin Config.Color Array"=w1779, "Legend.Voltage (V)"=w1787, "Legend.Current (A)"=w1786) -> (w1811:T14)
      }
      frame "--- Source Pin Sequence Scroll Operations ---" {
      }
      frame "Set Source Pin Seq Top Row" {
        # "#coercion dot"
        # "needed since each pin in seq is of two rows -\none actual and one empty row"
        # "true --- scrollbar moved down\nif selected row is lesser than top row - hide selection icon\nelse re-posiition selection icon\nfalse --- scrollbar moved up\nif selected row is greater than 18 rows ( the no of rows at max visible) away from toprow - hide selection icon\nelse re-position selection icon"
        # "Determine 'Source Pin Seq' Top Row visible based on scrollbar value"
        n680 = Unbundle By Name(w1834) -> ("Scrollbar.New Val"=w1828:i32, "Scrollbar.Old Val"=w1827:i32, "Indices.Selected Row"=w1815:i32)
        n681 = Greater?(x=w1828, y=w1827) -> (0:w1824:bool)
        n682 = expression code="x-2"(w1815) -> (w1826:i32)
        n683 = expression code="x+2"(w1815) -> (w1825:i32)
        n684 = Multiply(x=2 ("y"), y=w1828) -> (x*y=w1818:i32)
        n685 = To Unsigned Long Integer(number=w1818) -> (unsigned 32bit integer=w1816:u32)
        n686 = Select(t=w1826, s=w1824, f=w1825) -> (s? t:f=w1817:i32)
        n687 = property on="Source Pin Seq" class="LstBox (strict)"(error in=w1831, "Top Row"=w1816, "Active Row"=w1815) -> (error out=w1823:errorcluster, "ActiveRowPosLeft"=w1830:i32, "ActiveRowPosTop"=w1829:i32)  [unwired: 1 in, 1 out]
        n688 = Bundle By Name(cluster=w1834, "Indices.Top Row"=w1816, "Coords.Active Row Pos.Left"=w1830, "Coords.Active Row Pos.Top"=w1829) -> (w1833:T14)
        n689 = case shown="False" w1824 {
          tunnel: w1817 -> [w1839 _]
          tunnel: [w1835 w1844] -> w1822
          tunnel: w1815 -> [_ w1842]
          tunnel: w1818 -> [_ w1841]
          frame True {
            # "scrollbar moved down"
            n690 = Greater Or Equal To 0?(x=w1839) -> (x >= 0?=w1838:bool)
            n691 = Select(t="Overlap White Dropdown", s=w1838, f="Hide Selection Icon") -> (s? t:f=w1835:string)
          }
          frame False {
            # "scrollbar moved up"
            n692 = Subtract(x=w1842, y=w1841) -> (x-y=w1840:i32)
            n693 = Greater?(x=w1840, y=18) -> (0:w1847:bool)
            n694 = Select(t="Hide Selection Icon", s=w1847, f="Overlap White Dropdown") -> (s? t:f=w1844:string)
          }
        }
        n695 = Enqueue Element(queue=w1820, element=w1822, timeout in ms (-1)=50, error in (no error)=w1823) -> (error out=w1819:errorcluster)  [unwired: 2 out]
      }
      frame "Check Pin List Scrollbar" {
        w1855 = u32 18 ("y")
        # "Determine is scrollbar is needed and its range"
        n696 = Unbundle By Name(w1857) -> ("#Rows"=w1853:u32)
        n697 = Greater?(x=w1853, y=w1855) -> (0:w1850:bool)
        n698 = Subtract(x=w1853, y=w1855) -> (x-y=w1848:u32)
        n699 = Select(t=u32 18 ("y"), s=w1850, f=w1853) -> (s? t:f=w1851:u32)
        n700 = expression code="x/2+1"(w1848) -> (w1849:u32)
        n701 = Bundle By Name(cluster=w1857, "Flags.Visibilty.Scrollbar?"=w1850, "Indices.NumRows"=w1851, "Scrollbar.DocMax"=w1849) -> (w1852:T14)
      }
      frame "--- Source Pin Sequence Reorder Operations ---" {
      }
      frame "Check for valid pin re-order" {
        # "valid when - \ndrag and drop indices are not the same\nmouse did not leave 'Source Pin Seq' control"
        # "Check if the reordering is valid or not"
        n702 = Unbundle By Name(w1874) -> ("Seq Reorder.Drag Ind"=w1868:i32, "Seq Reorder.Drop Ind"=w1861:i32, "Seq Reorder.Drag?"=w1864:bool)
        n703 = expression code="x%2 ? x-1 : x"(w1861) -> (w1860:i32)
        n704 = Greater?(x=w1868, y=w1860) -> (0:w1867:bool)
        n705 = Not Equal?(x=w1868, y=w1860) -> (x != y?=w1873:bool)
        n706 = Compound Arithmetic op=AND(w1873, w1864) -> (w1865:bool)
        n707 = case shown="True" w1865 {
          tunnel: w1872 -> [w1875 w1879]
          tunnel: [w1875 w1878] -> w1871
          tunnel: w1870 -> [_ w1877]
          tunnel: string[] ["Restore Cell Font Color", "Update Power Down", "Reorder Pins", "Re-Calculate Parameters", "Update UI", "Update Plot Legend", "Get Mouse Down Row Info"] -> [_ w1876]
          frame False {
          }
          frame True {
            # "valid reordering"
            n708 = for {
              tunnel: w1877 -> [w1882]
              tunnel: w1876 -> [w1880] mode=indexing
              shift-right: [w1883] -> w1878
              shift-left: w1879 -> [w1884]
              n709 = Enqueue Element(queue=w1882, element=w1880, timeout in ms (-1)=50, error in (no error)=w1884) -> (error out=w1883:errorcluster)  [unwired: 2 out]
            }
          }
        }
        n710 = Select(t=w1864, s=w1865, f=FALSE) -> (s? t:f=w1862:bool)
        n711 = Bundle By Name(cluster=w1874, "Seq Reorder.Up?"=w1867, "Seq Reorder.Drag?"=w1862) -> (w1866:T14)
      }
      frame "Move Pin" {
        # "Determine the start and stop index for rerdering the seleced pin"
        n712 = Unbundle By Name(w1895) -> ("Indices.Selected Row"=w1893:i32, "Seq Reorder.Up?"=w1891:bool, "#Rows"=w1890:u32)
        n713 = case shown="False" w1891 {
          tunnel: w1893 -> [w1903 w1908]
          tunnel: [w1901 w1907] -> w1885
          tunnel: [w1902 w1906] -> w1892
          tunnel: w1890 -> [_ w1905]
          frame True {
            # "Move up - valid only if drop index is not less than 0"
            n714 = expression code="x-2"(w1903) -> (w1901:i32)
            n715 = Greater Or Equal To 0?(x=w1901) -> (x >= 0?=w1902:bool)
          }
          frame False {
            # "Move down - valid only if drop index is not greater than seq size"
            n716 = expression code="x+2"(w1908) -> (w1907:i32)
            n717 = To Long Integer(number=w1905) -> (32bit integer=w1904:i32)
            n718 = Less?(x=w1907, y=w1904) -> (x < y?=w1906:bool)
          }
        }
        n719 = case shown="True" w1892 {
          tunnel: [string[] ["Update Icon State"] string[] ["Restore Cell Font Color", "Reorder Pins", "Re-Calculate Parameters", "Update UI", "Update Plot Legend", "Get Mouse Down Row Info", "Update Icon State", "Update Power Down"]] -> w1887
          frame False {
            # "invalid reorder"
          }
          frame True {
            # "valid reorder"
          }
        }
        n720 = Bundle By Name(cluster=w1895, "Seq Reorder.Drag Ind"=w1893, "Seq Reorder.Drop Ind"=w1885) -> (w1894:T14)
        n721 = for {
          tunnel: w1886 -> [w1898]
          tunnel: w1887 -> [w1896] mode=indexing
          shift-right: [w1899] -> w1888
          shift-left: w1889 -> [w1900]
          n722 = Enqueue Element(queue=w1898, element=w1896, timeout in ms (-1)=50, error in (no error)=w1900) -> (error out=w1899:errorcluster)  [unwired: 2 out]
        }
      }
      frame "Reorder Pins" {
        # "round off drop index to ensure it doesnt happen in empty rows"
        # "Reorder all necessary configurations in pin sequence"
        n723 = Unbundle By Name(w1956) -> ("List Specs.UI Pin List"=w1953:string[], "Seq Reorder.Drag Ind"=w1945:i32, "Seq Reorder.Drop Ind"=w1917:i32, "List Specs.Pin List"=w1948:string[], "Pin Config.Source Pin Config"=w1943:T5[], "Pin Config.Error Info"=w1938:string[], "Pin Config.Color Array"=w1934:T3, "Pin Config.Error Ind"=w1929:i32[], "Legend.Voltage (V)"=w1925:T13[], "Legend.Current (A)"=w1921:T13[], "Plot Colors"=w1915:u32[])
        n724 = expression code="x%2 ? x-1 : x"(w1917) -> (w1918:i32)
        n725 = expression code="x/2"(w1918) -> (w1912:i32)
        n726 = expression code="x/2"(w1945) -> (w1914:i32)
        n727 = Delete From Array(array=w1953, length=2, index=w1945) -> (deleted portion=w1951:string[], array with subset deleted=w1952:string[])
        n728 = Delete From Array(array=w1934, index=w1914) -> (deleted portion=w1932:u32, array with subset deleted=w1933:T3)  [unwired: 1 in]
        n729 = Delete From Array(array=w1925, index=w1914) -> (deleted portion=w1926:T13, array with subset deleted=w1924:T13[])  [unwired: 1 in]
        n730 = Delete From Array(array=w1921, index=w1914) -> (deleted portion=w1922:T13, array with subset deleted=w1920:T13[])  [unwired: 1 in]
        n731 = Delete From Array(array=w1948, index=w1914) -> (deleted portion=w1946:string, array with subset deleted=w1949:string[])  [unwired: 1 in]
        n732 = Delete From Array(array=w1938, index=w1914) -> (deleted portion=w1939:string, array with subset deleted=w1937:string[])  [unwired: 1 in]
        n733 = Delete From Array(array=w1929, index=w1914) -> (deleted portion=w1930:i32, array with subset deleted=w1928:i32[])  [unwired: 1 in]
        n734 = Delete From Array(array=w1943, index=w1914) -> (deleted portion=w1942:T5, array with subset deleted=w1941:T5[])  [unwired: 1 in]
        n735 = Delete From Array(array=w1915, index=w1914) -> (deleted portion=w1913:u32, array with subset deleted=w1916:u32[])  [unwired: 1 in]
        n736 = Insert Into Array(array=w1952, index=w1918, new element=w1951) -> (w1950:string[])
        n737 = Insert Into Array(array=w1949, index=w1912, new element=w1946) -> (w1947:string[])
        n738 = Insert Into Array(array=w1933, index=w1912, new element=w1932) -> (w1931:T3)
        n739 = Insert Into Array(array=w1924, index=w1912, new element=w1926) -> (w1923:T13[])
        n740 = Insert Into Array(array=w1920, index=w1912, new element=w1922) -> (w1919:T13[])
        n741 = Insert Into Array(array=w1937, index=w1912, new element=w1939) -> (w1936:string[])
        n742 = Insert Into Array(array=w1941, index=w1912, new element=w1942) -> (w1940:T5[])
        n743 = Insert Into Array(array=w1928, index=w1912, new element=w1930) -> (w1927:i32[])
        n744 = Insert Into Array(array=w1916, index=w1912, new element=w1913) -> (w1911:u32[])
        n745 = Bundle By Name(cluster=w1956, "Seq Reorder.Drag?"=FALSE, "List Specs.UI Pin List"=w1950, "Seq Reorder.Drop Ind"=w1918, "List Specs.Pin List"=w1947, "Pin Config.Source Pin Config"=w1940, "Pin Config.Error Info"=w1936, "Flags.Check All?"=TRUE, "Pin Config.Color Array"=w1931, "Pin Config.Error Ind"=w1927, "Legend.Voltage (V)"=w1923, "Legend.Current (A)"=w1919, "Plot Colors"=w1911) -> (w1955:T14)
      }
      frame "Re-Calculate Parameters" {
        # "Top Row ::\nif top row is greater than selected row after moving up, it means selected row will be hidden\nin such a case, make the selected row the top row, else pass the top row as it is\n\nSelected Row ::\nSubtract existing selected row by the number of rows being moved up"
        # "Top Row ::\nif the gap b/w selected row and top row is greater than 18 (max rows visible at any time)  after moving down, it means selected row will be hidden.\nIn such a case, subtract the selected row from 16  to get the top row, else pass the top row as it is\n\nSelected Row ::\nAdd existing selected row by the number of rows being moved down"
        # "Calculate top row post re-ordering to ensure the selected row after re-ordering is still visible to the user"
        n746 = Unbundle By Name(w1974) -> ("Indices.Top Row"=w1963:u32, "Seq Reorder.Drag Ind"=w1971:i32, "Seq Reorder.Drop Ind"=w1970:i32, "Indices.Selected Row"=w1964:i32, "Seq Reorder.Up?"=w1966:bool, "Indices.Selected Row"=w1968:i32)
        n747 = Subtract(x=w1971, y=w1970) -> (x-y=w1969:i32)
        n748 = Absolute Value(x=w1969) -> (abs(x)=w1967:i32)
        n749 = To Long Integer(number=w1963) -> (32bit integer=w1962:i32)
        n750 = case shown="True" w1966 {
          tunnel: w1968 -> [_ w1992]
          tunnel: w1967 -> [w1981 w1991]
          tunnel: [w1978 w1988] -> w1965
          tunnel: w1964 -> [w1979 _]
          tunnel: w1962 -> [w1977 w1987]
          tunnel: [w1976 w1985] -> w1960
          frame True {
            # "move up"
            n751 = Subtract(x=w1979, y=w1981) -> (x-y=w1982:i32)
            n752 = Greater?(x=w1977, y=w1982) -> (0:w1980:bool)
            n753 = Select(t=w1982, s=w1980, f=w1977) -> (s? t:f=w1978:i32)
            n754 = expression code="x<0?0:x"(w1982) -> (w1976:i32)
          }
          frame False {
            # "move down"
            n755 = Add(x=w1991, y=w1992) -> (x+y=w1985:i32)
            n756 = Subtract(x=w1985, y=w1987) -> (x-y=w1986:i32)
            n757 = Greater Or Equal?(x=w1986, y=18) -> (x >= y?=w1989:bool)
            n758 = Subtract(x=w1985, y=16) -> (x-y=w1983:i32)
            n759 = Select(t=w1983, s=w1989, f=w1987) -> (s? t:f=w1988:i32)
          }
        }
        n760 = To Unsigned Long Integer(number=w1965) -> (unsigned 32bit integer=w1961:u32)
        n761 = Quotient & Remainder(x=w1960, y=2) -> (floor(x/y)=w1959:i32)  [unwired: 1 out]
        n762 = Bundle By Name(cluster=w1974, "Indices.Top Row"=w1961, "Indices.Actual Sel Row"=w1959, "Indices.Selected Row"=w1960, "Seq Reorder.Drag?"=FALSE) -> (w1973:T14)
      }
      frame "--- UI Update Operations ---" {
      }
      frame "Hide Listbox" {
        # "Hide 'Source Pin Selection' listbox control"
        n763 = Bundle By Name(cluster=w2001, "Flags.Visibilty.Pin Selection List"=FALSE ("Visibilty.Pin Selection List")) -> (w1996:T14)
        n764 = property on="Pin Selection" class="LstBox (strict)"(error in=w2000, "Left"=1713, "Top"=652) -> (error out=w1999:errorcluster)  [unwired: 1 in, 1 out]
      }
      frame "Hide Reorder Hover Icon" {
        # "Hide 'Reorder Hover Icon' control"
        n765 = Bundle By Name(cluster=w2008, "Flags.Visibilty.Reorder Hover Icon"=FALSE ("Visibilty.Pin Selection List")) -> (w2003:T14)
        n766 = property on="Reorder Hover Icon" class="Bool (strict)"(error in=w2007, "Left"=1713, "Top"=652) -> (error out=w2006:errorcluster)  [unwired: 1 in, 1 out]
      }
      frame "Hide Hover Icon" {
        # "Hide 'Hover icon'  control"
        n767 = Bundle By Name(cluster=w2016, "Flags.Visibilty.Hover Icon"=FALSE ("Visibilty.Hover Icon"), "Flags.Same Hover Row?"=FALSE) -> (w2011:T14)
        n768 = property on="Hover icon" class="Bool (strict)"(error in=w2015, "Left"=1713, "Top"=652) -> (error out=w2014:errorcluster)  [unwired: 1 in, 1 out]
      }
      frame "Format Selection List" {
        # "#coercion dot"
        # "Format the 'Pin Selection' rows upon hover"
        n769 = Unbundle By Name(w2020) -> ("Pin Selection.Selection Coords"=w2019:cluster{"Horizontal":i32, "Vertical":i32})
        n770 = invoke on="Pin Selection" class="LstBox (strict)" method="Point To Row"(error in=w2021, "Point"=w2019) -> (error out=w2026:errorcluster, "Row"=w2025:i32)  [unwired: 5 in, 5 out]
        n771 = property on="Pin Selection" class="LstBox (strict)"(error in=w2026, "Active Row"=-2 ("Active Row:Active Row Number"), "CellFontColor"=u32 0 ("Active Row:Cell Font:Color"), "CellBG"=u32 16250871 ("Active Row:Cell Font:Color"), "Active Row"=w2025, "CellBG"=u32 11783650 ("Color")) -> (error out=w2018:errorcluster)  [unwired: 1 in, 1 out]
      }
      frame "Hide Selection Icon" {
        # "Hide 'Selection icon' control"
        n772 = property on="Selection icon" class="Bool (strict)"(error in=w2032, "Left"=1713, "Top"=652) -> (error out=w2031:errorcluster)  [unwired: 1 in, 1 out]
        n773 = Bundle By Name(cluster=w2033, "Flags.Visibilty.Selection Icon"=FALSE ("Visibilty.Selection Icon")) -> (w2028:T14)
      }
      frame "Hide Border" {
        # "Hide 'Border' indicator"
        n774 = property on="Border" class="Str"(error in=w2040, "Left"=1027, "Top"=300, "Visible"=FALSE) -> (error out=w2039:errorcluster)  [unwired: 1 in, 1 out]
        n775 = Bundle By Name(cluster=w2041, "Flags.Visibilty.Border"=FALSE ("Visibilty.Border")) -> (w2035:T14)
      }
      frame "Hide Image" {
        # "Toggle the visibility of Info image"
        n776 = Unbundle By Name(w2044) -> ("Flags.Visibilty.Help?"=w2045:bool)
        n777 = Not(x=w2045) -> (.not. x?=w2043:bool)
        n778 = property on="R-Image" class="Bool (strict)"(error in=w2047, "Visible"=w2043) -> (error out=w2046:errorcluster)  [unwired: 1 in, 1 out]
        n779 = Bundle By Name(cluster=w2044, "Flags.Visibilty.Help?"=w2043) -> (w2042:T14)
      }
      frame "Hide Power Down Image" {
        # "Toggle the visibility of Power Down image"
        n780 = Unbundle By Name(w2051) -> ("Flags.Visibilty.PD Info"=w2052:bool)
        n781 = Not(x=w2052) -> (.not. x?=w2048:bool)
        n782 = property on="PD-Image" class="Bool (strict)"(error in=w2053, "Visible"=w2048) -> (error out=w2049:errorcluster)  [unwired: 1 in, 1 out]
        n783 = Bundle By Name(cluster=w2051, "Flags.Visibilty.PD Info"=w2048) -> (w2050:T14)
      }
      frame "Show/Hide Legend" {
        # "Show/Hide plot Legend  control"
        n784 = Unbundle By Name(w2068) -> ("#Rows"=w2057:u32, "Coords.Monitor.Right"=w2063:i32, "Coords.Plot Legend.Width"=w2061:i32, "#Rows"=w2060:u32, "Coords.Empty Legend.Width"=w2059:i32, "Flags.Visibilty.Plot Legend"=w2067:bool)
        n785 = Greater Than 0?(x=w2060) -> (x > 0?=w2055:bool)
        n786 = Select(t=w2061, s=w2055, f=w2059) -> (s? t:f=w2058:i32)
        n787 = Subtract(x=w2063, y=w2058) -> (x-y=w2054:i32)
        n788 = property on="Monitor" class="Bool (strict)"(error in=w2069, "Value"=w2067) -> (error out=w2065:errorcluster)  [unwired: 1 in, 1 out]
        n789 = case shown="False" w2067 {
          tunnel: [736 ("Left") w2093] -> w2062
          tunnel: [505 ("Top") -2 ("Top")] -> w2066
          tunnel: w2054 -> [_ w2093]
          frame False {
            # "hide plot legend"
          }
          frame True {
            # "show plot legend"
          }
        }
        n790 = case shown="2.., Default" w2057 {
          tunnel: w2066 -> [w2076 w2090]
          tunnel: w2065 -> [w2079 w2089]
          tunnel: [w2081 w2088] -> w2064
          tunnel: w2062 -> [w2077 w2087]
          frame 0 {
            # "First call will be to hide, so ensure both legends\nare hidden (only a dev env scenario)"
            # "empty pin sequence - show/hide empty plot legend control"
            n791 = property on="Empty Legend" class="Clust (strict)"(error in=w2079, "Left"=w2077, "Top"=w2076) -> (error out=w2078:errorcluster)  [unwired: 1 in, 1 out]
            n792 = First Call?() -> (First Call?: T/F=w2080:bool)
            n793 = case shown="True" w2080 {
              tunnel: w2078 -> [w2082 w2086]
              tunnel: [w2082 w2085] -> w2081
              tunnel: w2077 -> [_ w2084]
              tunnel: w2076 -> [_ w2083]
              frame False {
              }
              frame True {
                n794 = property on="Legend" class="Clust (strict)"(error in=w2086, "Left"=w2084, "Top"=w2083) -> (error out=w2085:errorcluster)  [unwired: 1 in, 1 out]
              }
            }
          }
          frame 2.., Default {
            # "non-empty pin sequence - show/hide plot egend"
            n795 = property on="Legend" class="Clust (strict)"(error in=w2089, "Left"=w2087, "Top"=w2090) -> (error out=w2088:errorcluster)  [unwired: 1 in, 1 out]
          }
        }
        n796 = case shown="False" w2055 {
          tunnel: w2068 -> [w2072 w2075]
          tunnel: [w2071 w2074] -> w2056
          tunnel: w2054 -> [w2070 w2073]
          frame False {
            # "empty pin seq -empty legend control"
            n797 = Bundle By Name(cluster=w2072, "Coords.Empty Legend.Left"=w2070) -> (w2071:T14)
          }
          frame True {
            # "non-empty seq - plot legend control"
            n798 = Bundle By Name(cluster=w2075, "Coords.Plot Legend.Left"=w2073) -> (w2074:T14)
          }
        }
      }
      frame "Format Pin List" {
        # "#coercion dot"
        # "Format all rows of 'Source Pin Seq' listbox control"
        n799 = Unbundle By Name(w2098) -> ("List Specs.Active Row Nos"=w2097:u32[], "List Specs.CellBG"=w2096:u32[], "List Specs.Cell Height"=w2095:i32[])
        n800 = for {
          shift-right: [w2104] -> w2099
          shift-left: w2100 -> [w2105]
          tunnel: w2097 -> [w2103] mode=indexing
          tunnel: w2096 -> [w2102] mode=indexing
          tunnel: w2095 -> [w2101] mode=indexing
          n801 = property on="Source Pin Seq" class="LstBox (strict)"(error in=w2105, "Active Row"=w2103, "CellBG"=w2102, "Cell Height"=w2101, "CellFontColor"=u32 0) -> (error out=w2104:errorcluster)  [unwired: 1 in, 1 out]
        }
      }
      frame "Update UI" {
        # "Update 'Source Pin Seq', 'Pin Color Array' and 'Scrollbar' properties"
        n802 = Unbundle By Name(w2137) -> ("List Specs.UI Pin List"=w2123:string[], "Indices.Top Row"=w2129:u32, "Indices.NumRows"=w2114:u32, "Pin Config.Color Array"=w2116:T3, "Indices.Top Row"=w2111:u32, "Flags.Visibilty.Scrollbar?"=w2131:bool, "Scrollbar.DocMax"=w2132:u32)
        n803 = Quotient & Remainder(x=w2129, y=u32 2) -> (floor(x/y)=w2127:u32)  [unwired: 1 out]
        n804 = To Double Precision Float(number=w2132) -> (double precision float=w2125:dbl)
        n805 = To Long Integer(number=w2127) -> (32bit integer=w2126:i32)
        n806 = property on="Scrollbar" class="Scroll (strict)"(error in=w2108, "Visible"=w2131, "DocMax"=w2125, "DocMin"=0.0 ("Doc Min"), "CoerceMax"=TRUE ("Coerce Maximum Value"), "CoerceMin"=TRUE ("Coerce Minimum Value"), "PageSize"=1.0 ("Page Size"), "Increment"=1.0, "Value"=w2126) -> (error out=w2118:errorcluster)  [unwired: 1 in, 1 out]
        n807 = expression code="x/2"(w2111) -> (w2109:u32)
        n808 = Greater Than 0?(x=w2114) -> (x > 0?=w2112:bool)
        n809 = Quotient & Remainder(x=w2114, y=u32 2) -> (floor(x/y)=w2113:u32)  [unwired: 1 out]
        n810 = Build Array(w2109) -> (w2110:u32[])
        n811 = property on="Color Array" class="Arr (strict)"(error in=w2118, "Visible"=w2112, "Number of Rows"=w2113, "Value"=w2116, "Index Values"=w2110) -> (error out=w2117:errorcluster)  [unwired: 1 in, 1 out]
        n812 = To Long Integer(number=w2129) -> (32bit integer=w2120:i32)
        n813 = property on="Source Pin Seq" class="LstBox (strict)"(error in=w2117, "Item Names"=w2123, "Top Row"=w2120, "Number of Rows"=w2114, "Scrollbar Visible"=FALSE ("Visible Items:Vertical Scrollbar Visible"), "Visible"=w2112) -> (error out=w2107:errorcluster, "Height"=w2121:u32)  [unwired: 1 in, 1 out]
        n814 = To Long Integer(number=w2121) -> (32bit integer=w2119:i32)
        n815 = Bundle By Name(cluster=w2137, "Coords.Source Pin Seq.Height"=w2119) -> (w2124:T14)
      }
      frame "Update Plot Legend" {
        w2147 = u32[] [0] ("Index Values")
        # "#coercion dot"
        # "Update 'Plot Legend' properties"
        n816 = Unbundle By Name(w2157) -> ("Indices.NumRows"=w2154:u32, "Legend"=w2138:T12)
        n817 = expression code="x/2"(w2154) -> (w2153:u32)
        n818 = expression code="x/2>4?4:x/2"(w2154) -> (w2144:u32)
        n819 = property on="Legend" class="Clust (strict)"(error in=w2148, "Value"=w2138) -> (error out=w2149:errorcluster)  [unwired: 1 in, 1 out]
        n820 = Greater?(x=w2153, y=u32 4) -> (0:w2143:bool)
        n821 = property on="Voltage (V)" class="Arr (strict)"(error in=w2149, "Number of Rows"=w2144, "VertScroll"=w2143, "HorizScroll"=FALSE ("Horizontal Scrollbar Visible"), "Index Values"=w2147) -> (error out=w2151:errorcluster)  [unwired: 1 in, 1 out]
        n822 = property on="Current (A)" class="Arr (strict)"(error in=w2151, "Number of Rows"=w2144, "VertScroll"=w2143, "HorizScroll"=FALSE ("Horizontal Scrollbar Visible"), "Index Values"=w2147) -> (error out=w2142:errorcluster)  [unwired: 1 in, 1 out]
        n823 = property on="Legend" class="Clust (strict)"(error in=w2142) -> (error out=w2141:errorcluster, "Height"=w2140:u32, "Width"=w2139:u32)  [unwired: 1 in, 1 out]
        n824 = To Long Integer(number=w2140) -> (32bit integer=w2146:i32)
        n825 = To Long Integer(number=w2139) -> (32bit integer=w2145:i32)
        n826 = Bundle By Name(cluster=w2157, "Flags.Visibilty.Plot Legend Scrollbar"=w2143, "Coords.Plot Legend.Height"=w2146, "Coords.Plot Legend.Width"=w2145) -> (w2156:T14)
      }
      frame "Update Scrollbar" {
        # "Update scrollbar properties"
        n827 = Unbundle By Name(w2161) -> ("Indices.Top Row"=w2159:u32)
        n828 = To Long Integer(number=w2159) -> (32bit integer=w2158:i32)
        n829 = Quotient & Remainder(x=w2158, y=2) -> (floor(x/y)=w2162:i32)  [unwired: 1 out]
        n830 = property on="Scrollbar" class="Scroll (strict)"(error in=w2165, "Value"=w2162) -> (error out=w2164:errorcluster)  [unwired: 1 in, 1 out]
        n831 = property on="Source Pin Seq" class="LstBox (strict)"(error in=w2164, "Top Row"=w2158) -> (error out=w2160:errorcluster)  [unwired: 1 in, 1 out]
      }
      frame "Update Error Info" {
        # "Generate tipstrip for Error icon on UI\nEnsure error (if exists) for selected pin in seq is the selected row in Error Display"
        # "Display error status on UI for the 'Pin Sequence' and 'Selected Pin'"
        n832 = Unbundle By Name(w2185) -> ("Pin Config.Source Pin Config"=w2183:T5[], "Pin Config.Error Info"=w2184:string[], "Pin Config.Source Pin Config"=w2180:T5[], "Indices.Actual Sel Row"=w2174:i32)
        n833 = Index Array(array=w2180, index=w2174) -> (element=w2179:T5)
        n834 = Unbundle By Name(w2179) -> ("Pin"=w2178:string)
        n835 = for {
          tunnel: w2183 -> [w2209] mode=indexing
          tunnel: w2184 -> [w2187] mode=indexing
          tunnel: [w2190] -> w2172 mode=indexing if=w2189
          shift-right: [w2192] -> w2181
          shift-left: w2182 -> [w2207]
          tunnel: w2178 -> [w2199]
          tunnel: [w2196] -> w2177 mode=indexing if=w2189
          tunnel: w2174 -> [w2197]
          tunnel: [w2188] -> w2170 mode=indexing if=w2189
          i -> [w2188]
          # "err msg"
          # "source"
          # "for each pin in sequence"
          n836 = Unbundle By Name(w2209) -> ("Pin"=w2200:string)
          n837 = Equal?(x=w2188, y=w2197) -> (x = y?=w2195:bool)
          n838 = Equal?(x=w2200, y=w2199) -> (x = y?=w2198:bool)
          n839 = Empty String/Path?(string/path=w2200) -> (empty?=w2203:bool)
          n840 = Compound Arithmetic op=AND(w2198, w2195) -> (w2196:bool)
          n841 = Select(t="<empty>", s=w2203, f=w2200) -> (s? t:f=w2201:string)
          n842 = Empty String/Path?(string/path=w2187) -> (empty?=w2208:bool)
          n843 = Format Into String(format string="Pin - %s", initial string="", error in=w2207, w2201) -> (resulting string=w2204:string, error out=w2193:errorcluster)
          n844 = Not(x=w2208) -> (.not. x?=w2189:bool)
          n845 = Format Into String(format string="|   %s" ("initial string"), initial string="", error in=w2193, w2187) -> (resulting string=w2186:string, error out=w2192:errorcluster)
          n846 = Build Array(w2204, w2186) -> (w2190:string[])
        }
        n847 = Bundle By Name(cluster=w2185, "Pin Config.Error Ind"=w2170) -> (w2171:T14)
        n848 = Search 1D Array(1D array=w2177, element=TRUE) -> (index of element=w2173:i32)  [unwired: 1 in]
        n849 = Empty Array?(array=w2172) -> (empty?=w2167:bool)
        n850 = property on="Error Display" class="MCListbox (strict)"(error in=w2181, "ItemNames"=w2172, "Value"=w2173, "SelColor"=u32 11783650 ("Color")) -> (error out=w2169:errorcluster)  [unwired: 1 in, 1 out]
        n851 = Not(x=w2167) -> (.not. x?=w2166:bool)
        n852 = property on="Error" class="Bool (strict)"(error in=w2169, "Visible"=w2166) -> (error out=w2168:errorcluster)  [unwired: 1 in, 1 out]
      }
      frame "Update Error Display Top Row" {
        # "Ensure the selected error row is in visible range to user"
        n853 = Unbundle By Name(w2213) -> ("Coords.Error Display.Height"=w2210:i32)
        n854 = property on="Error Display" class="MCListbox (strict)"(error in=w2216) -> (error out=w2215:errorcluster, "Value"=w2214:i32)  [unwired: 1 in, 1 out]
        n855 = case shown="1, Default" w2214 {
          selector: w2214 -> [_ w2228]
          tunnel: [w2218 w2231] -> w2212
          tunnel: w2215 -> [w2219 w2229]
          tunnel: w2210 -> [_ w2225]
          tunnel: u32 0 ("Height") -> [_ w2220]
          frame -1, 0 {
            # "#coercion dot"
            # "-1 - no error to highlight, 0 - first row \nin both cases top row can be 0"
            n856 = property on="Error Display" class="MCListbox (strict)"(error in=w2219, "TopLeft"=cluster{"Row":u32, "Column":u32} {"Row"=0, "Column"=0} ("Top Left Visible Cell")) -> (error out=w2218:errorcluster)  [unwired: 1 in, 1 out]
          }
          frame 1, Default {
            # "#coercion dot"
            # "work backwards from selected towards top until the cumulative height of rows is greater than the control's height itself - which means the selected row will be in visible range to user and the row where we stopped should be the top row"
            n857 = while {
              shift-right: [w2238] -> _
              shift-left: w2228 -> [w2241]
              shift-right: [w2240] -> _
              shift-left: w2220 -> [w2243]
              tunnel: [w2241] -> w2223 if=w2239
              tunnel: w2229 -> [w2237]
              tunnel: [w2236] -> w2226
              tunnel: w2225 -> [w2235]
              tunnel: [w2233] -> w2221
              stop <- w2239 stop-if-true
              # "#coercion dot"
              n858 = Bundle By Name(cluster=cluster{"Row":i32, "Column":i32} {"Row"=0, "Column"=0} ("Active Cell:Active Cell"), "Row"=w2241) -> (w2245:cluster{"Row":i32, "Column":i32})
              n859 = property on="Error Display" class="MCListbox (strict)"(error in=w2237, "ActiveCell"=w2245) -> (error out=w2236:errorcluster, "CellSize"=w2244:T19)  [unwired: 1 in, 1 out]
              n860 = Decrement(x=w2241) -> (x-1=w2238:i32)
              n861 = To Unsigned Long Integer(number=w2235) -> (unsigned 32bit integer=w2232:u32)
              n862 = Unbundle By Name(w2244) -> ("Height"=w2242:u32)
              n863 = Add(x=w2243, y=w2242) -> (x+y=w2240:u32)
              n864 = Less Than 0?(x=w2238) -> (x < 0?=w2234:bool)
              n865 = Greater Or Equal?(x=w2240, y=w2232) -> (x >= y?=w2233:bool)
              n866 = Compound Arithmetic op=OR(w2233, w2234) -> (w2239:bool)
            }
            n867 = Increment(x=w2223) -> (x+1=w2222:i32)
            n868 = Select(t=w2222, s=w2221, f=w2223) -> (s? t:f=w2224:i32)
            n869 = Bundle By Name(cluster=cluster{"Row":i32, "Column":u32} {"Row"=0, "Column"=0} ("Top Left Visible Cell"), "Row"=w2224) -> (w2227:cluster{"Row":i32, "Column":u32})
            n870 = property on="Error Display" class="MCListbox (strict)"(error in=w2226, "TopLeft"=w2227) -> (error out=w2231:errorcluster)  [unwired: 1 in, 1 out]
          }
        }
      }
      frame "Update Error Display Scrollbar" {
        # "Determine if Error Display's scrollbar should be shown or not"
        n871 = property on="Error Display" class="MCListbox (strict)"(error in=w2255) -> (error out=w2251:errorcluster, "ItemNames"=w2257:string[][], "NumRows"=w2254:u32)  [unwired: 1 in, 1 out]
        n872 = Array Size(array=w2257) -> (size(s)=w2260:i32[])
        n873 = To Long Integer(number=w2254) -> (32bit integer=w2258:i32)
        n874 = Index Array(array=w2260) -> (element=w2247:i32)  [unwired: 1 in]
        n875 = Format Into String(format string="Errors (%d)", error in=w2251, w2247) -> (resulting string=w2252:string, error out=w2250:errorcluster)  [unwired: 1 in]
        n876 = Greater Than 0?(x=w2247) -> (x > 0?=w2248:bool)
        n877 = property on="Error Header" class="Str"(error in=w2250, "Value"=w2252, "Text.FontBold"=w2248) -> (error out=w2253:errorcluster)  [unwired: 1 in, 1 out]
        n878 = Greater Or Equal?(x=w2247, y=w2258) -> (x >= y?=w2259:bool)
        n879 = Bundle By Name(cluster=w2262, "Indices.No.Errors"=w2247) -> (w2256:T14)
        n880 = property on="Error Display" class="MCListbox (strict)"(error in=w2253, "VScrollVis"=w2259) -> (error out=w2261:errorcluster)  [unwired: 1 in, 1 out]
      }
      frame "Update Icon State" {
        # "Release the state of various boolean icons on UI post operation"
        n881 = Unbundle By Name(w2274) -> ("All Refs"=w2269:refnum<vi>[], "Action"=w2271:string, "Flags.Visibilty.Settings Icon"=w2265:bool)
        n882 = case shown="\"Power Down Help\"" w2271 {
          tunnel: [_ 4 6 0 9 2 1 5] -> w2268
          tunnel: w2265 -> [_ _ w2276 _ _ _ _ _]
          tunnel: [_ _ w2276 _ _ _ _ _] -> w2264
          frame Default {
          }
          frame "Delete" {
          }
          frame "Settings" {
          }
          frame "Help" {
          }
          frame "Power Down Help" {
          }
          frame "Down" {
          }
          frame "Up" {
          }
          frame "Add" {
          }
        }
        n883 = Index Array(array=w2269, index=w2268) -> (element=w2267:refnum<vi>)
        n884 = To Variant(anything=w2264) -> (Variant=w2263:variant)
        n885 = property on="Property Node" class="Ctl"(reference=w2267, error in=w2266, "Value"=w2263) -> (error out=w2270:errorcluster)  [unwired: 1 out]
        n886 = Bundle By Name(cluster=w2274, "Action"="") -> (w2273:T14)
      }
      frame "Check Limits" {
        # "0 - DC Voltage\n1 - DC Currrent"
        # "lower limits"
        # "upper limits"
        # "Check for out of range and update pin configuration of selected pin"
        n887 = Unbundle By Name(w2287) -> ("Pin Config.Source Pin Config"=w2289:T5[], "Indices.Actual Sel Row"=w2288:i32)
        n888 = Index Array(array=w2289, index=w2288) -> (element=w2293:T5)
        n889 = Unbundle By Name(w2293) -> ("Source Mode"=w2284:T6, "START VALUE"=w2299:dbl, "TARGET VALUE"=w2298:dbl, "COMPLIANCE LIMIT"=w2297:dbl)
        n890 = Index Array(array=dbl[][] [[200.0, 200.0, 3.0], [3.0, 3.0, 200.0]], index (row)=w2284) -> (element=w2294:dbl[])  [unwired: 1 in]
        n891 = Index Array(array=dbl[][] [[-200.0, -200.0, 0.0], [-3.0, -3.0, 0.0]], index (row)=w2284) -> (element=w2283:dbl[])  [unwired: 1 in]
        n892 = Build Array(w2299, w2298, w2297) -> (w2296:dbl[])
        n893 = for {
          tunnel: w2296 -> [w2308] mode=indexing
          tunnel: w2294 -> [w2309] mode=indexing
          shift-right: [w2312] -> w2292
          shift-left: w2293 -> [w2313]
          tunnel: [w2311] -> w2291 mode=indexing
          tunnel: w2283 -> [w2310] mode=indexing
          i -> [w2314]
          # "for each parameter to be checked for limits"
          n894 = In Range and Coerce(upper limit=w2309, x=w2308, lower limit=w2310) -> (In Range?=w2311:bool)  [unwired: 1 out]
          n895 = case shown="False" w2311 {
            tunnel: w2314 -> [w2320 _]
            tunnel: w2313 -> [w2319 w2339]
            tunnel: [w2318 w2339] -> w2312
            tunnel: w2310 -> [w2317 _]
            tunnel: w2309 -> [w2316 _]
            tunnel: w2308 -> [w2315 _]
            frame False {
              # "Out of range - coerced - update config"
              n896 = case shown="-1, Default" w2320 {
                tunnel: w2319 -> [w2321 w2328 w2331 w2338]
                tunnel: [w2321 w2327 w2330 w2337] -> w2318
                tunnel: w2317 -> [_ w2325 _ w2334]
                tunnel: w2316 -> [_ w2324 w2329 w2333]
                tunnel: w2315 -> [_ w2322 _ w2335]
                frame -1, Default {
                }
                frame 0 {
                  # "Start Value"
                  n897 = Less Than 0?(x=w2322) -> (x < 0?=w2326:bool)
                  n898 = Select(t=w2325, s=w2326, f=w2324) -> (s? t:f=w2323:dbl)
                  n899 = Bundle By Name(cluster=w2328, "START VALUE"=w2323) -> (w2327:T5)
                }
                frame 2 {
                  # "Compliance Limit"
                  n900 = Bundle By Name(cluster=w2331, "COMPLIANCE LIMIT"=w2329) -> (w2330:T5)
                }
                frame 1 {
                  # "Target Value"
                  n901 = Less Than 0?(x=w2335) -> (x < 0?=w2336:bool)
                  n902 = Select(t=w2334, s=w2336, f=w2333) -> (s? t:f=w2332:dbl)
                  n903 = Bundle By Name(cluster=w2338, "TARGET VALUE"=w2332) -> (w2337:T5)
                }
              }
            }
            frame True {
            }
          }
        }
        n904 = And Array Elements(Boolean array=w2291) -> (logical AND=w2290:bool)
        n905 = case shown="False" w2290 {
          tunnel: w2287 -> [w2306 w2307]
          tunnel: [w2305 w2307] -> w2286
          tunnel: w2292 -> [w2302 _]
          tunnel: w2289 -> [w2304 _]
          tunnel: w2288 -> [w2303 _]
          frame False {
            # "coercion happened - update configuration"
            n906 = Replace Array Subset(array=w2304, new element=w2302, index=w2303) -> (w2301:T5[])
            n907 = Bundle By Name(cluster=w2306, "Pin Config.Active Pin Config"=w2302, "Pin Config.Source Pin Config"=w2301) -> (w2305:T14)
          }
          frame True {
          }
        }
      }
      frame "Update Active Pin Config" {
        # "Note - Config should be set after setting limits. Do not change!"
        # "#coercion dots 4"
        # "Update UI with selected source pin configuration, set appropriate limits and units"
        n908 = Unbundle By Name(w2379) -> ("Pin Config.Source Pin Config"=w2378:T5[], "Indices.Actual Sel Row"=w2360:i32)
        n909 = Equal To 0?(x=w2360) -> (x = 0?=w2357:bool)
        n910 = Greater Or Equal To 0?(x=w2360) -> (x >= 0?=w2369:bool)
        n911 = Select(t=u8 2, s=w2357, f=u8 0) -> (s? t:f=w2353:u8)
        n912 = Index Array(array=w2378, index=w2360) -> (element=w2340:T5)
        n913 = property on="Previous source end" class="Bool (strict)"(error in=w2356, "DisabledEnum"=w2353) -> (error out=w2354:errorcluster)  [unwired: 1 in, 1 out]
        n914 = property on="Previous source start" class="Bool (strict)"(error in=w2356, "DisabledEnum"=w2353) -> (error out=w2355:errorcluster)  [unwired: 1 in, 1 out]
        n915 = Select(t=enum32{"Default", "Config"}."Config" ("Tab"), s=w2369, f=enum32{"Default", "Config"}."Default") -> (s? t:f=w2368:enum32{"Default", "Config"})
        n916 = Unbundle By Name(w2340) -> ("Pin"=w2347:string, "Source Mode"=w2377:T6, "DEFAULT RAMP RATE"=w2365:bool)
        n917 = Bundle By Name(cluster=w2379, "Pin Config.Active Pin Config"=w2340) -> (w2376:T14)
        n918 = local write "Tab"(w2368) -> ()
        n919 = Merge Errors(w2355, w2354) -> (w2361:errorcluster)
        n920 = case shown="0" w2377 {
          tunnel: ["%_6p V" ("Format String") w2392 "%_6p A" ("Format String")] -> w2352
          tunnel: ["%_6p V/us" ("Format String") w2392 "%_6p A/us" ("Format String")] -> w2373
          tunnel: ["%_6p A" ("Format String") w2392 "%_6p V" ("Format String")] -> w2372
          tunnel: [-200.0 0.0 -3.0] -> w2349
          tunnel: [3.0 0.0 200.0] -> w2371
          frame 0 {
            # "DC Voltage mode"
          }
          frame Default {
            w2392 = "" ("Format String")
          }
          frame 1 {
            # "DC Current mode"
          }
        }
        n921 = Empty String/Path?(string/path=w2347) -> (empty?=w2346:bool)
        n922 = Select(t=u8 2, s=w2365, f=u8 0) -> (s? t:f=w2363:u8)
        n923 = property on="RAMP RATE" class="DigNum (strict)"(error in=w2361, "DisabledEnum"=w2363) -> (error out=w2366:errorcluster)  [unwired: 1 in, 1 out]
        n924 = case shown="True" w2346 {
          tunnel: ["" ("Pin") "<empty>" ("Pin")] -> w2345
          tunnel: [FALSE TRUE] -> w2344
          frame False {
            # "non empty pin name"
          }
          frame True {
            # "empty pin - display <empty>"
          }
        }
        n925 = Absolute Value(x=w2349) -> (abs(x)=w2348:dbl)
        n926 = property on="TARGET VALUE" class="DigNum (strict)"(error in=w2366, "FormatString"=w2352, "Minimum"=w2349, "Maximum"=w2348) -> (error out=w2351:errorcluster)  [unwired: 1 in, 1 out]
        n927 = property on="START VALUE" class="DigNum (strict)"(error in=w2351, "FormatString"=w2352, "Minimum"=w2349, "Maximum"=w2348) -> (error out=w2350:errorcluster)  [unwired: 1 in, 1 out]
        n928 = property on="RAMP RATE" class="DigNum (strict)"(error in=w2350, "FormatString"=w2373) -> (error out=w2375:errorcluster)  [unwired: 1 in, 1 out]
        n929 = property on="COMPLIANCE LIMIT" class="DigNum (strict)"(error in=w2375, "FormatString"=w2372, "Minimum"=0.0 ("Data Entry Limits:Minimum"), "Maximum"=w2371) -> (error out=w2374:errorcluster)  [unwired: 1 in, 1 out]
        n930 = property on="Pin" class="Str"(error in=w2374, "Caption.Text"=w2345, "Caption.Visible"=w2344) -> (error out=w2342:errorcluster)  [unwired: 1 in, 1 out]
        n931 = flat-sequence {
          tunnel: [w2381] -> w2341
          tunnel: w2342 -> [w2381]
          tunnel: w2340 -> [w2380]
          frame #0 {
            n932 = local write "Pin Config"(w2380) -> ()
          }
        }
      }
      frame "Update Meas Config" {
        # "#coercion 4 dots"
        # "Update the controls of Measurement Configuration.ctl for pin configuration"
        n933 = Unbundle By Name(w2415) -> ("Pin Config.Source Pin Config"=w2416:T5[])
        n934 = for {
          tunnel: w2416 -> [w2441] mode=indexing
          tunnel: [w2434] -> w2407 mode=indexing
          tunnel: [w2440] -> w2402 mode=indexing
          tunnel: [w2439] -> w2408 mode=indexing
          tunnel: [w2438] -> w2410 mode=indexing
          tunnel: [w2437] -> w2411 mode=indexing
          tunnel: [w2436] -> w2412 mode=indexing
          tunnel: [w2435] -> w2413 mode=indexing
          tunnel: [w2433] -> w2405 mode=indexing
          tunnel: [w2432] -> w2406 mode=indexing
          tunnel: [w2431] -> w2404 mode=indexing
          tunnel: [w2430] -> w2403 mode=indexing
          n935 = Unbundle By Name(w2441) -> ("TRANSIENT RESPONSE"=w2431:T9, "SENSE MODE"=w2432:T8, "DEFAULT RAMP RATE"=w2433:bool, "Pin"=w2434:string, "TARGET VALUE"=w2440:dbl, "RAMP RATE"=w2439:dbl, "COMPLIANCE LIMIT"=w2438:dbl, "START DELAY"=w2437:dbl, "RELATIVE TO"=w2436:T7, "Source Mode"=w2435:T6, "START VALUE"=w2430:dbl)
        }
        n936 = Absolute Value(x=w2403) -> (abs(x)=w2399:dbl[])
        n937 = Absolute Value(x=w2402) -> (abs(x)=w2400:dbl[])
        n938 = for {
          tunnel: w2399 -> [w2423] mode=indexing
          tunnel: w2400 -> [w2422] mode=indexing
          tunnel: [w2418] -> w2401
          stop <- w2417 stop-if-true
          n939 = Subtract(x=w2422, y=w2423) -> (x-y=w2421:dbl)
          n940 = Sign(1:w2421) -> (0:w2420:dbl)
          n941 = To Long Integer(number=w2420) -> (32bit integer=w2419:i32)
          n942 = case shown="0, Default" w2419 {
            tunnel: [TRUE FALSE TRUE] -> w2418
            tunnel: [FALSE TRUE TRUE] -> w2417
            frame 0, Default {
            }
            frame 1 {
              # "target>start"
            }
            frame -1 {
              # "target<start"
            }
          }
        }
        "Power Up/Down" <- w2401
        n943 = local write "Transient Response"(w2404) -> ()
        n944 = local write "Start Value"(w2403) -> ()
        n945 = local write "Target Value"(w2402) -> ()
        n946 = local write "Relative To"(w2412) -> ()
        n947 = local write "Sense Mode"(w2406) -> ()
        n948 = local write "Default Ramp Rate"(w2405) -> ()
        n949 = local write "Ramp Rate"(w2408) -> ()
        n950 = local write "Start Delay"(w2411) -> ()
        n951 = local write "Source Mode"(w2413) -> ()
        n952 = local write "Pin Name"(w2407) -> ()
        n953 = local write "Compliance Limit"(w2410) -> ()
        n954 = Bundle By Name(cluster=w2415, "Pin Config.ML Config.Transient Response"=w2404, "Pin Config.ML Config.Sense Mode"=w2406, "Pin Config.ML Config.Default Ramp Rate"=w2405, "Pin Config.ML Config.Pin Name"=w2407, "Pin Config.ML Config.Target Value"=w2402, "Pin Config.ML Config.Ramp Rate"=w2408, "Pin Config.ML Config.Compliance Limit"=w2410, "Pin Config.ML Config.Start Delay"=w2411, "Pin Config.ML Config.Relative To"=w2412, "Pin Config.ML Config.Source Mode"=w2413, "Pin Config.Power Up/Down"=w2401) -> (w2414:T14)
      }
      frame "Update Meas Config - 2" {
        # "Update the controls of Measurement Configuration.ctl for advanced settings"
        n955 = Unbundle By Name(w2444) -> ("Adv Settings.Adv Setting.Power line frequency"=w2442:T11, "Adv Settings.Adv Setting.Data Capture"=w2443:bool)
        n956 = local write "Power line frequency"(w2442) -> ()
        n957 = local write "Data Capture"(w2443) -> ()
      }
      frame "Validate Inputs" {
        # "Validate pin sequence parameters"
        n958 = Unbundle By Name(w2465) -> ("Indices.Row No Ref"=w2452:u32, "Flags.Check All?"=w2455:bool, "Pin Config.Error Info"=w2457:string[], "Error Map"=w2458:map{i32, string}, "Flags.Check All?"=w2450:bool, "Indices.Actual Sel Row"=w2449:i32, "Pinmap List"=w2464:string[], "Pin Config.ML Config.Pin Name"=w2463:string[], "Pin Config.Source Pin Config"=w2462:T5[], "Pin Config.Power Up/Down"=w2448:bool)
        n959 = To Long Integer(number=w2452) -> (32bit integer=w2451:i32)
        n960 = Not(x=w2448) -> (.not. x?=w2446:bool)
        n961 = Select(t=w2451, s=w2455, f=1) -> (s? t:f=w2454:i32)
        n962 = for {
          N: w2454 -> [_]
          tunnel: w2464 -> [w2491]
          tunnel: w2463 -> [w2489]
          tunnel: w2458 -> [w2486]
          tunnel: w2462 -> [w2477]
          shift-right: [w2484] -> w2459
          shift-left: w2460 -> [w2485]
          shift-right: [w2481] -> w2456
          shift-left: w2457 -> [w2482]
          tunnel: w2450 -> [w2479]
          tunnel: w2449 -> [w2478]
          tunnel: w2446 -> [w2472]
          i -> [w2480]
          # "for each pin the 'Source Pin Sequence'"
          n963 = Select(t=w2480, s=w2479, f=w2478) -> (s? t:f=w2474:i32)
          n964 = Index Array(array=w2477, index=w2474) -> (element=w2476:T5)
          n965 = Unbundle By Name(w2476) -> ("DEFAULT RAMP RATE"=w2492:bool, "Pin"=w2493:string, "TARGET VALUE"=w2494:dbl, "RAMP RATE"=w2495:dbl, "COMPLIANCE LIMIT"=w2496:dbl, "RELATIVE TO"=w2475:T7, "START VALUE"=w2471:dbl)
          n966 = Delete From Array(array=w2489, index=w2474) -> (array with subset deleted=w2483:string[])  [unwired: 1 in, 1 out]
          n967 = Absolute Value(x=w2494) -> (abs(x)=w2469:dbl)
          n968 = Absolute Value(x=w2471) -> (abs(x)=w2470:dbl)
          n969 = for {
            N: 8 -> [_]
            tunnel: w2496 -> [w2505]
            tunnel: w2495 -> [w2507]
            tunnel: w2469 -> [w2508]
            tunnel: w2493 -> [w2513]
            tunnel: w2492 -> [w2506]
            tunnel: w2486 -> [w2511]
            tunnel: [w2510] -> w2487 mode=indexing if=w2501
            tunnel: w2491 -> [w2512]
            tunnel: w2483 -> [w2509]
            shift-right: [w2503] -> w2484
            shift-left: w2485 -> [w2504]
            tunnel: w2475 -> [w2500]
            tunnel: w2474 -> [w2499]
            tunnel: w2472 -> [w2498]
            tunnel: w2470 -> [w2497]
            i -> [w2502]
            # "for each possible error check"
            n970 = case shown="1" w2502 {
              tunnel: w2513 -> [w2516 w2518 w2525 _ _ _ _ _ _]
              tunnel: [w2515 w2519 w2526 w2535 w2541 w2545 w2549 w2551 FALSE] -> w2501
              tunnel: w2512 -> [_ w2523 _ _ _ _ _ _ _]
              tunnel: w2509 -> [_ _ w2528 _ _ _ _ _ _]
              tunnel: w2508 -> [_ _ _ w2533 w2537 _ _ _ _]
              tunnel: w2507 -> [_ _ _ _ _ _ w2547 _ _]
              tunnel: w2506 -> [_ _ _ _ _ _ w2548 _ _]
              tunnel: w2505 -> [_ _ _ _ _ w2544 _ _ _]
              tunnel: w2504 -> [w2514 w2520 w2527 w2536 w2542 w2543 w2546 w2556 w2558]
              tunnel: [w2514 w2520 w2527 w2536 w2542 w2543 w2546 w2556 w2558] -> w2503
              tunnel: w2500 -> [_ _ _ _ _ _ _ w2554 _]
              tunnel: w2499 -> [_ _ _ _ _ _ _ w2555 _]
              tunnel: w2498 -> [_ _ _ w2534 w2540 _ _ _ _]
              tunnel: w2497 -> [_ _ _ w2532 w2538 _ _ _ _]
              frame 0 {
                # "Check for non-empty pin name"
                n971 = Empty String/Path?(string/path=w2516) -> (empty?=w2515:bool)
              }
              frame 1 {
                # "pin name should be \nlisted in pinmap list"
                # "Check for valid pin name"
                n972 = Search 1D Array(1D array=w2523, element=w2518) -> (index of element=w2522:i32)  [unwired: 1 in]
                n973 = Empty String/Path?(string/path=w2518) -> (empty?=w2517:bool)
                n974 = Less Than 0?(x=w2522) -> (x < 0?=w2521:bool)
                n975 = Compound Arithmetic op=AND(w2521, invert w2517) -> (w2519:bool)
              }
              frame 2 {
                # "Check for duplicate pin name"
                n976 = Search 1D Array(1D array=w2528, element=w2525) -> (index of element=w2530:i32)  [unwired: 1 in]
                n977 = Empty String/Path?(string/path=w2525) -> (empty?=w2524:bool)
                n978 = Greater Or Equal To 0?(x=w2530) -> (x >= 0?=w2529:bool)
                n979 = Compound Arithmetic op=AND(w2529, invert w2524) -> (w2526:bool)
              }
              frame 3 {
                # "Check target>=start for power up"
                n980 = Less?(x=w2533, y=w2532) -> (x < y?=w2531:bool)
                n981 = Compound Arithmetic op=AND(w2531, w2534) -> (w2535:bool)
              }
              frame 4 {
                # "Check start>=target for power down"
                n982 = Less?(x=w2538, y=w2537) -> (x < y?=w2539:bool)
                n983 = Compound Arithmetic op=AND(w2539, invert w2540) -> (w2541:bool)
              }
              frame 5 {
                # "Check non-zero Compliance Limit"
                n984 = Equal To 0?(x=w2544) -> (x = 0?=w2545:bool)
              }
              frame 6 {
                # "Check non-zero Ramp Rate"
                n985 = Equal To 0?(x=w2547) -> (x = 0?=w2550:bool)
                n986 = Compound Arithmetic op=AND(invert w2548, w2550) -> (w2549:bool)
              }
              frame 7 {
                # "Relative To"
                n987 = Equal To 0?(x=w2555) -> (x = 0?=w2553:bool)
                n988 = Not Equal To 0?(x=w2554) -> (x != 0?=w2552:bool)
                n989 = Compound Arithmetic op=AND(w2553, w2552) -> (w2551:bool)
              }
              frame Default {
              }
            }
            n990 = Look In Map(map=w2511, key=w2502) -> (value=w2510:string)  [unwired: 1 in, 1 out]
          }
          n991 = Array To Spreadsheet String(delimiter (Tab)="\n    ", array=w2487, 3:"" ("format string")) -> (spreadsheet string=w2467:string)
          n992 = Match Pattern(string=w2467, regular expression="[\\t\\n\\r\\s]*$") -> (before substring=w2466:string)  [unwired: 1 in, 3 out]
          n993 = Replace Array Subset(array=w2482, new element=w2466, index=w2474) -> (w2481:string[])
        }
        n994 = Bundle By Name(cluster=w2465, "Pin Config.Error Info"=w2456, "Flags.Check All?"=FALSE) -> (w2461:T14)
      }
      frame "Update Voltage Measurements" {
        w2567 = -1  # Last Index
        # "Update the voltage measurement results"
        n995 = property on="Voltage Measurements" class="Arr (strict)"(error in=w2560) -> (error out=w2573:errorcluster, "Value"=w2570:dbl[])  [unwired: 1 in, 1 out]
        n996 = property on="Indices" class="Arr (strict)"(error in=w2573) -> (error out=w2569:errorcluster, "Value"=w2568:i32[])  [unwired: 1 in, 1 out]
        n997 = Unbundle By Name(w2571) -> ("Legend.Voltage (V)"=w2561:T13[], "Pin Config.Source Pin Config"=w2563:T5[], "Pin Config.Color Array"=w2562:T3)
        n998 = property on="dt values" class="Arr (strict)"(error in=w2569) -> (error out=w2565:errorcluster, "Value"=w2566:dbl[])  [unwired: 1 in, 1 out]
        n999 = for {
          tunnel: w2570 -> [w2590]
          tunnel: w2568 -> [w2586] mode=indexing
          shift-right: [w2584] -> _
          shift-left: w2567 -> [w2588]
          tunnel: w2566 -> [w2587] mode=indexing
          tunnel: [w2585] -> w2559 mode=indexing
          tunnel: w2565 -> [w2583]
          tunnel: [w2581] -> w2564 mode=indexing
          tunnel: w2563 -> [w2578] mode=indexing
          tunnel: w2562 -> [w2579] mode=indexing
          tunnel: w2561 -> [w2576] mode=indexing
          i -> [w2582]
          n1000 = Unbundle By Name(w2578) -> ("Pin"=w2577:string)
          n1001 = Unbundle By Name(w2576) -> ("Visible"=w2575:bool)
          n1002 = Not Equal?(x=w2588, y=w2586) -> (x != y?=w2589:bool)
          n1003 = case shown="True" w2589 {
            tunnel: w2590 -> [_ w2602]
            tunnel: w2588 -> [w2591 w2593]
            tunnel: w2586 -> [_ w2601]
            tunnel: w2587 -> [_ w2600]
            tunnel: [waveform(dbl) {"t0"=timestamp(0 s since 1904-01-01), "dt"=1.0, "Y"=[]} w2599] -> w2585
            tunnel: [w2591 w2597] -> w2584
            frame False {
              # "empty waveform"
            }
            frame True {
              # "Get waveform data using indices"
              n1004 = Subtract(x=w2601, y=w2593) -> (x-y=w2594:i32)
              n1005 = Increment(x=w2593) -> (x+1=w2598:i32)
              n1006 = Array Subset(array=w2602, index=w2598, length=w2594) -> (w2596:dbl[])
              n1007 = Bundle By Name ("Build Waveform")(cluster=waveform(dbl) {"t0"=timestamp(0 s since 1904-01-01), "dt"=1.0, "Y"=[]} ("waveform"), "Y"=w2596, "dt"=w2600) -> (w2599:waveform(dbl))
              n1008 = Add(x=w2593, y=w2594) -> (x+y=w2597:i32)
            }
          }
          n1009 = To Unsigned Long Integer(number=w2582) -> (unsigned 32bit integer=w2580:u32)
          n1010 = property on="Voltage" class="WFGraph (strict)"(error in=w2583, "Active Plot"=w2580, "Plot.Visible?"=w2575, "Plot.Plot Name"=w2577, "Plot.Plot Color"=w2579, "XScale.ScaleFit"=u8 2 ("X Scale.Scale Fit")) -> (error out=w2581:errorcluster)  [unwired: 1 in, 1 out]
        }
        "Voltage" <- w2559
        n1011 = Merge Errors(w2564) -> (w2572:errorcluster)
      }
      frame "Update Current Measurements" {
        w2611 = -1  # Last Index
        # "Update the current measurement results"
        n1012 = property on="Current Measurements" class="Arr (strict)"(error in=w2616) -> (error out=w2617:errorcluster, "Value"=w2603:dbl[])  [unwired: 1 in, 1 out]
        n1013 = property on="Indices" class="Arr (strict)"(error in=w2617) -> (error out=w2613:errorcluster, "Value"=w2612:i32[])  [unwired: 1 in, 1 out]
        n1014 = Unbundle By Name(w2614) -> ("Legend.Current (A)"=w2605:T13[], "Pin Config.Source Pin Config"=w2607:T5[], "Pin Config.Color Array"=w2606:T3)
        n1015 = property on="dt values" class="Arr (strict)"(error in=w2613) -> (error out=w2609:errorcluster, "Value"=w2610:dbl[])  [unwired: 1 in, 1 out]
        n1016 = for {
          tunnel: w2603 -> [w2633]
          tunnel: w2612 -> [w2629] mode=indexing
          shift-right: [w2627] -> _
          shift-left: w2611 -> [w2631]
          tunnel: w2610 -> [w2630] mode=indexing
          tunnel: [w2628] -> w2604 mode=indexing
          tunnel: w2609 -> [w2626]
          tunnel: [w2624] -> w2608 mode=indexing
          tunnel: w2607 -> [w2622] mode=indexing
          tunnel: w2606 -> [w2621] mode=indexing
          tunnel: w2605 -> [w2619] mode=indexing
          i -> [w2625]
          n1017 = Unbundle By Name(w2619) -> ("Visible"=w2618:bool)
          n1018 = Unbundle By Name(w2622) -> ("Pin"=w2620:string)
          n1019 = Not Equal?(x=w2631, y=w2629) -> (x != y?=w2632:bool)
          n1020 = To Unsigned Long Integer(number=w2625) -> (unsigned 32bit integer=w2623:u32)
          n1021 = case shown="True" w2632 {
            tunnel: w2633 -> [_ w2645]
            tunnel: w2631 -> [w2634 w2636]
            tunnel: w2629 -> [_ w2644]
            tunnel: w2630 -> [_ w2643]
            tunnel: [waveform(dbl) {"t0"=timestamp(0 s since 1904-01-01), "dt"=1.0, "Y"=[]} w2642] -> w2628
            tunnel: [w2634 w2640] -> w2627
            frame False {
              # "empty waveform"
            }
            frame True {
              # "Get waveform data using indices"
              n1022 = Subtract(x=w2644, y=w2636) -> (x-y=w2637:i32)
              n1023 = Increment(x=w2636) -> (x+1=w2641:i32)
              n1024 = Array Subset(array=w2645, index=w2641, length=w2637) -> (w2639:dbl[])
              n1025 = Bundle By Name ("Build Waveform")(cluster=waveform(dbl) {"t0"=timestamp(0 s since 1904-01-01), "dt"=1.0, "Y"=[]} ("waveform"), "Y"=w2639, "dt"=w2643) -> (w2642:waveform(dbl))
              n1026 = Add(x=w2636, y=w2637) -> (x+y=w2640:i32)
            }
          }
          n1027 = property on="Current" class="WFGraph (strict)"(error in=w2626, "Active Plot"=w2623, "Plot.Visible?"=w2618, "Plot.Plot Name"=w2620, "Plot.Plot Color"=w2621) -> (error out=w2624:errorcluster)  [unwired: 1 in, 1 out]
        }
        "Current" <- w2604
        n1028 = Merge Errors(w2608) -> (w2615:errorcluster)
      }
      frame "Update Errors from Core Logic" {
        # "Store warnings/error info from Core Logic"
        n1029 = Unbundle By Name(w2649) -> ("Pin Config.Error Info"=w2648:string[])
        n1030 = property on="Warning" class="Arr (strict)"(error in=w2653) -> (error out=w2652:errorcluster, "Value"=w2647:string[])  [unwired: 1 in, 1 out]
        n1031 = Empty Array?(array=w2647) -> (empty?=w2650:bool)
        n1032 = Select(t=w2648, s=w2650, f=w2647) -> (s? t:f=w2646:string[])
        n1033 = Bundle By Name(cluster=w2649, "Pin Config.Error Info"=w2646) -> (w2651:T14)
      }
      frame "Update Power Down State" {
        # "disable it by default"
        # "Enable Power Down only if-\n-it is power up seq\n- power up is sucessful"
        # "#coercion dot 2"
        # "Determine the state of Power Down icon"
        n1034 = property on="Power Down" class="Bool (strict)"(error in=w2660, "DisabledEnum"=u8 2 ("f"), "Value"=FALSE ("POWER DOWN")) -> (error out=w2659:errorcluster)  [unwired: 1 in, 1 out]
        n1035 = Unbundle By Name(w2667) -> ("Pin Config.ML Config.Power Down"=w2661:bool, "Flags.P.up Success?"=w2654:bool, "Pin Config.Power Up/Down"=w2662:bool)
        n1036 = property on="Operation Complete?" class="Bool (strict)"(error in=w2659) -> (error out=w2658:errorcluster, "Value"=w2655:bool)  [unwired: 1 in, 1 out]
        n1037 = property on="Voltage Measurements" class="Arr (strict)"(error in=w2658) -> (error out=w2656:errorcluster, "Value"=w2657:dbl[])  [unwired: 1 in, 1 out]
        n1038 = case shown="False" w2655 {
          tunnel: w2667 -> [w2675 w2689]
          tunnel: [w2669 w2688] -> w2666
          tunnel: [w2674 w2687] -> w2663
          tunnel: w2662 -> [_ w2686]
          tunnel: w2661 -> [_ w2685]
          tunnel: w2657 -> [w2673 w2684]
          tunnel: w2656 -> [w2669 w2683]
          tunnel: w2654 -> [w2668 _]
          frame False {
            n1039 = Empty Array?(array=w2673) -> (empty?=w2672:bool)
            n1040 = Select(t=FALSE, s=w2672, f=w2668) -> (s? t:f=w2670:bool)
            n1041 = Bundle By Name(cluster=w2675, "Flags.P.up Success?"=w2670) -> (w2674:T14)
          }
          frame True {
            w2680 = FALSE
            # "power up - false\npower down - true"
            n1042 = Empty Array?(array=w2684) -> (empty?=w2682:bool)
            n1043 = Compound Arithmetic op=AND(invert w2685, invert w2686, invert w2682) -> (w2681:bool)
            n1044 = Select(t=u8 0, s=w2681, f=u8 2) -> (s? t:f=w2676:u8)
            n1045 = local write "Quick Power Down"(w2680) -> ()
            n1046 = property on="Power Down" class="Bool (strict)"(error in=w2683, "DisabledEnum"=w2676, "Value"=FALSE ("POWER DOWN")) -> (error out=w2688:errorcluster)  [unwired: 1 in, 1 out]
            n1047 = Bundle By Name(cluster=w2689, "Pin Config.ML Config.Power Down"=w2680, "Flags.P.up Success?"=w2681) -> (w2687:T14)
          }
        }
      }
      frame "Update Power Down" {
        w2691 = FALSE ("Pin Config.ML Config.Power Down")
        # "Enable Power Down only if-\n-it is power up seq\n- power up is sucessful"
        # "#coercion dot 1"
        n1048 = property on="Power Down" class="Bool (strict)"(error in=w2694, "DisabledEnum"=u8 2, "Value"=FALSE ("POWER DOWN")) -> (error out=w2696:errorcluster)  [unwired: 1 in, 1 out]
        n1049 = local write "Quick Power Down"(w2691) -> ()
        n1050 = Bundle By Name(cluster=w2693, "Pin Config.ML Config.Power Down"=w2691) -> (w2692:T14)
      }
      frame "Update Plot Visibility" {
        # "Update Plot Names, Visibility and Colors in Plot Legend for graphs"
        n1051 = Unbundle By Name(w2701) -> ("Legend.Voltage (V)"=w2699:T13[], "Legend.Current (A)"=w2702:T13[])
        n1052 = for {
          tunnel: [w2708] -> w2698
          tunnel: w2700 -> [w2710]
          tunnel: w2702 -> [w2709] mode=indexing
          i -> [w2707]
          n1053 = Unbundle By Name(w2709) -> ("Name"=w2705:string, "Color"=w2704:u32, "Visible"=w2703:bool)
          n1054 = To Unsigned Long Integer(number=w2707) -> (unsigned 32bit integer=w2706:u32)
          n1055 = property on="Current" class="WFGraph (strict)"(error in=w2710, "Active Plot"=w2706, "Plot.Plot Name"=w2705, "Plot.Plot Color"=w2704, "Plot.Visible?"=w2703) -> (error out=w2708:errorcluster)  [unwired: 1 in, 1 out]
        }
        n1056 = for {
          tunnel: [w2716] -> w2697
          tunnel: w2698 -> [w2718]
          tunnel: w2699 -> [w2717] mode=indexing
          i -> [w2715]
          n1057 = Unbundle By Name(w2717) -> ("Name"=w2713:string, "Color"=w2712:u32, "Visible"=w2711:bool)
          n1058 = To Unsigned Long Integer(number=w2715) -> (unsigned 32bit integer=w2714:u32)
          n1059 = property on="Voltage" class="WFGraph (strict)"(error in=w2718, "Active Plot"=w2714, "Plot.Plot Name"=w2713, "Plot.Plot Color"=w2712, "Plot.Visible?"=w2711) -> (error out=w2716:errorcluster)  [unwired: 1 in, 1 out]
        }
      }
      frame "Update Default Ramp Rate" {
        # "Update Default Ramp Rate and Actual Ramp Rate values from Core Logic"
        n1060 = property on="Default Ramp Rate?" class="Arr (strict)"(error in=w2722) -> (error out=w2721:errorcluster, "Value"=w2720:bool[])  [unwired: 1 in, 1 out]
        n1061 = Empty Array?(array=w2720) -> (empty?=w2719:bool)
        n1062 = case shown="False" w2719 {
          tunnel: [w2730 w2744] -> w2724
          tunnel: w2721 -> [w2733 w2744]
          tunnel: w2720 -> [w2726 _]
          tunnel: w2725 -> [w2729 w2743]
          tunnel: [w2727 w2743] -> w2723
          frame False {
            n1063 = property on="Actual Ramp Rates" class="Arr (strict)"(error in=w2733) -> (error out=w2730:errorcluster, "Value"=w2731:dbl[])  [unwired: 1 in, 1 out]
            n1064 = Unbundle By Name(w2729) -> ("Pin Config.Source Pin Config"=w2732:T5[])
            n1065 = for {
              tunnel: w2732 -> [w2737] mode=indexing
              tunnel: w2731 -> [w2736] mode=indexing
              tunnel: [w2735] -> w2728 mode=indexing
              tunnel: w2726 -> [w2734] mode=indexing
              n1066 = case shown="True" w2734 {
                selector: w2734 -> [_ w2739]
                tunnel: w2737 -> [w2738 w2742]
                tunnel: w2736 -> [_ w2741]
                tunnel: [w2738 w2740] -> w2735
                frame False {
                }
                frame True {
                  n1067 = Bundle By Name(cluster=w2742, "DEFAULT RAMP RATE"=w2739, "RAMP RATE"=w2741) -> (w2740:T5)
                }
              }
            }
            n1068 = Bundle By Name(cluster=w2729, "Pin Config.Source Pin Config"=w2728) -> (w2727:T14)
          }
          frame True {
          }
        }
      }
      frame "--- Measurement Link Operations ---" {
      }
      frame "Post UI Update" {
        # "This case will be triggered, after framework updates the User interface with result values."
        n1069 = for {
          shift-right: [w2755] -> w2748
          shift-left: w2751 -> [w2756]
          tunnel: w2749 -> [w2754]
          tunnel: string[] ["Update Power Down State", "Check for Changes - 1", "Check for Changes - 2", "Restore Formatting", "Re-shuffle Plot Colors", "Generate Plot Colors", "Update Voltage Measurements", "Update Current Measurements", "Reset Graph Scales", "Update Default Ramp Rate", "Update Errors from Core Logic", "Update Error Info", "Update Error Display Top Row", "Update Error Display Scrollbar", "Monitor Icons", "Update Adv Settings", "Check Limits", "Update Active Pin Config", "Update Meas Config"] -> [w2753] mode=indexing
          n1070 = Enqueue Element(queue=w2754, element=w2753, timeout in ms (-1)=50, error in (no error)=w2756) -> (error out=w2755:errorcluster)  [unwired: 2 out]
        }
      }
      frame "Update Adv Settings" {
        # "Store Adv Settings configuration"
        n1071 = Unbundle By Name(w2761) -> ("Flags.Adv Settings Change?"=w2763:bool, "Adv Settings.Adv Setting.Data Capture"=w2758:bool, "Adv Settings.Adv Setting.Power line frequency"=w2757:T11)
        n1072 = case shown="True" w2763 {
          tunnel: w2761 -> [w2765 w2782]
          tunnel: [w2765 w2781] -> w2759
          tunnel: w2762 -> [w2764 w2774]
          tunnel: [w2764 w2773] -> w2760
          tunnel: w2757 -> [_ w2771]
          tunnel: w2758 -> [_ w2770]
          frame False {
            # "no changes"
          }
          frame True {
            # "Changes exist in Adv Settings"
            n1073 = property on="Power line frequency" class="Ring (strict)"(error in=w2774) -> (error out=w2773:errorcluster, "Strings []"=w2772:string[])  [unwired: 1 in, 1 out]
            n1074 = To Long Integer(number=w2771) -> (32bit integer=w2778:i32)
            n1075 = Index Array(array=w2772, index=w2778) -> (element=w2775:string)
            n1076 = Concatenate Strings("Freq_" ("string"), w2775) -> (w2776:string)
            n1077 = Select(t=string[] ["Capture data"], s=w2770, f=string[] [] ("array")) -> (s? t:f=w2767:string[])
            n1078 = Insert Into Array(array=string[] [], new element=w2776) -> (w2780:string[])  [unwired: 1 in]
            n1079 = Bundle By Name(cluster=w2782, "Adv Settings.Setting.Sel.Main"=w2767, "Adv Settings.Setting.Sel.PL_Freq"=w2780, "Adv Settings.Adv Setting.Power line frequency"=w2771, "Adv Settings.Adv Setting.Data Capture"=w2770, "Flags.Visibilty.Plot Legend Scrollbar"=FALSE ("Flags.Adv Setting Change?")) -> (w2781:T14)
          }
        }
      }
      frame "--- Measurement Link Event Operations ---" {
      }
      frame "Check for Changes - 1" {
        # "#coercion  dot"
        # "Check for changes in pin sequence configuration"
        n1080 = Unbundle By Name(w2804) -> ("Pin Config.Source Pin Config"=w2797:T5[], "Pin Config.ML Config.Power Down"=w2785:bool)
        n1081 = property on="Power Down" class="Bool (strict)"(error in=w2803, "Val(Sgnl)"=w2785) -> (error out=w2786:errorcluster)  [unwired: 1 in, 1 out]
        n1082 = for {
          tunnel: "Ramp Rate" -> [w2825] mode=indexing
          tunnel: "Compliance Limit" -> [w2824] mode=indexing
          tunnel: "Start Delay" -> [w2823] mode=indexing
          tunnel: "Source Mode" -> [w2822] mode=indexing
          tunnel: "Target Value" -> [w2821] mode=indexing
          tunnel: [w2820] -> w2800 mode=indexing
          tunnel: w2797 -> [w2818]
          tunnel: [w2819] -> w2798 mode=indexing
          tunnel: "Pin Name" -> [w2816] mode=indexing
          tunnel: "Default Ramp Rate" -> [w2815] mode=indexing
          tunnel: "Sense Mode" -> [w2814] mode=indexing
          tunnel: "Relative To" -> [w2811] mode=indexing
          tunnel: "Transient Response" -> [w2812] mode=indexing
          tunnel: "Start Value" -> [w2810] mode=indexing
          i -> [w2813]
          n1083 = Bundle By Name(cluster=T5 {"Pin"="Pin A", "MODE"="", "TARGET VALUE"=0.0, "RAMP RATE"=0.0, "COMPLIANCE LIMIT"=0.0, "START DELAY"=0.0, "Source Mode"=0, "RELATIVE TO"=enum."Power sequence start", "DEFAULT RAMP RATE"=FALSE, "SENSE MODE"=0, "Sense Mode Frame"="", "TRANSIENT RESPONSE"=0, "Transient Reponse Frame"="", "START VALUE"=0.0} ("Pin Config"), "START VALUE"=w2810, "RELATIVE TO"=w2811, "TRANSIENT RESPONSE"=w2812, "SENSE MODE"=w2814, "DEFAULT RAMP RATE"=w2815, "RAMP RATE"=w2825, "COMPLIANCE LIMIT"=w2824, "START DELAY"=w2823, "Source Mode"=w2822, "TARGET VALUE"=w2821, "Pin"=w2816) -> (w2820:T5)
          n1084 = Index Array(array=w2818, index=w2813) -> (element=w2817:T5)
          n1085 = Not Equal?(x=w2817, y=w2820) -> (x != y?=w2819:bool)
        }
        n1086 = Array Size(array=w2797) -> (size(s)=w2788:i32)
        n1087 = Array Size(array="Start Value") -> (size(s)=w2789:i32)
        n1088 = Not Equal?(x=w2788, y=w2789) -> (x != y?=w2795:bool)
        n1089 = Build Array (concatenate)(w2795, w2798) -> (w2796:bool[])
        n1090 = Less Or Equal?(x=w2788, y=w2789) -> (x <= y?=w2787:bool)
        n1091 = Or Array Elements(Boolean array=w2796) -> (logical OR=w2799:bool)
        n1092 = Bundle By Name(cluster=w2804, "Flags.Same Size?"=w2787, "Flags.Changes?"=w2799, "Pin Config.Source Pin Config"=w2800, "Pins"="Pin Name") -> (w2805:T14)
      }
      frame "Check for Changes - 2" {
        # "Check for changes in Advanced Settings configuration"
        n1093 = Unbundle By Name(w2831) -> ("Adv Settings.Adv Setting.Power line frequency"=w2835:T11, "Adv Settings.Adv Setting.Data Capture"=w2834:bool)
        n1094 = Not Equal?(x="Power line frequency", y=w2835) -> (x != y?=w2833:bool)
        n1095 = Not Equal?(x=w2834, y="Data Capture") -> (x != y?=w2832:bool)
        n1096 = Or(x=w2833, y=w2832) -> (x .or. y?=w2829:bool)
        n1097 = Bundle By Name(cluster=w2831, "Adv Settings.Adv Setting.Power line frequency"="Power line frequency", "Flags.Adv Settings Change?"=w2829, "Adv Settings.Adv Setting.Data Capture"="Data Capture") -> (w2830:T14)
      }
      frame "Restore Formatting" {
        n1098 = Unbundle By Name(w2840) -> ("Flags.Changes?"=w2839:bool, "Flags.Same Size?"=w2838:bool)
        n1099 = case shown="True" w2839 {
          tunnel: [_ w2846] -> w2837
          tunnel: w2838 -> [_ w2845]
          frame False {
            # "no changes"
          }
          frame True {
            n1100 = Select(t=string[] ["Set Parameters"], s=w2845, f=string[] ["Restore Cell Font Color", "Set Parameters"]) -> (s? t:f=w2846:string[])
          }
        }
        n1101 = for {
          shift-right: [w2851] -> w2841
          shift-left: w2843 -> [w2852]
          tunnel: w2842 -> [w2850]
          tunnel: w2837 -> [w2849] mode=indexing
          n1102 = Enqueue Element(queue=w2850, element=w2849, timeout in ms (-1)=50, error in (no error)=w2852) -> (error out=w2851:errorcluster)  [unwired: 2 out]
        }
      }
      frame "Re-shuffle Plot Colors" {
        # "#coercion dot"
        # "Rearrange reference colors"
        n1103 = Unbundle By Name(w2859) -> ("Pin Config.Color Array"=w2856:T3, "Plot Colors"=w2858:u32[], "Pin Config.Color Array"=w2854:T3)
        n1104 = for {
          tunnel: w2854 -> [w2864]
          tunnel: w2858 -> [w2861] mode=indexing
          tunnel: [w2861] -> w2853 mode=indexing if=w2862
          n1105 = Search 1D Array(1D array=w2864, element=w2861) -> (index of element=w2863:i32)  [unwired: 1 in]
          n1106 = Less Than 0?(x=w2863) -> (x < 0?=w2862:bool)
        }
        n1107 = Build Array (concatenate)(w2856, w2853) -> (w2855:T3)
        n1108 = Bundle By Name(cluster=w2859, "Plot Colors"=w2855) -> (w2857:T14)
      }
      frame "Generate Plot Colors" {
        # "true-color exists\nfalse-generate color"
        # "Generate plot colors in case UI config and results are being updated from TS layer"
        n1109 = Unbundle By Name(w2867) -> ("Flags.Changes?"=w2865:bool, "Legend.Current (A)"=w2868:T13[], "Pin Config.Source Pin Config"=w2871:T5[], "Legend.Voltage (V)"=w2872:T13[], "Pin Config.Color Array"=w2874:T3, "Pin Config.Source Pin Config"=w2876:T5[], "Pin Config.Color Array"=w2879:T3, "Plot Colors"=w2873:u32[])
        n1110 = Array Size(array=w2879) -> (size(s)=w2875:i32)
        n1111 = Array Size(array=w2876) -> (size(s)=w2878:i32)
        n1112 = Not Equal?(x=w2878, y=w2875) -> (x != y?=w2877:bool)
        n1113 = case shown="False" w2877 {
          tunnel: w2875 -> [_ w2913]
          tunnel: w2874 -> [_ w2914]
          tunnel: w2873 -> [_ w2912]
          tunnel: w2872 -> [w2881 w2911]
          tunnel: w2871 -> [w2882 w2908]
          tunnel: w2870 -> [w2888 w2910]
          tunnel: [w2888 w2909] -> w2869
          tunnel: w2868 -> [w2884 w2907]
          tunnel: w2867 -> [w2887 w2906]
          tunnel: [w2886 w2902] -> w2866
          tunnel: w2865 -> [w2885 _]
          frame False {
            n1114 = case shown="False" w2885 {
              tunnel: w2884 -> [w2890 w2895]
              tunnel: [w2890 w2894] -> w2883
              tunnel: w2882 -> [_ w2893]
              tunnel: w2881 -> [w2889 w2892]
              tunnel: [w2889 w2891] -> w2880
              frame False {
                # "No changes - nothing to do"
              }
              frame True {
                # "Sizes are same but pin config changed - so only updating pin names is enough"
                n1115 = for {
                  tunnel: w2895 -> [w2901] mode=indexing
                  tunnel: [w2900] -> w2894 mode=indexing
                  tunnel: w2893 -> [w2899] mode=indexing
                  tunnel: w2892 -> [w2898] mode=indexing
                  tunnel: [w2896] -> w2891 mode=indexing
                  # "for each pin sequence"
                  n1116 = Unbundle By Name(w2899) -> ("Pin"=w2897:string)
                  n1117 = Bundle By Name(cluster=w2901, "Name"=w2897) -> (w2900:T13)
                  n1118 = Bundle By Name(cluster=w2898, "Name"=w2897) -> (w2896:T13)
                }
              }
            }
            n1119 = Bundle By Name(cluster=w2887, "Legend.Current (A)"=w2883, "Legend.Voltage (V)"=w2880) -> (w2886:T14)
          }
          frame True {
            # "True - color exists so pick the existing color, visibility value and plot name\nFalse - pick new color from reference of colors, visibility as True and plot name from pin config"
            # "#coercion dot"
            # "differences exist - so generate colors"
            n1120 = for {
              tunnel: w2914 -> [w2937]
              tunnel: w2913 -> [w2938]
              tunnel: w2912 -> [w2935]
              tunnel: [w2933] -> w2903 mode=indexing
              tunnel: w2911 -> [w2919]
              tunnel: [w2925] -> w2904 mode=indexing
              shift-right: [w2932] -> w2909
              shift-left: w2910 -> [w2932]
              tunnel: w2908 -> [w2931] mode=indexing
              tunnel: w2907 -> [w2917]
              tunnel: [w2920] -> w2905 mode=indexing
              i -> [w2915]
              # "for each pin in sequence"
              n1121 = Index Array(array=w2917, index=w2915) -> (element=w2916:T13)
              n1122 = Index Array(array=w2919, index=w2915) -> (element=w2918:T13)
              n1123 = Greater?(x=w2938, y=w2915) -> (0:w2923:bool)
              n1124 = Index Array(array=w2935, index=w2915) -> (element=w2934:u32)
              n1125 = Index Array(array=w2937, index=w2915) -> (element=w2936:u32)
              n1126 = Unbundle By Name(w2916) -> ("Visible"=w2922:bool)
              n1127 = Unbundle By Name(w2918) -> ("Visible"=w2929:bool)
              n1128 = Unbundle By Name(w2931) -> ("Pin"=w2930:string)
              n1129 = Select(t=w2936, s=w2923, f=w2934) -> (s? t:f=w2933:u32)
              n1130 = Select(t=w2922, s=w2923, f=TRUE) -> (s? t:f=w2921:bool)
              n1131 = Select(t=w2929, s=w2923, f=TRUE) -> (s? t:f=w2926:bool)
              n1132 = Bundle By Name(cluster=T13 {"Color"=0, "Name"="Pin", "Visible"=FALSE} ("Plot"), "Name"=w2930, "Visible"=w2926, "Color"=w2933) -> (w2925:T13)
              n1133 = Bundle By Name(cluster=w2925, "Visible"=w2921) -> (w2920:T13)
            }
            n1134 = Bundle By Name(cluster=w2906, "Legend.Current (A)"=w2905, "Legend.Voltage (V)"=w2904, "Pin Config.Color Array"=w2903) -> (w2902:T14)
          }
        }
      }
      frame "Set Parameters" {
        w2943 = string[] [] ("List Specs.UI Pin List")
        n1135 = Unbundle By Name(w2952) -> ("Pin Config.Source Pin Config"=w2939:T5[], "Indices.Selected Row"=w2948:i32, "Indices.Actual Sel Row"=w2949:i32, "Indices.Actual Sel Row"=w2950:i32, "Flags.Same Size?"=w2945:bool)
        n1136 = case shown="True" w2945 {
          tunnel: w2949 -> [_ w2964]
          tunnel: w2948 -> [_ w2965]
          tunnel: [w2958 w2963] -> w2947
          tunnel: [w2958 w2962] -> w2946
          tunnel: [w2959 w2962] -> w2944
          tunnel: w2950 -> [_ _]
          tunnel: w2939 -> [w2961 _]
          frame False {
            # "load last pin config in seq"
            n1137 = Array Size(array=w2961) -> (size(s)=w2960:i32)
            n1138 = Decrement(x=w2960) -> (x-1=w2959:i32)
            n1139 = expression code="x*2"(w2959) -> (w2958:i32)
          }
          frame True {
            # "load previosuly selected pin config"
            n1140 = expression code="x<0?0:x"(w2964) -> (w2962:i32)
            n1141 = expression code="x<0?0:x"(w2965) -> (w2963:i32)
          }
        }
        n1142 = for {
          shift-right: [w2969] -> w2953
          shift-left: w2955 -> [w2970]
          tunnel: w2954 -> [w2968]
          tunnel: string[] ["Read Pin List", "Format Pin List", "Check Pin List Scrollbar", "Update UI", "Update Plot Legend", "Get Mouse Down Row Info", "Update Plot Visibility"] -> [w2967] mode=indexing
          n1143 = Enqueue Element(queue=w2968, element=w2967, timeout in ms (-1)=50, error in (no error)=w2970) -> (error out=w2969:errorcluster)  [unwired: 2 out]
        }
        n1144 = Bundle By Name(cluster=w2952, "Indices.Top Row"=u32 0, "Pin Config.Error Ind"=i32[] [] ("Pin Config.Error Codes"), "Indices.Row No Ref"=u32 0, "List Specs.UI Pin List"=w2943, "List Specs.Pin List"=w2943, "Pin Config.Error Info"=w2943, "Indices.Selected Row"=w2947, "Indices.Active Row"=w2946, "Indices.Actual Sel Row"=w2944, "Flags.Check All?"=TRUE) -> (w2957:T14)
      }
      frame "--- Continuous Monitoring Operations ---" {
      }
      frame "Check UI Resize?" {
        # "During screen resize - hide plot legend, info image, power down info image and pin selection list of visible"
        # "Monitor Voltage graph size to know if screen is being resized"
        n1145 = Unbundle By Name(w2989) -> ("Coords.Graph Size"=w2981:cluster{"Width":u32, "Height":u32}, "Flags.Visibilty.Plot Legend"=w2976:bool, "Flags.Visibilty.Help?"=w2974:bool, "Flags.Visibilty.PD Info"=w2973:bool)
        n1146 = property on="Voltage" class="WFGraph (strict)"(error in=w2986) -> (error out=w2985:errorcluster, "Width"=w2982:u32, "Height"=w2983:u32)  [unwired: 1 in, 1 out]
        n1147 = Bundle(cluster=cluster{"Width":u32, "Height":u32} {"Width"=0, "Height"=0} ("Coords.Graph Size"), "Width"=w2982, "Height"=w2983) -> (w2977:cluster{"Width":u32, "Height":u32})
        n1148 = Not Equal?(x=w2981, y=w2977) -> (x != y?=w2980:bool)
        n1149 = case shown="True" w2980 {
          tunnel: w2988 -> [_ w3001]
          tunnel: w2985 -> [w2991 w3002]
          tunnel: [w2991 w3000] -> w2987
          tunnel: string[] ["Get Icons Coords - 1", "Get Icons Coords - 2", "Get Icons Coords - 3", "Reset Graph Scales", "Hide Listbox"] -> [_ w2999]
          tunnel: w2976 -> [w2990 w2996]
          tunnel: [w2990 FALSE ("Plot Legend")] -> w2975
          tunnel: w2974 -> [_ w2995]
          tunnel: w2973 -> [_ w2992]
          frame False {
            # "none"
          }
          frame True {
            # "screen resizing on - calculate all necessary controls' dimensions again"
            n1150 = Build Array(w2996, w2995, w2992) -> (w2994:bool[])
            n1151 = for {
              tunnel: [w3004] -> w2993 mode=concatenating if=w3003
              tunnel: w2994 -> [w3003] mode=indexing
              i -> [w3005]
              n1152 = case shown="0, Default" w3005 {
                tunnel: [string[] ["Show/Hide Legend"] string[] ["Hide Image", "Update Icon State"] string[] ["Hide Power Down Image", "Update Icon State"]] -> w3004
                frame 0, Default {
                  # "Plot Legend"
                }
                frame 1 {
                  # "Info Image"
                }
                frame 2 {
                  # "Power Down Info Image"
                }
              }
            }
            n1153 = Build Array (concatenate)(w2999, w2993) -> (w2998:string[])
            n1154 = for {
              shift-right: [w3012] -> w3000
              shift-left: w3002 -> [w3013]
              tunnel: w3001 -> [w3011]
              tunnel: w2998 -> [w3010] mode=indexing
              n1155 = Enqueue Element(queue=w3011, element=w3010, timeout in ms (-1)=50, error in (no error)=w3013) -> (error out=w3012:errorcluster)  [unwired: 2 out]
            }
          }
        }
        n1156 = Bundle By Name(cluster=w2989, "Coords.Graph Size"=w2977, "Flags.Visibilty.Plot Legend"=w2975) -> (w2978:T14)
      }
      frame "Get Pinmap List" {
        # "Read list of pins from pinmap file"
        n1157 = Unbundle By Name(w3028) -> ("Pinmap List"=w3016:string[])
        n1158 = property on="Pin Name" class="CmbBox"(error in=w3029) -> (error out=w3025:errorcluster, "Strings[]"=w3019:string[])  [unwired: 1 in, 1 out]
        n1159 = Not Equal?(x=w3016, y=w3019) -> (x != y?=w3027:bool)
        n1160 = Empty Array?(array=w3019) -> (empty?=w3026:bool)
        n1161 = Array Size(array=w3019) -> (size(s)=w3021:i32)
        n1162 = Array Size(array=w3016) -> (size(s)=w3022:i32)
        n1163 = Not Equal?(x=w3022, y=w3021) -> (x != y?=w3020:bool)
        n1164 = Compound Arithmetic op=AND(w3020, w3027, invert w3026) -> (w3015:bool)
        n1165 = Select(t=w3019, s=w3015, f=w3016) -> (s? t:f=w3014:string[])
        n1166 = case shown="True" w3015 {
          tunnel: w3028 -> [w3031 w3055]
          tunnel: w3025 -> [w3030 w3049]
          tunnel: [w3030 w3054] -> w3024
          tunnel: [w3031 w3053] -> w3023
          tunnel: w3014 -> [_ w3042]
          tunnel: w3018 -> [_ w3044]
          tunnel: string[] ["Validate Inputs", "Update Error Info", "Update Error Display Top Row", "Update Error Display Scrollbar", "Check for Plot Name Autofit"] -> [_ w3043]
          frame False {
            # "no changes made"
          }
          frame True {
            # "invalid pin names will be still there in the \nlist in the format 'Pin Name [!]'\nSo consider only valid pin names"
            # "Pinmap list changed - so update UI"
            n1167 = for {
              tunnel: w3044 -> [w3058]
              shift-right: [w3059] -> w3045
              shift-left: w3049 -> [w3060]
              tunnel: w3043 -> [w3057] mode=indexing
              n1168 = Enqueue Element(queue=w3058, element=w3057, timeout in ms (-1)=50, error in (no error)=w3060) -> (error out=w3059:errorcluster)  [unwired: 2 out]
            }
            n1169 = for {
              tunnel: w3042 -> [w3061] mode=indexing
              tunnel: [w3061] -> w3036 mode=indexing if=w3062
              shift-right: [w3068] -> w3048
              shift-left: w3045 -> [w3068]
              tunnel: w3042 -> [w3066] mode=indexing
              tunnel: [w3064] -> w3041 mode=indexing if=w3062
              tunnel: [w3063] -> w3039 mode=indexing if=w3062
              n1170 = Match Pattern(string=w3066, regular expression=" \\[!\\]") -> (before substring=w3064:string, offset past match=w3065:i32)  [unwired: 1 in, 2 out]
              n1171 = Less Than 0?(x=w3065) -> (x < 0?=w3062:bool)
              n1172 = String Length(string=w3064) -> (length=w3063:i32)
            }
            n1173 = Array Size(array=w3036) -> (size(s)=w3033:i32)
            n1174 = expression code="x<=7 ? x : 7"(w3033) -> (w3047:i32)
            n1175 = Greater?(x=w3033, y=7) -> (0:w3050:bool)
            n1176 = Initialize Array(0, w3033) -> (w3032:i32[])
            n1177 = To Unsigned Long Integer(number=w3047) -> (unsigned 32bit integer=w3035:u32)
            n1178 = Array Max & Min(array=w3039) -> (max value=w3038:i32, max index (indices)=w3037:i32)  [unwired: 2 out]
            n1179 = property on="Pin Selection" class="LstBox (strict)"(error in=w3048, "Item Names"=w3036, "Number of Rows"=w3035, "Scrollbar Visible"=w3050) -> (error out=w3054:errorcluster, "Height"=w3052:u32)  [unwired: 1 in, 1 out]
            n1180 = To Long Integer(number=w3052) -> (32bit integer=w3046:i32)
            n1181 = Bundle By Name(cluster=w3055, "Flags.Check All?"=TRUE, "Indices.Pin Len new"=w3038, "Indices.Pin Len Ind"=w3037, "Pinmap List"=w3041, "Pin Selection.Dimensions.Height"=w3046, "Pin Symbols"=w3032) -> (w3053:T14)
          }
        }
      }
      frame "Check for Plot Name Autofit" {
        # "old - contains the max length of pin name in old pinmap list\nnew - contains the max length of pin name in the updated pinmap list"
        # "When pinmap list is updated check if max. pin name length changed"
        n1182 = Unbundle By Name(w3076) -> ("Indices.Pin Len \nold"=w3075:i32, "Indices.Pin Len new"=w3074:i32)
        n1183 = Not Equal?(x=w3075, y=w3074) -> (x != y?=w3069:bool)
        n1184 = case shown="True" w3069 {
          tunnel: w3073 -> [w3077 w3081]
          tunnel: w3072 -> [_ w3080]
          tunnel: [w3077 w3079] -> w3071
          tunnel: string[] ["Auto fit Plot Name Control", "Update Plot Legend"] -> [_ w3078]
          frame False {
          }
          frame True {
            n1185 = for {
              tunnel: w3080 -> [w3084]
              shift-right: [w3085] -> w3079
              shift-left: w3081 -> [w3086]
              tunnel: w3078 -> [w3083] mode=indexing
              n1186 = Enqueue Element(queue=w3084, element=w3083, timeout in ms (-1)=50, error in (no error)=w3086) -> (error out=w3085:errorcluster)  [unwired: 2 out]
            }
          }
        }
      }
      frame "Auto fit Plot Name Control" {
        # "objective - to autosize plot name control in plot legend to fit the maximum pin name in pinmap list"
        # "pin name length changed - run the algorithm to determine the exact width of plot name control in 'Legend'"
        n1187 = Unbundle By Name(w3101) -> ("Indices.Pin Len new"=w3097:i32, "Pinmap List"=w3095:string[], "Indices.Pin Len Ind"=w3094:i32)
        n1188 = Index Array(array=w3095, index=w3094) -> (element=w3093:string)
        n1189 = property on="PN AutoFit" class="Str"(error in=w3105, "Value"=w3093, "WrappingEnabled"=TRUE ("Enable Wrapping")) -> (error out=w3103:errorcluster, "Text.FontSize"=w3096:u32)  [unwired: 1 in, 1 out]
        n1190 = To Unsigned Long Integer(number=w3097) -> (unsigned 32bit integer=w3091:u32)
        n1191 = Bundle By Name(cluster=w3101, "Indices.Pin Len \nold"=w3097) -> (w3099:T14)
        n1192 = Multiply(x=w3091, y=w3096) -> (x*y=w3104:u32)
        n1193 = while {
          shift-right: [w3114] -> w3100
          shift-left: w3104 -> [w3113]
          tunnel: w3103 -> [w3112]
          tunnel: [w3106] -> w3090
          shift-right: [w3110] -> _
          shift-left: "Start" -> [w3111]
          shift-right: [w3109] -> _
          shift-left: _ -> [w3107]
          stop <- w3108 stop-if-true
          n1194 = case shown="\"Start\"" w3111 {
            selector: w3111 -> [_ w3121 w3139 _]
            tunnel: [_ w3117 w3132 w3146] -> w3114
            tunnel: w3113 -> [_ w3125 w3133 w3145]
            tunnel: w3112 -> [w3116 w3124 w3141 w3150]
            tunnel: [w3116 w3123 w3140 w3149] -> w3106
            tunnel: [_ w3120 w3139 "Fit" ("f")] -> w3110
            tunnel: [_ u32 0 w3131 w3147] -> w3109
            tunnel: [TRUE _ w3137 _] -> w3108
            tunnel: w3107 -> [_ _ w3138 _]
            frame "False", Default {
            }
            frame "Start" {
              n1195 = Increment(x=w3125) -> (x+1=w3129:u32)
              n1196 = Quotient & Remainder(x=w3129, y=u32 2) -> (floor(x/y)=w3117:u32)  [unwired: 1 out]
              n1197 = property on="PN AutoFit" class="Str"(error in=w3124, "Width"=w3117) -> (error out=w3128:errorcluster)  [unwired: 1 in, 1 out]
              n1198 = invoke on="PN AutoFit" class="Str" method="Get Nth Line"(error in=w3128, "index"=u32 1 ("line index")) -> (error out=w3123:errorcluster, "start"=w3126:u32)  [unwired: 5 in, 5 out]
              n1199 = Equal To 0?(x=w3126) -> (x = 0?=w3122:bool)
              n1200 = Select(t=w3121, s=w3122, f="Find") -> (s? t:f=w3120:string)
            }
            frame "Fit" {
              n1201 = Subtract(x=w3133, y=w3138) -> (x-y=w3134:u32)
              n1202 = property on="PN AutoFit" class="Str"(error in=w3141, "Width"=w3134) -> (error out=w3143:errorcluster)  [unwired: 1 in, 1 out]
              n1203 = Quotient & Remainder(x=w3138, y=u32 2) -> (floor(x/y)=w3131:u32)  [unwired: 1 out]
              n1204 = invoke on="PN AutoFit" class="Str" method="Get Nth Line"(error in=w3143, "index"=u32 1 ("line index")) -> (error out=w3140:errorcluster, "start"=w3136:u32)  [unwired: 5 in, 5 out]
              n1205 = Equal To 0?(x=w3131) -> (x = 0?=w3137:bool)
              n1206 = Equal To 0?(x=w3136) -> (x = 0?=w3135:bool)
              n1207 = Select(t=w3134, s=w3135, f=w3133) -> (s? t:f=w3132:u32)
            }
            frame "Find" {
              n1208 = while {
                shift-right: [w3156] -> _
                shift-left: w3145 -> [w3158]
                shift-right: [w3154] -> w3147
                shift-left: 1 -> [w3153]
                shift-right: [w3152] -> w3149
                shift-left: w3150 -> [w3152]
                stop <- w3155 stop-if-true
                n1209 = Quotient & Remainder(x=w3158, y=u32 2) -> (floor(x/y)=w3156:u32)  [unwired: 1 out]
                n1210 = Add(x=w3153, y=w3153) -> (x+y=w3154:i32)
                n1211 = Equal To 0?(x=w3156) -> (x = 0?=w3155:bool)
              }
              n1212 = expression code="x*2"(w3145) -> (w3146:u32)
            }
          }
        }
        n1213 = Bundle(cluster=w3090, "status"=FALSE) -> (w3088:errorcluster)  [unwired: 2 in]
        n1214 = property on="Name" class="Str"(error in=w3088, "Width"=w3100) -> (error out=w3087:errorcluster)  [unwired: 1 in, 1 out]
        n1215 = property on="Name" class="Str"(error in=w3087, "Width"=w3100) -> ()  [unwired: 1 in, 2 out]
      }
      frame "Monitor ML Controls State" {
        # "index 8 - Power Down - should always be disabled state"
        # "Disable controls during execution and enable post execution"
        n1216 = Unbundle By Name(w3163) -> ("All Refs"=w3166:refnum<vi>[], "Flags.UI State"=w3160:T20)
        n1217 = property on="Pin Name" class="Arr (strict)"(error in=w3169) -> (error out=w3168:errorcluster, "DisabledEnum"=w3162:T20)  [unwired: 1 in, 1 out]
        n1218 = Not Equal?(x=w3160, y=w3162) -> (x != y?=w3159:bool)
        n1219 = Delete From Array(array=w3166, index=8) -> (array with subset deleted=w3165:refnum<vi>[])  [unwired: 1 in, 1 out]
        n1220 = case shown="True" w3159 {
          tunnel: w3168 -> [w3170 w3175]
          tunnel: [w3170 w3174] -> w3167
          tunnel: w3165 -> [_ w3173]
          tunnel: w3162 -> [_ w3172]
          frame False {
          }
          frame True {
            n1221 = for {
              tunnel: w3175 -> [w3179]
              tunnel: w3173 -> [w3178] mode=indexing
              tunnel: w3172 -> [w3177]
              tunnel: [w3176] -> w3171 mode=indexing
              # "for each control on UI"
              n1222 = property on="Property Node" class="Ctl"(reference=w3178, error in=w3179, "DisabledEnum"=w3177) -> (error out=w3176:errorcluster)  [unwired: 1 out]
            }
            n1223 = Merge Errors(w3171) -> (w3174:errorcluster)
          }
        }
        n1224 = Bundle By Name(cluster=w3163, "Flags.UI State"=w3162) -> (w3161:T14)
      }
      frame "Monitor Icons" {
        # "index 8 - Power Down - should always be disabled state"
        # "Hide Power Down image, pin selection listbox, Relative To image and plot legend if visible when ML events are triggered (Run, Paste)"
        n1225 = Unbundle By Name(w3192) -> ("Flags.Visibilty.Plot Legend"=w3188:bool, "Flags.Visibilty.Help?"=w3187:bool, "Flags.Visibilty.PD Info"=w3186:bool)
        n1226 = Bundle By Name(cluster=w3192, "Flags.Visibilty.Plot Legend"=FALSE) -> (w3190:T14)
        n1227 = Build Array(w3188, w3187, w3186) -> (w3185:bool[])
        n1228 = for {
          tunnel: [w3199] -> w3184 mode=concatenating if=w3198
          tunnel: w3185 -> [w3198] mode=indexing
          i -> [w3200]
          n1229 = case shown="0, Default" w3200 {
            tunnel: [string[] ["Show/Hide Legend"] string[] ["Hide Image", "Update Icon State"] string[] ["Hide Power Down Image", "Update Icon State"]] -> w3199
            frame 0, Default {
              # "Plot Legend"
            }
            frame 1 {
              # "Info Image"
            }
            frame 2 {
              # "Power Down Info Image"
            }
          }
        }
        n1230 = Build Array (concatenate)("Hide Listbox" ("element"), w3184) -> (w3183:string[])
        n1231 = for {
          shift-right: [w3196] -> w3191
          shift-left: w3181 -> [w3197]
          tunnel: w3189 -> [w3195]
          tunnel: w3183 -> [w3194] mode=indexing
          n1232 = Enqueue Element(queue=w3195, element=w3194, timeout in ms (-1)=50, error in (no error)=w3197) -> (error out=w3196:errorcluster)  [unwired: 2 out]
        }
      }
      frame "--- Error Handling Operations ---" {
      }
      frame "Handle Error" {
        w3206 = errorcluster {"status"=FALSE, "code"=0, "source"=""}  # No Error
      }
      frame "--- Exit Operations ---" {
      }
      frame "Exit" {
        # "This case is triggered to close the User Interface from framework"
        n1233 = Flush Queue(queue=w3215, error in (no error)=w3217) -> (queue out=w3214:refnum<queue>, error out=w3213:errorcluster)  [unwired: 1 out]
        n1234 = Release Queue(queue=w3214, force destroy? (F)=TRUE, error in (no error)=w3213) -> (error out=w3212:errorcluster)  [unwired: 2 out]
      }
    }
  }
  n1235 = property on="Voltage Measurements" class="Arr (strict)" props=["DisabledEnum"]() -> ()  [unwired: 2 in, 3 out]
